vi "RealTimeSingle.vi"(0 "Digitizer Settings":T30={"Digitizer delay (us) "=0.0, "rf points per line"=2048, "lines per plane"=128, "Samp Rate (Hz)"=100000000.0, "Additional dig delay (us)"=0.0, "Voltage Scale"=0.4, "Pre-Looks"=0, "Offset delay (us)"=0.0, "bits A/D"=8, "Avg Num"=1, "DigTimeOut"=5.0, "Rel Dig Delay"=0.0, "Dig Ch"=0, "LeCroyCluster"={"LeCroy Channels"=[TRUE, FALSE, FALSE, FALSE], "LC read pt offset"=0.0, "Sweep Avg"=FALSE}, "Main Digitizer"=enum."NI Digitizer", "Dig Config"=enum."Single channel", "Digitizer ID Cluster"={"Acqiris/Alazar/SP ID"=[], "NI Instr Handles"=[], "LeCroy VISA"="", "GaGe Handle"={"Handle"=0, "Sample size"=0, "Resolution"=0, "Offset"=0, "Channels"=0, "Boards"=0}, "ATS Ref"="ATS9350", "Acqiris Address"=["PCI::INSTR0"], "ADQRef"=refnum, "adq_cu_ptr"=refnum}, "Trigger Settings"={"Trig Source"=1, "Trig Coupling"=0, "Trig Slope"=0, "Level (mV)"=1500.0}, "Bulk Acq"=FALSE, "Bulk Start Indexes"=[], "Data Ref RF"=refnum, "NI ID/Channel"=[], "Total Dig CH"=1, "Xtra Ann Trig delay (us)"=10.0, "Fix Z Delay?"=FALSE, "One Way Transmission?"=FALSE, "Data Ref Log"=refnum} {"Trigger Settings"."Trig Slope" items=["Positive", "Negative"]; "Trigger Settings"."Level (mV)" format="%.2f"; "Trigger Settings"."Trig Coupling" items=["DC 1 MOhm", "AC 1 MOhm", "DC 50 Ohm", "AC 50 Ohm"]; "Trigger Settings"."Trig Source" items=["Chan 1", "External"]; "Rel Dig Delay" format="%.2f"; "DigTimeOut" format="%.2f"; "Avg Num" min=1; "Offset delay (us)" format="%.2f"; "Additional dig delay (us)" format="%.2f"; "Digitizer delay (us)" format="%.2f"}, 1 "File Name":string="Case", 4 "Motion Settings":T26={"No Motion?"=FALSE, "Motion System"=enum."NI 735x", "Motion Bd ID"=1, "Motion Profile"="SMAC1", "# Axis"=1, "Reverse Z axis?"=TRUE, "SMAC Axis"=0, "scan pair"=enum."y-(x) scan", "RT fps"=6.0, "Steps per mm"=[1000, 1000, 1000, 1000], "Motor Parameters"={"velocity ct/s"=[10000.0, 10000.0, 10000.0, 50000.0], "accel ct/s^2"=[50000.0, 50000.0, 50000.0, 200000.0]}, "One Way Scan"=FALSE, "Reverse One Way Scan"=FALSE, "Global Position (mm)"=[], "Plane"=0, "Distance between\nscan lines (um)"=0.0, "Distance between\nscan planes (um)"=0.0, "number of scan planes"=1, "Total steps in line"=0, "Xtra plane\ndistance  (um)"=100, "Xtra planes "=1, "Add Axis"=FALSE, "overshoot cts"=200, "BKPT Shift"=0, "Scan Start Time (ms)"=0, "ESP VISA"="GPIB::1::INSTR", "3rd Axis"=1, "GL Ref Out"=refnum, "Galil Address"=""} {"3rd Axis" items=["x", "y", "z", "w"]; "Xtra planes" min=1; "Xtra plane\ndistance  (um)" min=0; "Distance between\nscan planes (um)" format="%.2f"; "Distance between\nscan lines (um)" format="%.2f"; "SMAC Axis" items=["None"=0, "Axis 1"=1, "Axis 2"=2, "Axis 3"=3, "Axis 4"=4, "Axis 5"=5, "Axis 6"=6, "Axis 7"=7, "Axis 8"=8, "Vector Space 1"=17, "Vector Space 2"=18, "Vector Space 3"=19, "Vector Space 4"=20]; "Motion Bd ID" min=1 max=32 step=1}, 5 "Type of scan":T21=enum."1-D B Scan", 6 "Ann Array Params":T22={"Synth Foc?"=FALSE, "Focal Zones"=41, "Switch T/R"=0, "Trans Geometry (mm)"={"Transducer"=0, "Geo Focus"=12.0, "a (radius)"=3.0, "# of rings"=5, "kerf space "=0.1, "Center Freq"=12.0}, "Sub Ap Excite?"=FALSE, "Full Array Scan?"=FALSE, "Xmt/Rcv"={"XMIT"=[TRUE, TRUE, TRUE, TRUE, TRUE], "RCV"=[TRUE, TRUE, TRUE, TRUE, TRUE]}, "PulseSpacing (us)"=0.0, "Xmit Ring"=0, "XMIT CHS"=0, "RCV CHS"=0, "GPU?"=FALSE, "Save TIFF?"=FALSE, "downfactor"=1, "RCV 1CH"=0} {"RCV 1CH" items=["All", "1", "2", "3", "4", "5"]; "Trans Geometry (mm)"."Transducer" items=["6D 12R 40 MHz"=0, "10D 31R 20 MHz"=1, "10D 23R 20 MHz"=2, "6D 23R 40 MHz"=3, "4.5D 10.7R 40 MHz"=4, "9D 23.5R 20 MHz"=5, "9D 25.8R 20MHz"=6, "Enter"=99]; "Switch T/R" min=1 max=5 step=1}, 7 "return to start":bool, 9 "Dual XDCR Settings":T1 {"XDCR Settings"."UT340 Controls"."Low Pass Filter (MHz)" min=-6 max=60 step=1; "XDCR Settings"."UT340 Controls"."High Pass Filter (MHz)" min=1 max=20 step=1; "XDCR Settings"."UT340 Controls"."Rep Rate (Hz)" min=20 step=1; "XDCR Settings"."UT340 Controls"."Pulse Width (ns)" min=100.0 max=250.0 step=2.0; "XDCR Settings"."UT340 Controls"."Voltage" min=100 max=250 step=2; "XDCR Settings"."UT340 Controls"."PC Gain (dB)" min=2 max=72; "XDCR Settings"."UT340 Controls"."PE Gain (dB)" min=-6 max=60 step=1; "XDCR Settings"."JSR Complete"."JSR Trigger Settings"."PRF (Hz)" items=["100 Hz"=0.1, "200 Hz"=0.2, "400 Hz"=0.4, "600 Hz"=0.6, "800 Hz"=0.8, "1000 Hz"=1.0, "1250 Hz"=1.25, "1500 Hz"=1.5, "1750 Hz"=1.75, "2000 Hz"=2.0, "2500 Hz"=2.5, "3000 Hz"=3.0, "3500 Hz"=3.5, "4000 Hz"=4.0, "4500 Hz"=4.5, "5000 Hz"=5.0]; "XDCR Settings"."JSR Complete"."JSR Trigger Settings"."Trigger Source" items=["Internal", "External"]; "XDCR Settings"."JSR Complete"."JSR Trigger Settings"."External Trigger Limit" items=["No Limit", "5 kHz"]; "XDCR Settings"."JSR Complete"."JSR Receive Settings"."Gain (dB)" min=-13 max=66 step=1; "XDCR Settings"."JSR Complete"."JSR Receive Settings"."Low Pass Filter" items=["5 MHz"=5, "10 MHz"=10, "15 MHz"=15, "22.5 MHz"=22, "35 MHz"=35, "50 MHz"=50]; "XDCR Settings"."JSR Complete"."JSR Receive Settings"."High Pass Filter" items=["DC"=0, "1 MHz"=1000, "2.5 MHz"=2500, "5 MHz"=5000, "7.5 MHz"=7500, "12.5 MHz"=12500]; "XDCR Settings"."JSR Complete"."JSR Receive Settings"."Receiver Mode" items=["Echo", "Through"]; "XDCR Settings"."JSR Complete"."JSR Pulse Settings"."Pulser Voltage (V)" items=["100"=100, "125"=125, "150"=150, "175"=175, "200"=200, "225"=225, "250"=250, "275"=275, "300"=300, "325"=325, "350"=350, "375"=375, "400"=400, "425"=425, "450"=450, "475"=475]; "XDCR Settings"."JSR Complete"."JSR Pulse Settings"."Pulser Impedance" items=["High z", "Low z"]; "XDCR Settings"."JSR Complete"."JSR Pulse Settings"."Pulse Energy Level" items=["0 (Minimum)", "1", "2", "3 (Maximum)"]; "XDCR Settings"."JSR Complete"."JSR Pulse Settings"."Damping" items=["331 Ohms"=331, "198 Ohms"=198, "142 Ohms"=142, "110 Ohms"=110, "92 Ohms"=92, "77 Ohms"=77, "67 Ohms"=67, "59 Ohms"=59, "52 Ohms"=52, "47 Ohms"=47, "43 Ohms"=43, "39 Ohms"=39, "37 Ohms"=37, "34 Ohms"=34, "32 Ohms"=32, "30 Ohms"=30]; "XDCR Settings"."Panametrics Settings"."FINE ATTENUATION" items=["00.0", "00.5", "01.0", "01.5", "02.0", "02.5", "03.0", "03.5", "04.0", "04.5", "05.0", "05.5", "06.0", "06.5", "07.0", "07.5", "08.0", "08.5", "09.0", "09.5", "10.0", "10.5", "11.0", "11.5", "12.0", "12.5", "13.0", "13.5", "14.0", "14.5", "15.0", "15.5"]; "XDCR Settings"."Panametrics Settings"."COARSE ATTENUATION" items=["00.0", "10.0", "20.0", "30.0", "40.0", "50.0"]; "XDCR Settings"."Panametrics Settings"."GAIN (db)" items=["26.0", "40.0", "54.0"]; "XDCR Settings"."Panametrics Settings"."PRF (KHz)" items=["XREMT", "EXBNC", "0.200", "0.500", "1.000", "2.000", "5.000", "10.00", "20.00"]; "XDCR Settings"."Panametrics Settings"."MODE" items=["P/ E", "THRU", "RPP", "EXT_PLSR"]; "XDCR Settings"."Panametrics Settings"."LP FILT (MHz)" items=["20", "50", "100", "200"]; "XDCR Settings"."Panametrics Settings"."HP FILT (KHz)" items=["1", "1000", "3000", "10000"]; "XDCR Settings"."Panametrics Settings"."DAMPING (Ohm)" items=["7", "10", "16", "20", "26", "30", "40", "50"]; "XDCR Settings"."Panametrics Settings"."ENERGY (uJ)" items=["1", "2", "4", "8", "16", "32"]; "XDCR Settings"."Daxsonics Settings"."Freq (MHz)" items=["4"=4, "5"=5, "6"=6, "8"=8, "10"=10, "12"=12, "14"=14, "15"=15, "16"=16, "17"=17, "18"=18, "20"=20, "25"=25, "30"=30, "35"=35, "40"=40, "45"=45, "50"=50]; "XDCR Settings"."Daxsonics Settings"."Voltage (V)" items=["0"=0, "5"=5, "10"=10, "15"=15, "20"=20, "25"=25, "30"=30, "35"=35, "40"=40, "45"=45, "50"=50, "55"=55, "60"=60, "65"=65, "70"=70, "75"=75, "80"=80, "85"=85, "90"=90, "95"=95, "100"=100, "110"=110, "120"=120, "130"=130, "140"=140, "150"=150, "160"=160, "170"=170, "180"=180, "190"=190]; "XDCR Settings"."Daxsonics Settings"."Gain (dB)" items=["22"=22, "25"=25, "28"=28, "31"=31, "34"=34, "37"=37, "40"=40, "43"=43, "46"=46, "49"=49, "52"=52, "55"=55, "58"=58, "61"=61, "64"=64, "67"=67]; "XDCR Settings"."Digitizer Settings"."Additional dig delay (ms)" format="%.2f"; "XDCR Settings"."Digitizer Settings"."Time scale per Div" items=["100 ns"=0.1, "200 ns"=0.2, "500 ns"=0.5, "1 micros"=1.0, "2 micros"=2.0, "5 micros"=5.0, "10 micros"=10.0, "20 micros"=20.0, "50 micros"=50.0, "100 micros"=100.0, "200 micros"=200.0, "500 micros"=500.0, "1 ms"=1000.0, "2 ms"=2000.0, "5 ms"=5000.0, "10 ms"=10000.0, "20 ms"=20000.0, "50 ms"=50000.0, "100 ms"=100000.0, "200 ms"=200000.0]; "XDCR Settings"."Digitizer Settings"."RF data Sampling"."rf points per line" min=1; "XDCR Settings"."Digitizer Settings"."RF data Sampling"."Ref Delay (ms)" format="%.2f"}) -> (11 "Dual XDCR Settings Out":T1 {"XDCR Settings"."UT340 Controls"."Low Pass Filter (MHz)" min=-6 max=60 step=1; "XDCR Settings"."UT340 Controls"."High Pass Filter (MHz)" min=1 max=20 step=1; "XDCR Settings"."UT340 Controls"."Rep Rate (Hz)" min=20 step=1; "XDCR Settings"."UT340 Controls"."Pulse Width (ns)" min=100.0 max=250.0 step=2.0; "XDCR Settings"."UT340 Controls"."Voltage" min=100 max=250 step=2; "XDCR Settings"."UT340 Controls"."PC Gain (dB)" min=2 max=72; "XDCR Settings"."UT340 Controls"."PE Gain (dB)" min=-6 max=60 step=1; "XDCR Settings"."JSR Complete"."JSR Trigger Settings"."PRF (Hz)" items=["100 Hz"=0.1, "200 Hz"=0.2, "400 Hz"=0.4, "600 Hz"=0.6, "800 Hz"=0.8, "1000 Hz"=1.0, "1250 Hz"=1.25, "1500 Hz"=1.5, "1750 Hz"=1.75, "2000 Hz"=2.0, "2500 Hz"=2.5, "3000 Hz"=3.0, "3500 Hz"=3.5, "4000 Hz"=4.0, "4500 Hz"=4.5, "5000 Hz"=5.0]; "XDCR Settings"."JSR Complete"."JSR Trigger Settings"."Trigger Source" items=["Internal", "External"]; "XDCR Settings"."JSR Complete"."JSR Trigger Settings"."External Trigger Limit" items=["No Limit", "5 kHz"]; "XDCR Settings"."JSR Complete"."JSR Receive Settings"."Gain (dB)" min=-13 max=66 step=1; "XDCR Settings"."JSR Complete"."JSR Receive Settings"."Low Pass Filter" items=["5 MHz"=5, "10 MHz"=10, "15 MHz"=15, "22.5 MHz"=22, "35 MHz"=35, "50 MHz"=50]; "XDCR Settings"."JSR Complete"."JSR Receive Settings"."High Pass Filter" items=["DC"=0, "1 MHz"=1000, "2.5 MHz"=2500, "5 MHz"=5000, "7.5 MHz"=7500, "12.5 MHz"=12500]; "XDCR Settings"."JSR Complete"."JSR Receive Settings"."Receiver Mode" items=["Echo", "Through"]; "XDCR Settings"."JSR Complete"."JSR Pulse Settings"."Pulser Voltage (V)" items=["100"=100, "125"=125, "150"=150, "175"=175, "200"=200, "225"=225, "250"=250, "275"=275, "300"=300, "325"=325, "350"=350, "375"=375, "400"=400, "425"=425, "450"=450, "475"=475]; "XDCR Settings"."JSR Complete"."JSR Pulse Settings"."Pulser Impedance" items=["High z", "Low z"]; "XDCR Settings"."JSR Complete"."JSR Pulse Settings"."Pulse Energy Level" items=["0 (Minimum)", "1", "2", "3 (Maximum)"]; "XDCR Settings"."JSR Complete"."JSR Pulse Settings"."Damping" items=["331 Ohms"=331, "198 Ohms"=198, "142 Ohms"=142, "110 Ohms"=110, "92 Ohms"=92, "77 Ohms"=77, "67 Ohms"=67, "59 Ohms"=59, "52 Ohms"=52, "47 Ohms"=47, "43 Ohms"=43, "39 Ohms"=39, "37 Ohms"=37, "34 Ohms"=34, "32 Ohms"=32, "30 Ohms"=30]; "XDCR Settings"."Panametrics Settings"."FINE ATTENUATION" items=["00.0", "00.5", "01.0", "01.5", "02.0", "02.5", "03.0", "03.5", "04.0", "04.5", "05.0", "05.5", "06.0", "06.5", "07.0", "07.5", "08.0", "08.5", "09.0", "09.5", "10.0", "10.5", "11.0", "11.5", "12.0", "12.5", "13.0", "13.5", "14.0", "14.5", "15.0", "15.5"]; "XDCR Settings"."Panametrics Settings"."COARSE ATTENUATION" items=["00.0", "10.0", "20.0", "30.0", "40.0", "50.0"]; "XDCR Settings"."Panametrics Settings"."GAIN (db)" items=["26.0", "40.0", "54.0"]; "XDCR Settings"."Panametrics Settings"."PRF (KHz)" items=["XREMT", "EXBNC", "0.200", "0.500", "1.000", "2.000", "5.000", "10.00", "20.00"]; "XDCR Settings"."Panametrics Settings"."MODE" items=["P/ E", "THRU", "RPP", "EXT_PLSR"]; "XDCR Settings"."Panametrics Settings"."LP FILT (MHz)" items=["20", "50", "100", "200"]; "XDCR Settings"."Panametrics Settings"."HP FILT (KHz)" items=["1", "1000", "3000", "10000"]; "XDCR Settings"."Panametrics Settings"."DAMPING (Ohm)" items=["7", "10", "16", "20", "26", "30", "40", "50"]; "XDCR Settings"."Panametrics Settings"."ENERGY (uJ)" items=["1", "2", "4", "8", "16", "32"]; "XDCR Settings"."Daxsonics Settings"."Freq (MHz)" items=["4"=4, "5"=5, "6"=6, "8"=8, "10"=10, "12"=12, "14"=14, "15"=15, "16"=16, "17"=17, "18"=18, "20"=20, "25"=25, "30"=30, "35"=35, "40"=40, "45"=45, "50"=50]; "XDCR Settings"."Daxsonics Settings"."Voltage (V)" items=["0"=0, "5"=5, "10"=10, "15"=15, "20"=20, "25"=25, "30"=30, "35"=35, "40"=40, "45"=45, "50"=50, "55"=55, "60"=60, "65"=65, "70"=70, "75"=75, "80"=80, "85"=85, "90"=90, "95"=95, "100"=100, "110"=110, "120"=120, "130"=130, "140"=140, "150"=150, "160"=160, "170"=170, "180"=180, "190"=190]; "XDCR Settings"."Daxsonics Settings"."Gain (dB)" items=["22"=22, "25"=25, "28"=28, "31"=31, "34"=34, "37"=37, "40"=40, "43"=43, "46"=46, "49"=49, "52"=52, "55"=55, "58"=58, "61"=61, "64"=64, "67"=67]; "XDCR Settings"."Digitizer Settings"."Additional dig delay (ms)" format="%.2f"; "XDCR Settings"."Digitizer Settings"."Time scale per Div" items=["100 ns"=0.1, "200 ns"=0.2, "500 ns"=0.5, "1 micros"=1.0, "2 micros"=2.0, "5 micros"=5.0, "10 micros"=10.0, "20 micros"=20.0, "50 micros"=50.0, "100 micros"=100.0, "200 micros"=200.0, "500 micros"=500.0, "1 ms"=1000.0, "2 ms"=2000.0, "5 ms"=5000.0, "10 ms"=10000.0, "20 ms"=20000.0, "50 ms"=50000.0, "100 ms"=100000.0, "200 ms"=200000.0]; "XDCR Settings"."Digitizer Settings"."RF data Sampling"."rf points per line" min=1; "XDCR Settings"."Digitizer Settings"."RF data Sampling"."Ref Delay (ms)" format="%.2f"}, 12 "Ann Array Params Out":T22={"Synth Foc?"=FALSE, "Focal Zones"=41, "Switch T/R"=0, "Trans Geometry (mm)"={"Transducer"=0, "Geo Focus"=12.0, "a (radius)"=3.0, "# of rings"=5, "kerf space "=0.1, "Center Freq"=12.0}, "Sub Ap Excite?"=FALSE, "Full Array Scan?"=FALSE, "Xmt/Rcv"={"XMIT"=[TRUE, TRUE, TRUE, TRUE, TRUE], "RCV"=[TRUE, TRUE, TRUE, TRUE, TRUE]}, "PulseSpacing (us)"=0.0, "Xmit Ring"=0, "XMIT CHS"=0, "RCV CHS"=0, "GPU?"=FALSE, "Save TIFF?"=FALSE, "downfactor"=1, "RCV 1CH"=0} {"RCV 1CH" items=["All", "1", "2", "3", "4", "5"]; "Trans Geometry (mm)"."Transducer" items=["6D 12R 40 MHz"=0, "10D 31R 20 MHz"=1, "10D 23R 20 MHz"=2, "6D 23R 40 MHz"=3, "4.5D 10.7R 40 MHz"=4, "9D 23.5R 20 MHz"=5, "9D 25.8R 20MHz"=6, "Enter"=99]; "Switch T/R" min=1 max=5 step=1}, 13 "Dual XDCR Mode":T25(ring), 14 "Digitizer Settings Out":T30={"Digitizer delay (us) "=0.0, "rf points per line"=2048, "lines per plane"=128, "Samp Rate (Hz)"=100000000.0, "Additional dig delay (us)"=0.0, "Voltage Scale"=0.4, "Pre-Looks"=0, "Offset delay (us)"=0.0, "bits A/D"=8, "Avg Num"=1, "DigTimeOut"=5.0, "Rel Dig Delay"=0.0, "Dig Ch"=0, "LeCroyCluster"={"LeCroy Channels"=[TRUE, FALSE, FALSE, FALSE], "LC read pt offset"=0.0, "Sweep Avg"=FALSE}, "Main Digitizer"=enum."NI Digitizer", "Dig Config"=enum."Single channel", "Digitizer ID Cluster"={"Acqiris/Alazar/SP ID"=[], "NI Instr Handles"=[], "LeCroy VISA"="", "GaGe Handle"={"Handle"=0, "Sample size"=0, "Resolution"=0, "Offset"=0, "Channels"=0, "Boards"=0}, "ATS Ref"="ATS9350", "Acqiris Address"=["PCI::INSTR0"], "ADQRef"=refnum, "adq_cu_ptr"=refnum}, "Trigger Settings"={"Trig Source"=1, "Trig Coupling"=0, "Trig Slope"=0, "Level (mV)"=1500.0}, "Bulk Acq"=FALSE, "Bulk Start Indexes"=[], "Data Ref RF"=refnum, "NI ID/Channel"=[], "Total Dig CH"=1, "Xtra Ann Trig delay (us)"=10.0, "Fix Z Delay?"=FALSE, "One Way Transmission?"=FALSE, "Data Ref Log"=refnum} {"Trigger Settings"."Trig Slope" items=["Positive", "Negative"]; "Trigger Settings"."Level (mV)" format="%.2f"; "Trigger Settings"."Trig Coupling" items=["DC 1 MOhm", "AC 1 MOhm", "DC 50 Ohm", "AC 50 Ohm"]; "Trigger Settings"."Trig Source" items=["Chan 1", "External"]; "Rel Dig Delay" format="%.2f"; "DigTimeOut" format="%.2f"; "Avg Num" min=1; "Offset delay (us)" format="%.2f"; "Additional dig delay (us)" format="%.2f"; "Digitizer delay (us)" format="%.2f"}, 15 "File Name Out":string="Case", 18 "Motion Settings Out":T26={"No Motion?"=FALSE, "Motion System"=enum."NI 735x", "Motion Bd ID"=1, "Motion Profile"="SMAC1", "# Axis"=1, "Reverse Z axis?"=TRUE, "SMAC Axis"=0, "scan pair"=enum."y-(x) scan", "RT fps"=6.0, "Steps per mm"=[1000, 1000, 1000, 1000], "Motor Parameters"={"velocity ct/s"=[10000.0, 10000.0, 10000.0, 50000.0], "accel ct/s^2"=[50000.0, 50000.0, 50000.0, 200000.0]}, "One Way Scan"=FALSE, "Reverse One Way Scan"=FALSE, "Global Position (mm)"=[], "Plane"=0, "Distance between\nscan lines (um)"=0.0, "Distance between\nscan planes (um)"=0.0, "number of scan planes"=1, "Total steps in line"=0, "Xtra plane\ndistance  (um)"=100, "Xtra planes "=1, "Add Axis"=FALSE, "overshoot cts"=200, "BKPT Shift"=0, "Scan Start Time (ms)"=0, "ESP VISA"="GPIB::1::INSTR", "3rd Axis"=1, "GL Ref Out"=refnum, "Galil Address"=""} {"3rd Axis" items=["x", "y", "z", "w"]; "Xtra planes" min=1; "Xtra plane\ndistance  (um)" min=0; "Distance between\nscan planes (um)" format="%.2f"; "Distance between\nscan lines (um)" format="%.2f"; "SMAC Axis" items=["None"=0, "Axis 1"=1, "Axis 2"=2, "Axis 3"=3, "Axis 4"=4, "Axis 5"=5, "Axis 6"=6, "Axis 7"=7, "Axis 8"=8, "Vector Space 1"=17, "Vector Space 2"=18, "Vector Space 3"=19, "Vector Space 4"=20]; "Motion Bd ID" min=1 max=32 step=1}, 19 "error out":errorcluster)   [LabVIEW 2022 SP3]
uses:
  ScanningControl/Digitizers/-DigitizerRoutines/DigitizerSettings.ctl
  ScanningControl/Digitizers/-DigitizerRoutines/Digitizer.ctl
  ScanningControl/Digitizers/-DigitizerRoutines/DigConfig.ctl
  ScanningControl/Digitizers/-DigitizerRoutines/DigitizerID.ctl
  C:/Windows/System32/ADQAPI_dotNet_helper.dll
  Windows/System32/ADQAPI_dotNet_helper.dll
  ScanningControl/Motion Controllers/NI_controller/-NI_MotionRoutines/MotionParameters.ctl
  ScanningControl/Motion Controllers/NI_controller/-NI_MotionRoutines/MotionSys.ctl
  ScanningControl/Motion Controllers/-MotionRoutines/ScanAxis.ctl
  ScanningControl/Motion Controllers/-MotionRoutines/3rdAxis.ctl
  ScanningControl/Pulsers/Daxsonics/-DaxSubroutines/Dax_Control_Cluster.ctl
  Annular Array/-AnnularRoutines/AnnularArray.ctl
  Annular Array/-AnnularRoutines/TransGeometry.ctl
  Annular Array/-AnnularRoutines/ArrayGeometry.ctl
  ScanningControl/-ScanSystem/Controls/ScanType2.ctl
  ScanningControl/DualXDCR/Dual XDCR Complete Settings.ctl
  ScanningControl/DualXDCR/XDCRSettings.ctl
  ScanningControl/Pulsers/Panametrics/Pana5900.ctl
  ScanningControl/Pulsers/JSR/Controls/JSR Complete.ctl
  ScanningControl/Pulsers/JSR/Controls/JSR Pulse.ctl
  ScanningControl/Pulsers/JSR/Controls/Damping.ctl
  ScanningControl/Pulsers/JSR/Controls/Energy.ctl
  ScanningControl/Pulsers/JSR/Controls/Z.ctl
  ScanningControl/Pulsers/JSR/Controls/Volt.ctl
  ScanningControl/Pulsers/JSR/Controls/JSR Recieve.ctl
  ScanningControl/Pulsers/JSR/Controls/Mode.ctl
  ScanningControl/Pulsers/JSR/Controls/HPF.ctl
  ScanningControl/Pulsers/JSR/Controls/LPF.ctl
  ScanningControl/Pulsers/JSR/Controls/Gain.ctl
  ScanningControl/Pulsers/JSR/Controls/JSR Trigger.ctl
  ScanningControl/Pulsers/JSR/Controls/Trig Limit.ctl
  ScanningControl/Pulsers/JSR/Controls/Trig Source.ctl
  ScanningControl/Pulsers/JSR/Controls/PRF.ctl
  ScanningControl/Pulsers/UTEX/Controls/UTEX Controls.ctl
  ScanningControl/Pulsers/JSR/Controls/JSR Simple.ctl
  ScanningControl/Pulsers/UTEX/Controls/UTEX Controls Simple.ctl
  <vilib>/Utility/miscctls.llb/LVRectTypeDef.ctl
  ScanningControl/-ScanSystem/Controls/location.ctl
  ScanningControl/Motion Controllers/Galil/Command Menu.ctl
  <vilib>/Analysis/baseanly.llb/Mean (DBL).vi
  ScanningControl/Motion Controllers/-MotionRoutines/MotionGlobals.vi
  ScanningControl/Pulsers/PulserGlobals.vi
  ScanningControl/Switch Modules/SwitchGlobals.vi
  Misc Programs/MathOperations/ModuloFractionArray.vi
  Misc Programs/MathOperations/ModuloFraction.vi
  <vilib>/Motion/FlexMotion/CustomControls/CustomControls.llb/Program.flx
  <vilib>/Motion/FlexMotion/FunctionsVIs/OnboardProgramming.llb/Pause/Resume Program.flx
  <vilib>/Motion/FlexMotion/FunctionsVIs/Trajectory.llb/Load Acceleration/Deceleration.flx
  <vilib>/ptbypt/NI_PtbyPt.lvlib
  <vilib>/Analysis/NI_AALBase.lvlib
  <vilib>/Motion/FlexMotion/FunctionsVIs/StartStopMotion.llb/Start Motion (8 axes).flx
  <vilib>/Motion/FlexMotion/FunctionsVIs/StartStopMotion.llb/Stop Motion (8 axes).flx
  <instrlib>/LeCroy Wave Series/LeCroy Wave Series.lvlib
panel:
  in  "Reset Scan":bool
  in  "Initilize":bool
  out "Total Pts":bool=TRUE
  in  "Force Symmetric?":bool
  out "Z Change":bool=TRUE
  out "FixedLinesPerPlane":i32
  out "Scan Start Pos (mm)":dbl[](array[numeric])
  in  "Transducer":u16(ring)
  in  "Delay Corr?":bool=TRUE
  out "Last End Point":dbl format="%.2f"
  out "End Point Counter":u32
  in  "Dual XDCR\nDigi Time Settings":cluster{"RF PPL":i32, "Ref Delay (us)":dbl}[](array[cluster])
  in  "FileName Gen":bool
  in  "Acquisition Volume (mm)":dbl[](array[numeric])
  in  "dB Range":cluster{dbl, dbl}(slide)={-1.5, -60.0} scale=-42.1..0.11000000000000001
  out "Found Center":bool
  in  "Fill":bool
  in  "1-to-1":bool
  in  "Scan":bool
  in  "Exit":bool
  in  "Tab Control":T34(tab)
  in  "Inc Step Size\n(mm)":dbl=1.0
  in  "Axis Tune":enum32{"Axis 1", "Axis 2", "Axis 3", "Axis 4"}(radio)=enum."Axis 2"
  in  "Position (mm)":dbl format="%.2f"
  in  "Stop Motor":bool
  in  "Pause Motion":bool caption="Pause Scanning"
  out "Frame #":i32
  out "No data":bool
  out "FPS":dbl format="%#.2g"
  in  "Position (mm) (Pt1)":dbl format="%.3f"
  in  "Position (mm) (Pt2)":dbl format="%.3f"
  in  "End Point\nMarker":bool
  in  "Center":bool
  in  "JSR Simple":T35={"Pulse Energy Level"=2, "Gain (dB)"=50, "Pulser Voltage (V)"=0} {"Pulser Voltage (V)" items=["100"=100, "125"=125, "150"=150, "175"=175, "200"=200, "225"=225, "250"=250, "275"=275, "300"=300, "325"=325, "350"=350, "375"=375, "400"=400, "425"=425, "450"=450, "475"=475]; "Gain (dB)" min=-13 max=66 step=1; "Pulse Energy Level" items=["0 (Minimum)", "1", "2", "3 (Maximum)"]}
  in  "Distance Between Planes (um)":sgl[](array[numeric])
  in  "Acquistion Parameters":T36={"Sampling Rate"=250.0, "Ref Delay (ms)"=0.0, "rf points per line"=2048, "Dig Scale"=4.0} {"Dig Scale" items=["10 V"=10.0, "4 V"=4.0, "2 V"=2.0, "1 V"=1.0, "400 mV"=0.4, "200 mV"=0.2, "100 mV"=0.1]; "rf points per line" min=1; "Ref Delay (ms)" format="%.2f"}
  in  "Motion Parameters":T37={"lines per plane"=128, "Distance between\nscan lines (um)"=100.0, "Frames/s"=2.0, "BKPT Shift"=75, "Overshoot"=200} {"Overshoot" min=0 max=10000; "Distance between\nscan lines (um)" min=0.1 step=0.1; "lines per plane" min=1}
  in  "Display mode":u16(ring)=1 items=["Linear Abs Grey", "Log Grey Scale", "Linear Color Scale", "Sector"]
  in  "SetDig":bool
  in  "UT340 Controls":T38={"PE Gain (dB)"=1, "Voltage"=100} {"Voltage" min=1 max=20 step=1; "PE Gain (dB)" min=-6 max=60 step=1}
  in  "Set Pulser":bool
  in  "Daxsonics Settings":T3={"Freq (MHz) "=20, "Voltage (V)"=0, "Gain (dB)"=22} {"Freq (MHz)" items=["3"=3, "2"=2, "1"=1, "0"=0]; "Voltage (V)" items=["66"=66, "65"=65, "64"=64, "63"=63, "62"=62, "61"=61, "60"=60, "59"=59, "58"=58, "57"=57, "56"=56, "55"=55, "54"=54, "53"=53, "52"=52, "51"=51, "50"=50, "49"=49, "48"=48, "47"=47, "46"=46, "45"=45, "44"=44, "43"=43, "42"=42, "41"=41, "40"=40, "39"=39, "38"=38, "37"=37, "36"=36, "35"=35, "34"=34, "33"=33, "32"=32, "31"=31, "30"=30, "29"=29, "28"=28, "27"=27, "26"=26, "25"=25, "24"=24, "23"=23, "22"=22, "21"=21, "20"=20, "19"=19, "18"=18, "17"=17, "16"=16, "15"=15, "14"=14, "13"=13, "12"=12, "11"=11, "10"=10, "9"=9, "8"=8, "7"=7, "6"=6, "5"=5, "4"=4, "3"=3, "2"=2, "1"=1, "0"=0, "-1"=65535, "-2"=65534, "-3"=65533, "-4"=65532, "-5"=65531, "-6"=65530, "-7"=65529, "-8"=65528, "-9"=65527, "-10"=65526, "-11"=65525, "-12"=65524, "-13"=65523]; "Gain (dB)" items=["475"=475, "450"=450, "425"=425, "400"=400, "375"=375, "350"=350, "325"=325, "300"=300, "275"=275, "250"=250, "225"=225, "200"=200, "175"=175, "150"=150, "125"=125, "100"=100]}
  in  "Panametrics Settings":T39 {"FINE ATTENUATION" items=["00.0", "00.5", "01.0", "01.5", "02.0", "02.5", "03.0", "03.5", "04.0", "04.5", "05.0", "05.5", "06.0", "06.5", "07.0", "07.5", "08.0", "08.5", "09.0", "09.5", "10.0", "10.5", "11.0", "11.5", "12.0", "12.5", "13.0", "13.5", "14.0", "14.5", "15.0", "15.5"]; "COARSE ATTENUATION" items=["00.0", "10.0", "20.0", "30.0", "40.0", "50.0"]; "ENERGY (uJ)" items=["1", "2", "4", "8", "16", "32"]}
  in  "scan pair":T28=enum."x-(y) scan"
  in  "Full Scan Size (mm)":dbl[](array[numeric])
  in  "Re-Load\nDual Transducer\nSettings":bool
  in  "Save\nDual Transducer\nSettings":bool
  in  "distance?":bool=TRUE
  in  "Type of Mean":u16(ring)=3 items=["Mean from lines", "Mean just lines", "Poly Mean", "No mean", "Filter"]
  in  "*.eye":bool
  in  "BMP?":bool
  in  "Movie Name":string="none"
  in  "Filter Prams":T40={"low cutoff"=20, "order"=81, "high cutoff"=60}
  in  "view":bool=TRUE
  in  "Pause Mode?":bool
  out "Real Time Image":dbl[][](graph)
  # "Width \n(White Lines)"
  # "Cross-Axis\nWidth"
  # "Depth\n(Blue Lines)"
  # "1-D and 2-D B scan settings"
  # "1-D and 2-D B scan settings"
  # "Manual Axis Motion"
  # "XDCR 1"
  # "XDCR 2"
  # "Click Value\nto Change"
  # "Cross-Axis\nWidth"
  # "Depth"
  # "Width"
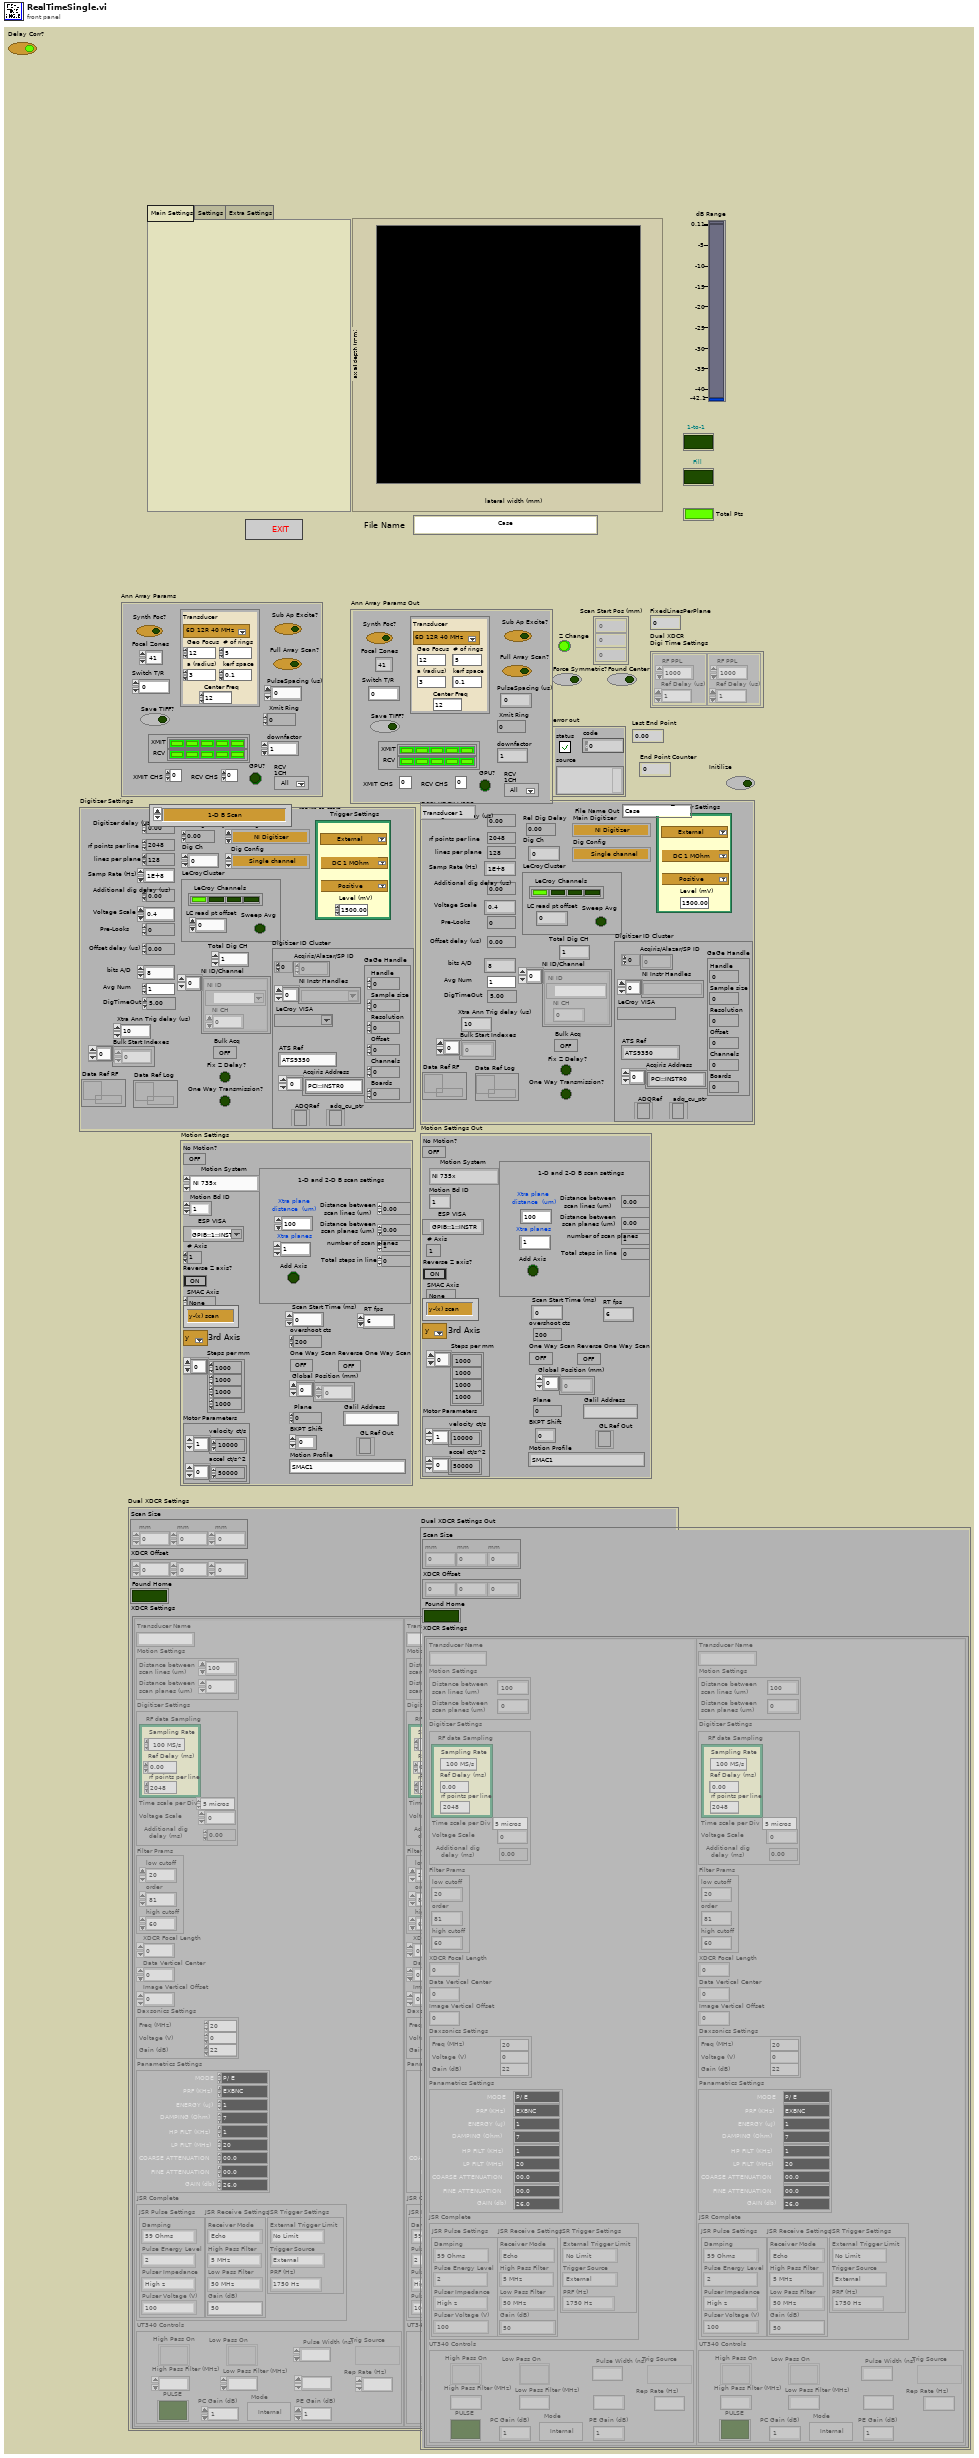
[diagram p1: front panel]
types:
  T1 = typedef "Dual XDCR Complete Settings.ctl" = cluster{"Scan Size":dbl[], "XDCR Offset":dbl[], "Found Home":bool, "XDCR Settings":T2[]}
  T2 = typedef "XDCRSettings.ctl" = cluster{"Transducer Name":string, "Motion Settings":cluster{"Distance between\nscan lines (um)":sgl, "Distance between\nscan planes (um)":sgl}, "Digitizer Settings":cluster{"RF data Sampling":cluster{"Sampling Rate":dbl, "Ref Delay (ms)":dbl, "rf points per line":i32}, "Time scale per Div":dbl, "Voltage Scale":dbl, "Additional dig delay (ms)":dbl}, "Filter Prams":cluster{"low cutoff":i32, "order":i32, "high cutoff":i32}, "XDCR Focal Length":dbl, "Data Vertical Center":dbl, "Image Vertical Offset":dbl, "Daxsonics Settings":T3, "Panametrics Settings":T4, "JSR Complete":T5, "UT340 Controls":T20}
  T3 = typedef "Dax_Control_Cluster.ctl" = cluster{"Freq (MHz) ":u16, "Voltage (V)":u16, "Gain (dB)":u16}
  T4 = typedef "Pana5900.ctl" = cluster{"ENERGY (uJ)":u16, "DAMPING (Ohm)":u16, "HP FILT (KHz) ":u16, "LP FILT (MHz)":u16, "MODE":u16, "PRF (KHz)":u16, "GAIN (db)":u16, "COARSE ATTENUATION":u16, "FINE ATTENUATION":u16}
  T5 = typedef "JSR Complete.ctl" = cluster{"JSR Pulse Settings":T6, "JSR Receive Settings":T11, "JSR Trigger Settings":T16}
  T6 = typedef "JSR Pulse.ctl" = cluster{"Damping":T7, "Pulse Energy Level":T8, "Pulser Impedance":T9, "Pulser Voltage (V)":T10}
  T7 = typedef "Damping.ctl" = i16
  T8 = typedef "Energy.ctl" = u16
  T9 = typedef "Z.ctl" = u16
  T10 = typedef "Volt.ctl" = i16
  T11 = typedef "JSR Recieve.ctl" = cluster{"Receiver Mode":T12, "High Pass Filter":T13, "Low Pass Filter":T14, "Gain (dB)":T15}
  T12 = typedef "Mode.ctl" = i8
  T13 = typedef "HPF.ctl" = u16
  T14 = typedef "LPF.ctl" = u16
  T15 = typedef "Gain.ctl" = i8
  T16 = typedef "JSR Trigger.ctl" = cluster{"External Trigger Limit":T17, "Trigger Source":T18, "PRF (Hz)":T19}
  T17 = typedef "Trig Limit.ctl" = i8
  T18 = typedef "Trig Source.ctl" = i8
  T19 = typedef "PRF.ctl" = dbl
  T20 = typedef "UTEX Controls.ctl" = cluster{"High Pass On":bool, "High Pass Filter (MHz)":i16, "Low Pass On":bool, "Low Pass Filter (MHz)":i16, "PE Gain (dB)":i16, "Voltage":i16, "Pulse Width (ns)":dbl, "Mode":bool, "PC Gain (dB)":i16, "Trig Source":bool, "Rep Rate (Hz)":i16, "PULSE":bool}
  T21 = typedef "ScanType2.ctl" = enum16{"Therapy With Scan", "M scan", "M Scan With Therapy Burst", "1-D B Scan", "1-D B Scan With Therapy Burst", "2-D B Scan", "2-D B Scan With Therapy Burst", "Rotational Scan", "1-D B-Scan PRF", "2-D B-Scan PRF", "Real-Time Scan", "Contrast Agents", "1-D w/ Real-Time Set Up", "Dual Transducer", "Acoustic Microscopy", "Hydrophone Scanning"}
  T22 = typedef "AnnularArray.ctl" = cluster{"Synth Foc?":bool, "Focal Zones":i16, "Switch T/R":i16, "Trans Geometry (mm)":T23, "Sub Ap Excite?":bool, "Full Array Scan?":bool, "Xmt/Rcv":cluster{"XMIT":bool[], "RCV":bool[]}, "PulseSpacing (us)":sgl, "Xmit Ring":i32, "XMIT CHS":u8, "RCV CHS":u8, "GPU?":bool, "Save TIFF?":bool, "downfactor":i32, "RCV 1CH":u16}
  T23 = typedef "TransGeometry.ctl" = cluster{"Transducer":T24, "Geo Focus":dbl, "a (radius)":dbl, "# of rings":i32, "kerf space ":dbl, "Center Freq":dbl}
  T24 = typedef "ArrayGeometry.ctl" = u16
  T25 = enum16{"Transducer 1", "Transducer 2", "Dual XDCR", "Exit"}
  T26 = typedef "MotionParameters.ctl" = cluster{"No Motion?":bool, "Motion System":T27, "Motion Bd ID":u8, "Motion Profile":string, "# Axis":i8, "Reverse Z axis?":bool, "SMAC Axis":u16, "scan pair":T28, "RT fps":sgl, "Steps per mm":i32[], "Motor Parameters":cluster{"velocity ct/s":dbl[], "accel ct/s^2":dbl[]}, "One Way Scan":bool, "Reverse One Way Scan":bool, "Global Position (mm)":dbl[], "Plane":i32, "Distance between\nscan lines (um)":sgl, "Distance between\nscan planes (um)":sgl, "number of scan planes":i32, "Total steps in line":i32, "Xtra plane\ndistance  (um)":i32, "Xtra planes ":i32, "Add Axis":bool, "overshoot cts":i32, "BKPT Shift":i32, "Scan Start Time (ms)":u32, "ESP VISA":refnum<visa-resource-name>, "3rd Axis":T29, "GL Ref Out":refnum<k7>, "Galil Address":string}
  T27 = typedef "MotionSys.ctl" = enum16{"MM3000", "NI 735x", "Newport ESP", "No Motion Card", "Galil"}
  T28 = typedef "ScanAxis.ctl" = enum16{"y-(x) scan", "x-(y) scan", "z-(x) scan", "z-(y) scan", "y-(z) scan", "x-(z) scan", "w-(x) scan", "w-(y) scan", "w-(z) scan", "x-(w) scan", "y-(w) scan", "z-(w) scan"}
  T29 = typedef "3rdAxis.ctl" = u16
  T30 = typedef "DigitizerSettings.ctl" = cluster{"Digitizer delay (us) ":dbl, "rf points per line":i32, "lines per plane":i32, "Samp Rate (Hz)":dbl, "Additional dig delay (us)":dbl, "Voltage Scale":dbl, "Pre-Looks":i32, "Offset delay (us)":dbl, "bits A/D":i8, "Avg Num":i32, "DigTimeOut":sgl, "Rel Dig Delay":sgl, "Dig Ch":i32, "LeCroyCluster":cluster{"LeCroy Channels":bool[], "LC read pt offset":dbl, "Sweep Avg":bool}, "Main Digitizer":T31, "Dig Config":T32, "Digitizer ID Cluster":T33, "Trigger Settings":cluster{"Trig Source":u16, "Trig Coupling":u16, "Trig Slope":u16, "Level (mV)":dbl}, "Bulk Acq":bool, "Bulk Start Indexes":i32[], "Data Ref RF":refnum<data-value>, "NI ID/Channel":cluster{"NI ID":refnum<k15>, "NI CH":i32}[], "Total Dig CH":i32, "Xtra Ann Trig delay (us)":dbl, "Fix Z Delay?":bool, "One Way Transmission?":bool, "Data Ref Log":refnum<data-value>}
  T31 = typedef "Digitizer.ctl" = enum16{"Acqiris Digitizer", "NI Digitizer", "LeCroy", "GaGe", "AlazarTech", "No Digitizer", "Teledyne"}
  T32 = typedef "DigConfig.ctl" = enum16{"Single channel", "2 Chans w/ 2 Acqiris", "2 Chans w/ 1 Acqiris", "5-CH Pulser New", "5-CH pulser w/ ann array", "5-pass style ann array", "Empty"}
  T33 = typedef "DigitizerID.ctl" = cluster{"Acqiris/Alazar/SP ID":u32[], "NI Instr Handles":refnum<k15>[], "LeCroy VISA":refnum<visa-resource-name>, "GaGe Handle":cluster{"Handle":u32, "Sample size":u32, "Resolution":i32, "Offset":i32, "Channels":u32, "Boards":u32}, "ATS Ref":string, "Acqiris Address":string[], "ADQRef":refnum<k24>, "adq_cu_ptr":refnum<k24>}
  T34 = enum32{"Main Settings", "Settings", "Extra Settings"}
  T35 = typedef "JSR Simple.ctl" = cluster{"Pulse Energy Level":T8, "Gain (dB)":T15, "Pulser Voltage (V)":T10}
  T36 = cluster{"Sampling Rate":dbl, "Ref Delay (ms)":dbl, "rf points per line":i32, "Dig Scale":dbl}
  T37 = cluster{"lines per plane":u16, "Distance between\nscan lines (um)":sgl, "Frames/s":sgl, "BKPT Shift":i32, "Overshoot":i32}
  T38 = typedef "UTEX Controls Simple.ctl" = cluster{"PE Gain (dB)":i16, "Voltage":i16}
  T39 = cluster{"ENERGY (uJ)":u16, "COARSE ATTENUATION":u16, "FINE ATTENUATION":u16}
  T40 = cluster{"low cutoff":i32, "order":i32, "high cutoff":i32}
  T41 = typedef "LVRectTypeDef.ctl" = cluster{"Left":i16, "Top":i16, "Right":i16, "Bottom":i16}
  T42 = cluster{"gain":dbl, bool, "Array":i16[][], "gain 2":dbl, bool}
  T43 = typedef "location.ctl" = enum16{"Automatic", "WCM Main", "Hawaii", "Columbia MM3000", "Columbia  NI System", "NYU", "RRI 2", "UHI Allen", "CUMC RT", "Chiba", "Stony Brook", "WCM Microscopy", "WCM Aeoretch", "WCM Optics Lab", "WCM Main 2Axis", "WCM Rotation", "WCM SAM SMAC", "SERI GP"}
  T44 = typedef "SwitchOption.ctl" = enum16{"Cytex", "Pickering", "NI Switch", "No Switch", "Riverside USB"}
  T45 = typedef "pulser.ctl" = enum16{"Pan 5900", "Daxsonics", "Agilent 33xxx", "UTEX", "JSR", "WMC Mono-Cycle", "No Pulser", "NYU AVTECH", "Tabor W1281A", "Pan 5800", "Unlisted", "Tabor WX2182B"}
  T46 = enum8{"Enabled", "Disabled", "Disabled and Grayed Out"}
  T47 = enum16{"Round to +INF", "Round Nearest", "Round to -INF"}
  T48 = enum16{"Absolute Position", "Relative Position", "Velocity", "Relative to Cap Pos", "Modulus Position", "Absolute Contouring", "Relative Contouring"}
  T49 = enum16{"Home", "Index", "Center", "Forward Limit", "Reverse Limit", "Run Sequence"}
  T50 = typedef "Command Menu.ctl" = enum16{"CommandPassThrough", "Abort Motion", "Define Pos", "Velocity", "Acceleration", "Deceleration", "Position Rel", "Postion Abs", "Begin Move", "After Move", "Home", "KI", "KD", "KP", "IL", "Config I/O", "Set Bit", "Clear Bit", "Motor Off", "Moto On", "Status", "Execute", "Halt Execute", "HX Status", "Tell Velocity", "Check Motion", "BreakPoint", "Tell Position", "Current Code Line", "Tell Switches", "OC Force On", "OC Off", "Pos Soft Limit", "Rev Soft Limit"}
  T51 = cluster{"Voltage Scale":dbl, "Offset":dbl, "Coupling":u16}
  T52 = typedef "Program.flx" = u8
  T53 = enum16{"Left Button", "Center Button", "Right Button", "Window Close"}
  T54 = typedef "Bd Id Out" = u8
  T55 = cluster{"velocity ct/s":dbl[], "accel ct/s^2":dbl[]}
  T56 = typedef "Resource Out (Enum).flx" = u16
  T57 = typedef "AxisOrVectorSpaceControl To Control.flx" = u16
  T58 = typedef "GL Axis Control.ctl" = u16
  T59 = typedef "LVStringsAndValuesArrayTypeDef_DBL.ctl" = cluster{"String":string, "Value":dbl}[]
  T60 = cluster{"Samp Rate (Hz)":dbl, "Digitizer delay (us) ":dbl, "rf points per line":i32, "Voltage Scale":dbl}
  T61 = cluster{"lines per plane":i32, "Distance between\nscan lines (um)":sgl, "RT fps":sgl, "BKPT Shift":i32, "overshoot cts":i32}
  T62 = cluster{"FIR Windowed Coefficients":dbl[], "Filter Prams":cluster{"low cutoff":i32, "order":i32, "high cutoff":i32}}
  T63 = cluster{"Trig Source":u16, "Trig Coupling":u16, "Trig Slope":u16, "Level (mV)":dbl}
  T64 = cluster{"data value reference":refnum<data-value>, "bytes to transfer":u32, "rf pts actual":u32}
  T65 = typedef "imagedata.ctl" = cluster{"image type":i32, "image depth":i32, "image":u8[], "mask":u8[], "colors":u32[], "Rectangle":cluster{"left":i16, "top":i16, "right":i16, "bottom":i16}}
  T66 = cluster{"Y Scale Offset":dbl, "Y Scale Multi":dbl, "X Scale Offset":dbl, "X Scale Multi":dbl, "Gate Distance":dbl}
  T67 = typedef "LVBoundsTypeDef.ctl" = cluster{"Width":u32, "Height":u32}
  T68 = typedef "eventvkey.ctl" = enum16{"ASCII", "Enter", "Return", "Shift", "Ctrl", "Alt", "Cmd", "Opt", "Caps", "NumLock", "Clear", "Break", "Up", "Down", "Left", "Right", "Insert", "Delete", "Home", "End", "PageUp", "PageDown", "Escape", "Help", "Pause", "ScrollLock", "F1", "F2", "F3", "F4", "F5", "F6", "F7", "F8", "F9", "F10", "F11", "F12", "F13", "F14", "F15", "F16", "F17", "F18", "F19", "F20", "F21", "F22", "F23", "F24", "Play", "VolumeUp", "VolumeDown", "Mute", "Two Byte Char"}
  T69 = cluster{"Shift":bool, "Ctrl":bool, "Alt":bool, "Cmd":bool, "Opt":bool}
  T70 = typedef "LVRangeTypeDef.ctl" = cluster{"Minimum":dbl, "Maximum":dbl, "Increment":dbl, "Minor Increment":dbl, "Start":dbl}
  T71 = cluster{"gain":dbl, bool, "Array out":i16[][], "gain 2 Ch":dbl, "dig error":bool}
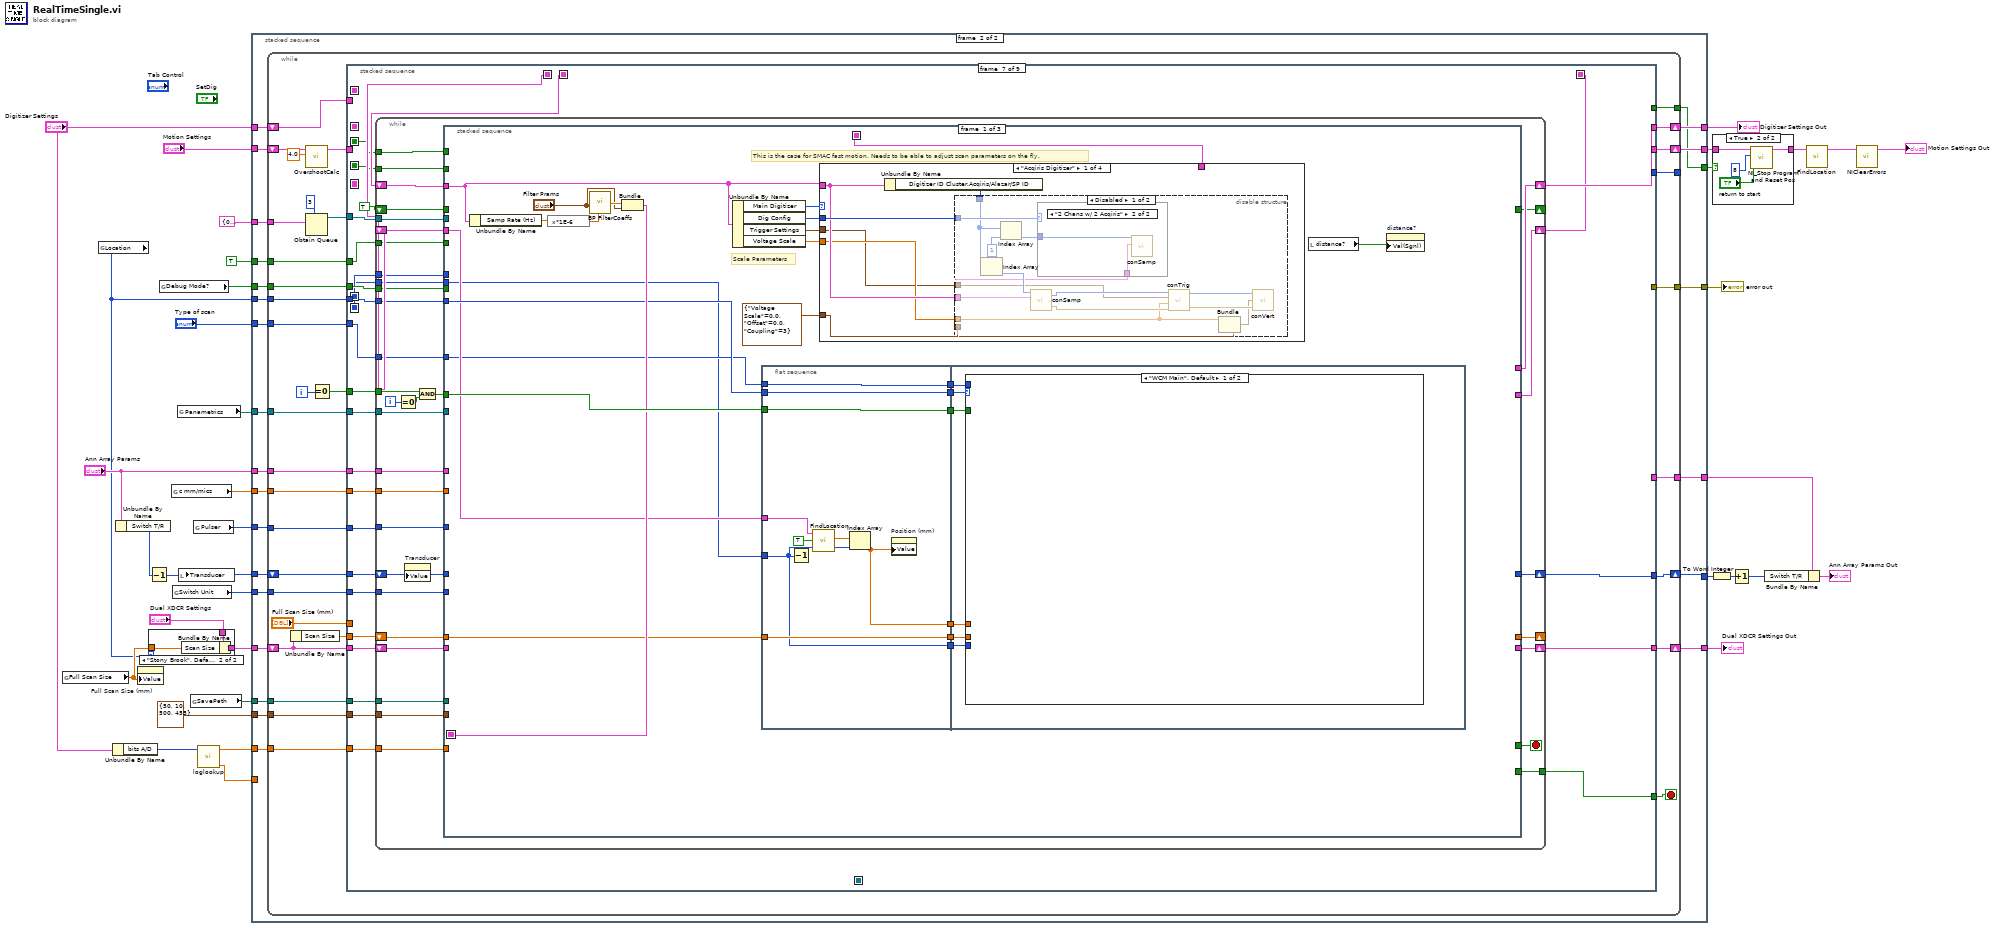
[diagram p0: block diagram]
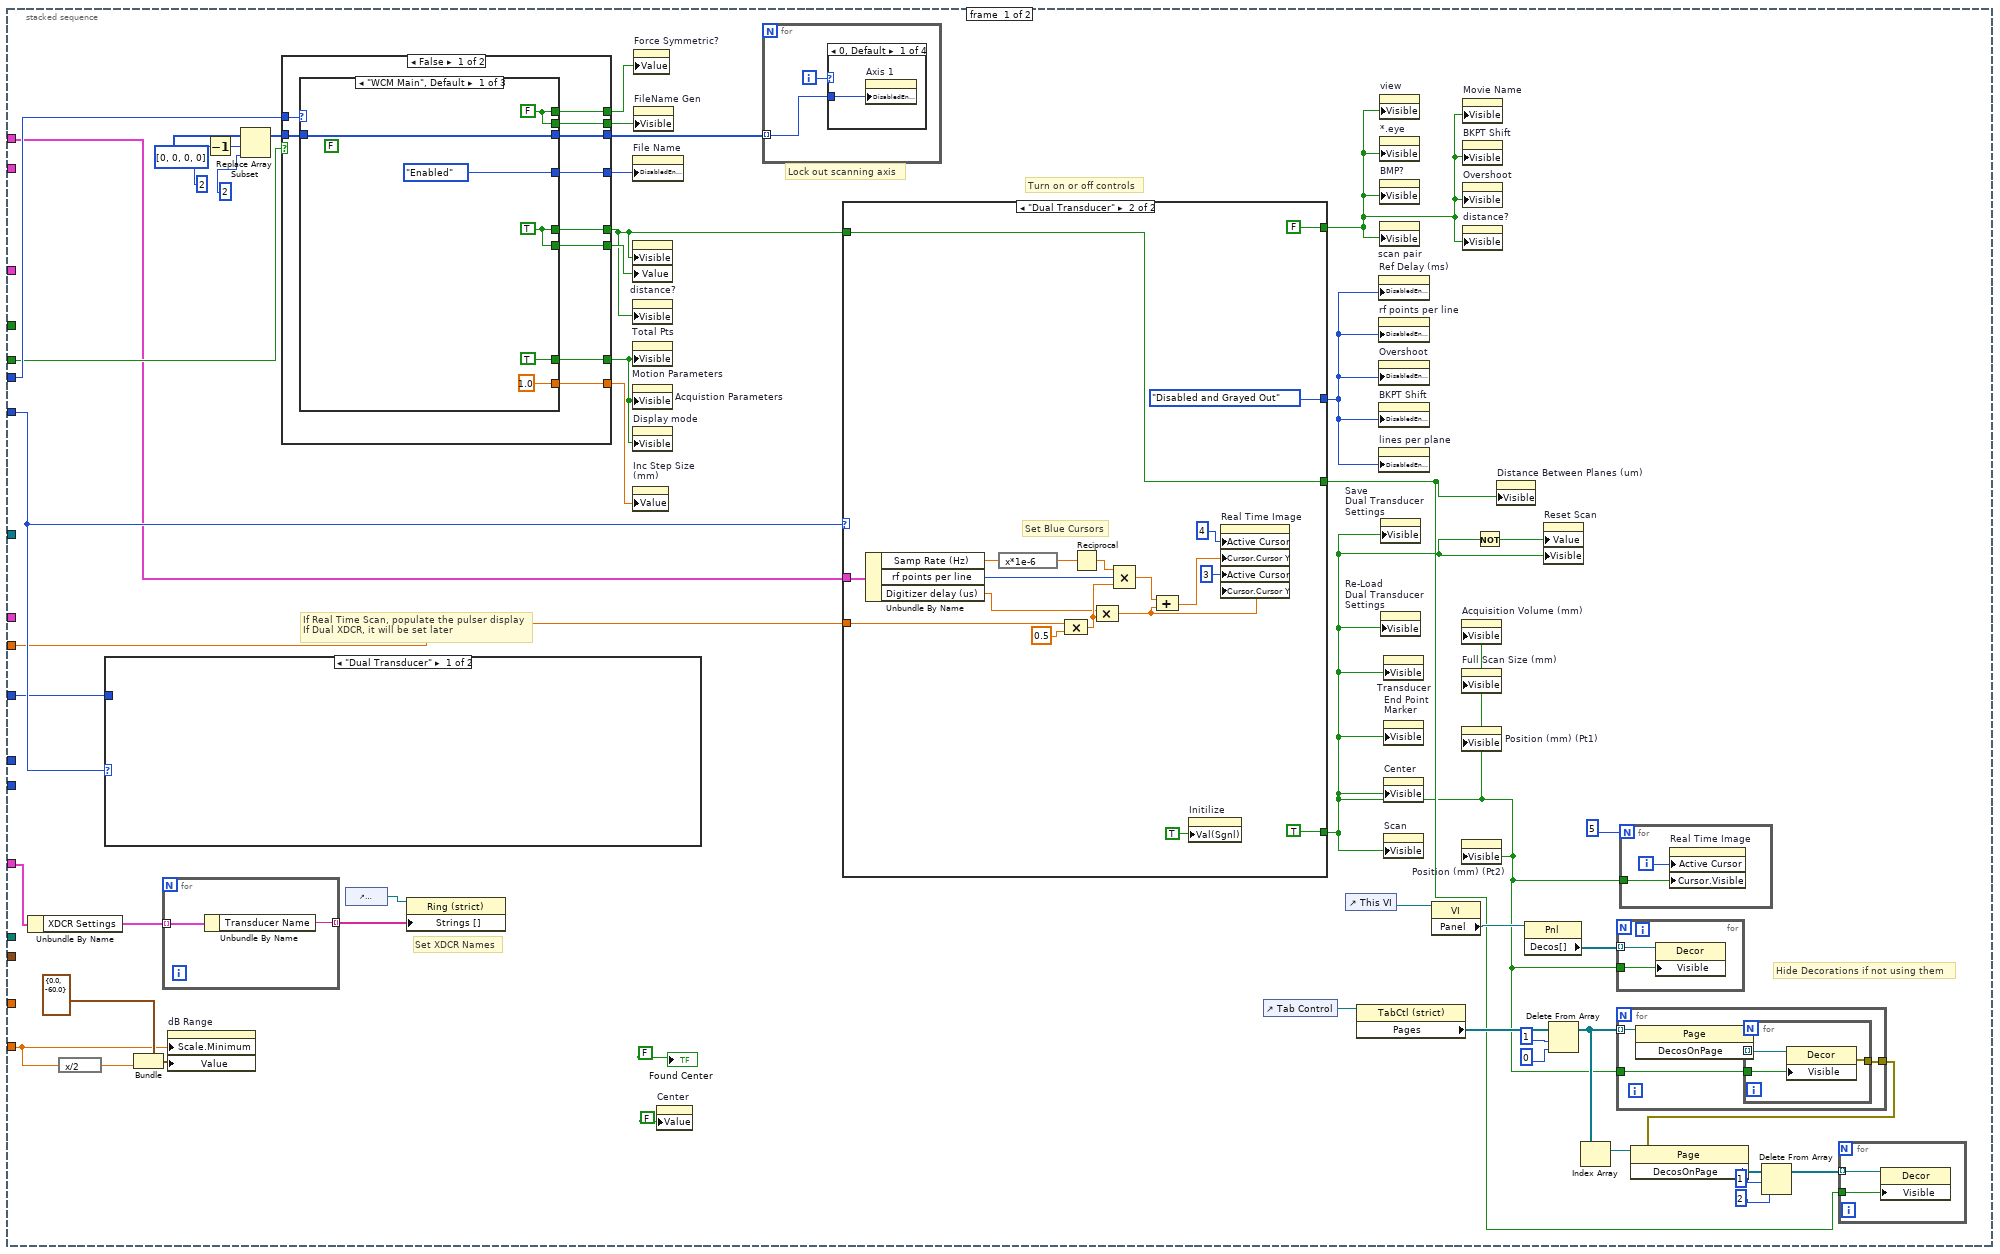
[diagram p2: hidden frame]
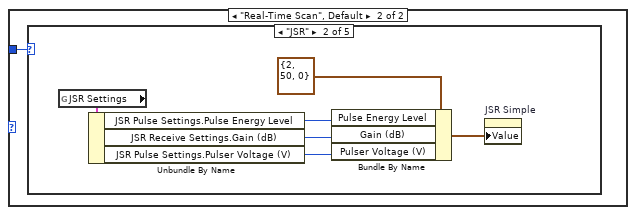
[diagram p3: hidden frame]
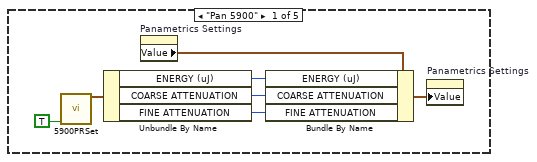
[diagram p4: hidden frame]
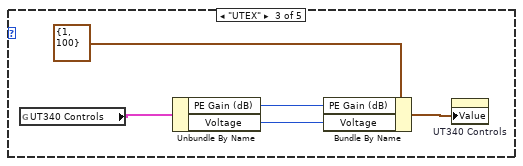
[diagram p5: hidden frame]
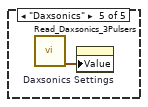
[diagram p7: hidden frame]
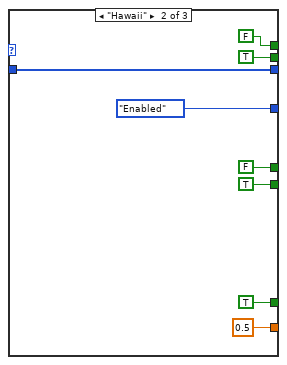
[diagram p8: hidden frame]
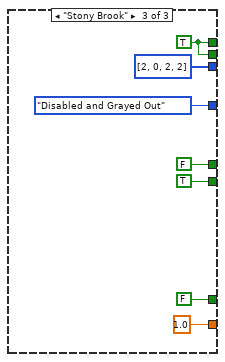
[diagram p9: hidden frame]
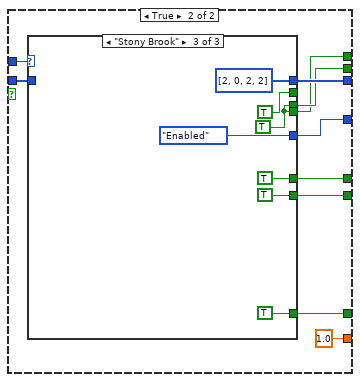
[diagram p10: hidden frame]
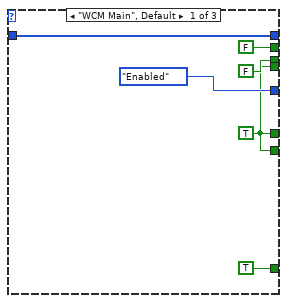
[diagram p11: hidden frame]
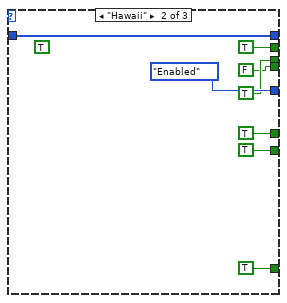
[diagram p12: hidden frame]
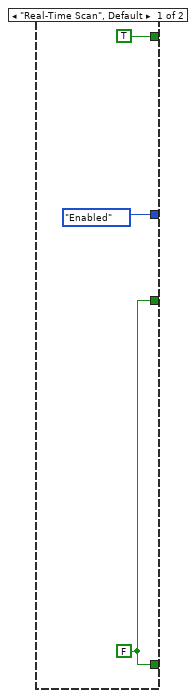
[diagram p13: hidden frame]
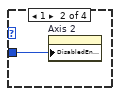
[diagram p14: hidden frame]
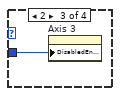
[diagram p15: hidden frame]
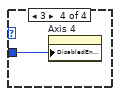
[diagram p16: hidden frame]
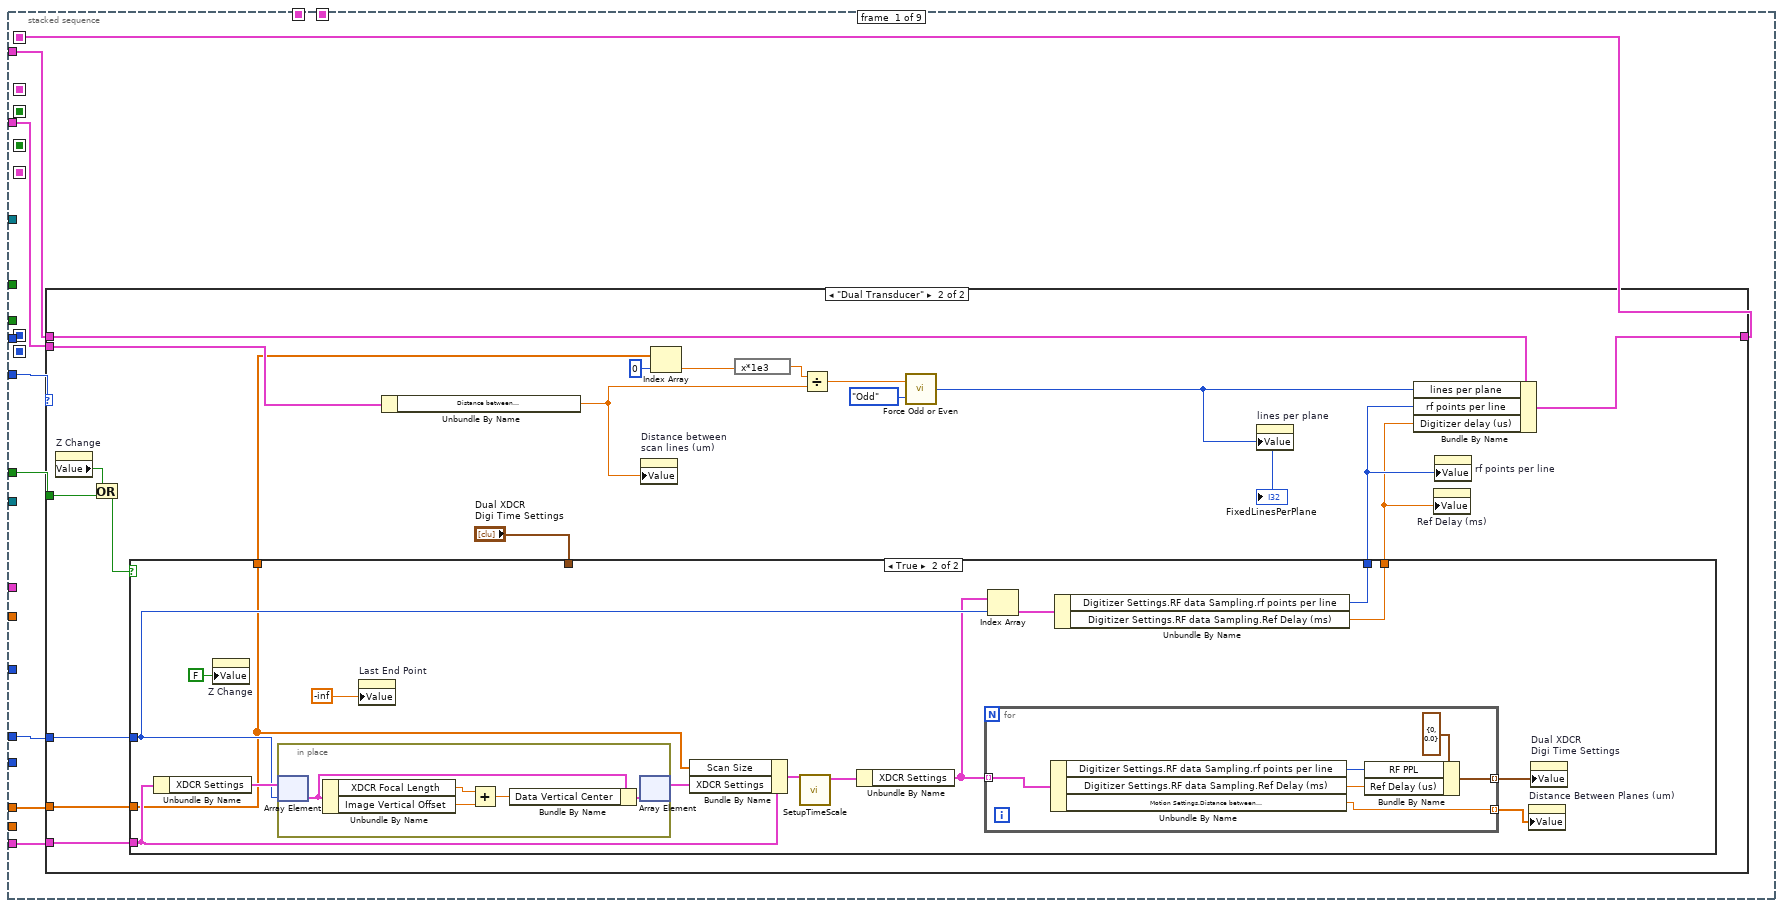
[diagram p17: hidden frame]
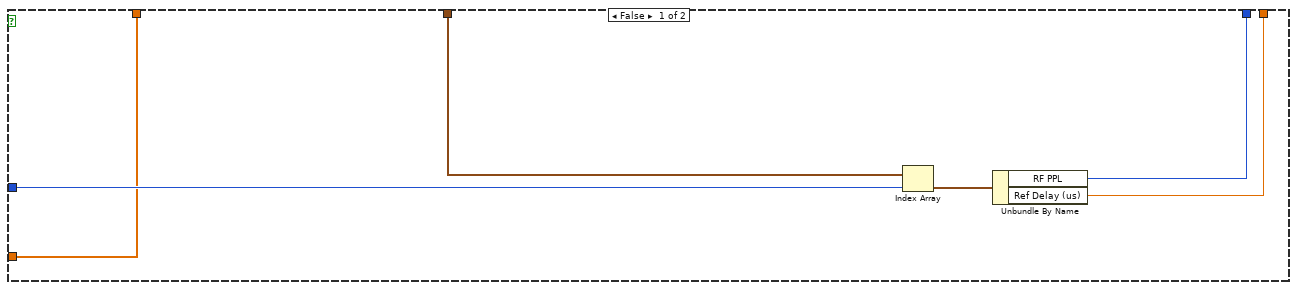
[diagram p19: hidden frame]
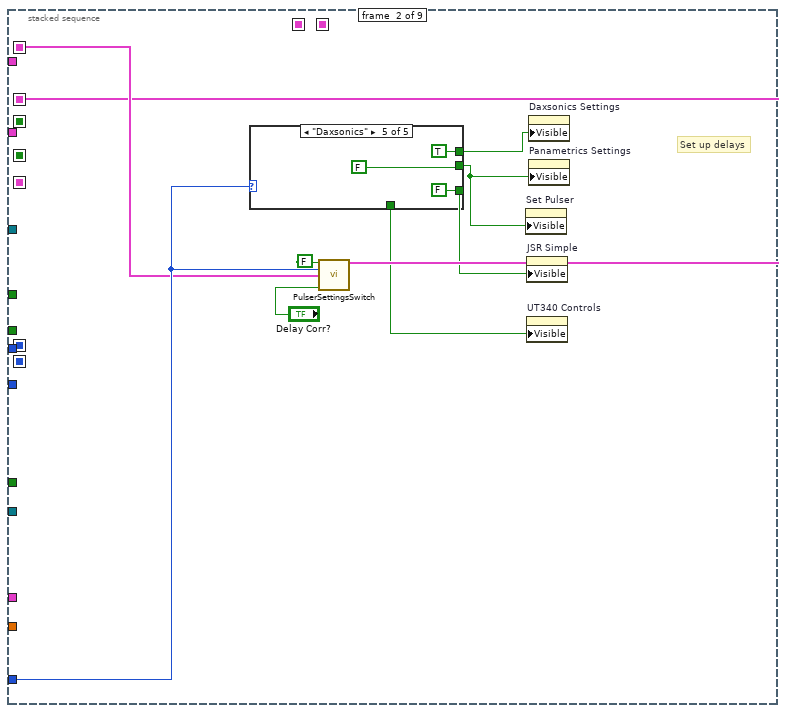
[diagram p20: hidden frame]
diagram:
  n1 = global read "SwitchGlobals.vi" "Full Scan Size"() -> (w10:dbl[])
  n2 = global read "MotionGlobals.vi" "Location"() -> (w9:T43)
  n3 = Unbundle By Name("Digitizer Settings") -> ("bits A/D"=w26:i8)
  n4 = Unbundle By Name("Ann Array Params") -> ("Switch T/R"=w21:i16)
  n5 = property on="Full Scan Size (mm)" class="Arr (strict)"("Value"=w10) -> ()  [unwired: 2 in, 2 out]
  n6 = Decrement(x=w21) -> (x-1=w30:i16)
  n7 = case shown="\"Stony Brook\", Default" w9 {
    tunnel: [w36 w39] -> w23
    tunnel: "Dual XDCR Settings" -> [w36 w38]
    tunnel: w10 -> [_ w37]
    frame "Hawaii" {
    }
    frame "Stony Brook", Default {
      n8 = Bundle By Name(cluster=w38, "Scan Size"=w37) -> (w39:T1)
    }
  }
  n9 = global read "MotionGlobals.vi" "Debug Mode?"() -> (w14:bool)
  n10 = global read "MotionGlobals.vi" "c mm/mics"() -> (w5:sgl)
  n11 = global read "SwitchGlobals.vi" "Switch Unit"() -> (w24:T44)
  n12 = global read "PulserGlobals.vi" "Panametrics"() -> (w6:refnum<visa-resource-name>)
  n13 = local write "Transducer"(w30) -> ()
  n14 = global read "MotionGlobals.vi" "SavePath"() -> (w35:path)
  n15 = global read "PulserGlobals.vi" "Pulser"() -> (w25:T45)
  n16 = call "loglookup.vi"("A/D bits"=w26) -> ("Log Lookup"=w27:sgl[], "Minimum dB"=w1:dbl)  [unwired: 2 in, 2 out]
  n17 = stacked-sequence {
    tunnel: w35 -> [_ w237]
    tunnel: [_ w236] -> w34
    tunnel: [_ w235] -> w33
    tunnel: T42 {"gain"=0.0, TRUE, "Array"=[], "gain 2"=0.0, TRUE} -> [_ w234]
    tunnel: T41 {"Left"=50, "Top"=10, "Right"=500, "Bottom"=455} ("Plot Area Bounds") -> [_ w233]
    tunnel: w30 -> [_ w232]
    tunnel: w5 -> [w55 w231]
    tunnel: [_ w215] -> w8
    tunnel: [_ w230] -> w29
    tunnel: w27 -> [_ w229]
    tunnel: "Digitizer Settings" -> [w56 w228]
    tunnel: w25 -> [w85 w227]
    tunnel: w24 -> [_ w226]
    tunnel: w23 -> [w83 w225]
    tunnel: "Ann Array Params" -> [_ w224]
    tunnel: [_ w223] -> w20
    tunnel: [_ w222] -> w17
    tunnel: TRUE -> [_ w221]
    tunnel: "Type of scan" -> [w88 w220]
    tunnel: w14 -> [w86 w219]
    tunnel: "Motion Settings" -> [_ w218]
    tunnel: [_ w217] -> w11
    tunnel: w9 -> [w87 w216]
    tunnel: w6 -> [_ w214]
    tunnel: w1 -> [w44 _]
    frame #0 {
      # "Hide Decorations if not using them"
      # "Turn on or off controls"
      # "Set XDCR Names"
      # "If Real Time Scan, populate the pulser display\nIf Dual XDCR, it will be set later"
      # "Lock out scanning axis"
      n18 = Unbundle By Name(w83) -> ("XDCR Settings"=w82:T2[])
      n19 = expression code="x/2"(w44) -> (w43:dbl)
      n20 = case shown="\"Dual Transducer\"" w88 {
        tunnel: w85 -> [_ w100]
        frame "Dual Transducer" {
        }
        frame "Real-Time Scan", Default {
          n21 = case shown="\"JSR\"" w100 {
            frame "Pan 5900" {
              n22 = call "5900PRSet.vi"("ExitSendCmd"=TRUE) -> ("Panametrics Settings Out"=w104:T4)  [unwired: 12 in, 2 out]
              n23 = Unbundle By Name(w104) -> ("ENERGY (uJ)"=w105:u16, "COARSE ATTENUATION"=w106:u16, "FINE ATTENUATION"=w107:u16)
              n24 = property on="Panametrics Settings" class="Clust (strict)"() -> ("Value"=w102:T39)  [unwired: 2 in, 2 out]
              n25 = Bundle By Name(cluster=w102, "ENERGY (uJ)"=w105, "COARSE ATTENUATION"=w106, "FINE ATTENUATION"=w107) -> (w103:T39)
              n26 = property on="Panametrics Settings" class="Clust (strict)"("Value"=w103) -> ()  [unwired: 2 in, 2 out]
            }
            frame "JSR" {
              n27 = global read "PulserGlobals.vi" "JSR Settings"() -> (w111:T5)
              n28 = Unbundle By Name(w111) -> ("JSR Pulse Settings.Pulse Energy Level"=w110:T8, "JSR Receive Settings.Gain (dB)"=w108:T15, "JSR Pulse Settings.Pulser Voltage (V)"=w109:T10)
              n29 = Bundle By Name(cluster=T35 {"Pulse Energy Level"=2, "Gain (dB)"=50, "Pulser Voltage (V)"=0} ("JSR Simple"), "Pulse Energy Level"=w110, "Gain (dB)"=w108, "Pulser Voltage (V)"=w109) -> (w112:T35)
              n30 = property on="JSR Simple" class="Clust (strict)"("Value"=w112) -> ()  [unwired: 2 in, 2 out]
            }
            frame "UTEX" {
              n31 = global read "PulserGlobals.vi" "UT340 Controls"() -> (w116:T20)
              n32 = Unbundle By Name(w116) -> ("PE Gain (dB)"=w115:i16, "Voltage"=w114:i16)
              n33 = Bundle By Name(cluster=T38 {"PE Gain (dB)"=1, "Voltage"=100} ("UT340 Controls"), "PE Gain (dB)"=w115, "Voltage"=w114) -> (w117:T38)
              n34 = property on="UT340 Controls" class="Clust (strict)"("Value"=w117) -> ()  [unwired: 2 in, 2 out]
            }
            frame "Agilent 33xxx", Default {
            }
            frame "Daxsonics" {
              n35 = call "Read_Daxsonics_3Pulsers.vi"() -> ("Dax Values"=w119:T3)  [unwired: 5 in, 6 out]
              n36 = property on="Daxsonics Settings" class="Clust (strict)"("Value"=w119) -> ()  [unwired: 2 in, 2 out]
            }
          }
        }
      }
      n37 = Bundle(cluster=cluster{dbl, dbl} {0.0, -60.0} ("dB Range"), w43) -> (w45:cluster{dbl, dbl})  [unwired: 1 in]
      n38 = for {
        tunnel: w82 -> [w213] mode=indexing
        tunnel: [w212] -> w81 mode=indexing
        n39 = Unbundle By Name(w213) -> ("Transducer Name"=w212:string)
      }
      n40 = property on="dB Range" class="Slide (strict)"("Scale.Minimum"=w44, "Value"=w45) -> ()  [unwired: 2 in, 2 out]
      n41 = Decrement(x=2 ("Axis 1")) -> (x-1=w71:i32)
      n42 = Replace Array Subset(array=i32[] [0, 0, 0, 0], new element=2 ("new element/subarray"), index=w71) -> (w70:i32[])
      n43 = case shown="False" w86 {
        tunnel: [w129 w160] -> w79
        tunnel: [w128 w159] -> w78
        tunnel: w87 -> [w127 w158]
        tunnel: [w126 w157] -> w75
        tunnel: [w125 w156] -> w47
        tunnel: [w124 w155] -> w74
        tunnel: [w123 w154] -> w73
        tunnel: w70 -> [w122 w153]
        tunnel: [w121 w152] -> w67
        tunnel: [w120 1.0 ("Cursor.Cursor Position:Cursor Y")] -> w58
        frame False {
          n44 = case shown="\"WCM Main\", Default" w127 {
            tunnel: [w135 FALSE FALSE] -> w125
            tunnel: [w135 TRUE TRUE] -> w129
            tunnel: [w132 w138 i32[] [2, 0, 2, 2]] -> w128
            tunnel: [T46."Enabled" ("Disabled") T46."Enabled" ("Disabled") T46."Disabled and Grayed Out" ("Disabled")] -> w126
            tunnel: [w131 TRUE w145] -> w124
            tunnel: [TRUE TRUE FALSE] -> w123
            tunnel: w122 -> [w132 w138 _]
            tunnel: [w131 FALSE w145] -> w121
            tunnel: [1.0 ("Inc Step Size\n(mm)") 0.5 ("Inc Step Size\n(mm)") 1.0 ("Inc Step Size\n(mm)")] -> w120
            frame "WCM Main", Default {
              (unwired) FALSE
              w131 = FALSE
              w135 = TRUE
            }
            frame "Hawaii" {
            }
            frame "Stony Brook" {
              w145 = TRUE
            }
          }
        }
        frame True {
          n45 = case shown="\"Stony Brook\"" w158 {
            tunnel: [w161 TRUE TRUE] -> w156
            tunnel: [w161 TRUE TRUE] -> w160
            tunnel: [w162 w168 i32[] [2, 0, 2, 2]] -> w159
            tunnel: [FALSE TRUE TRUE] -> _
            tunnel: [T46."Enabled" ("Disabled") T46."Enabled" ("Disabled") T46."Enabled" ("Disabled")] -> w157
            tunnel: [FALSE TRUE w175] -> w155
            tunnel: [TRUE TRUE TRUE] -> w154
            tunnel: w153 -> [w162 w168 _]
            tunnel: [w161 FALSE w175] -> w152
            frame "WCM Main", Default {
              w161 = TRUE
            }
            frame "Hawaii" {
              (unwired) TRUE
            }
            frame "Stony Brook" {
              w175 = TRUE
            }
          }
        }
      }
      n46 = control-ref of="Transducer"() -> (w80:refnum<vi>)
      n47 = property on="Property Node" class="Ring (strict)"(reference=w80, "Strings []"=w81) -> ()  [unwired: 1 in, 2 out]
      n48 = property on="File Name" class="Str"("DisabledEnum"=w75) -> ()  [unwired: 2 in, 2 out]
      n49 = property on="distance?" class="Bool (strict)"("Visible"=w47, "Value"=w79) -> ()  [unwired: 2 in, 2 out]
      n50 = property on="Total Pts" class="Bool (strict)"("Visible"=w47) -> ()  [unwired: 2 in, 2 out]
      n51 = property on="Motion Parameters" class="Clust (strict)"("Visible"=w73) -> ()  [unwired: 2 in, 2 out]
      n52 = property on="Acquistion Parameters" class="Clust (strict)"("Visible"=w73) -> ()  [unwired: 2 in, 2 out]
      n53 = property on="Display mode" class="Ring (strict)"("Visible"=w73) -> ()  [unwired: 2 in, 2 out]
      n54 = property on="Inc Step Size\n(mm)" class="DigNum (strict)"("Value"=w58) -> ()  [unwired: 2 in, 2 out]
      n55 = property on="Force Symmetric?" class="Bool (strict)"("Value"=w67) -> ()  [unwired: 2 in, 2 out]
      n56 = property on="FileName Gen" class="Bool (strict)"("Visible"=w74) -> ()  [unwired: 2 in, 2 out]
      n57 = property on="Center" class="Bool (strict)"("Value"=FALSE ("Center")) -> ()  [unwired: 2 in, 2 out]
      n58 = for {
        tunnel: w78 -> [w206] mode=indexing
        i -> [w207]
        n59 = case shown="0, Default" w207 {
          tunnel: w206 -> [w208 w209 w210 w211]
          frame 0, Default {
            n60 = property on="Axis 1" class="Bool (strict)"("DisabledEnum"=w208) -> ()  [unwired: 2 in, 2 out]
          }
          frame 1 {
            n61 = property on="Axis 2" class="Bool (strict)"("DisabledEnum"=w209) -> ()  [unwired: 2 in, 2 out]
          }
          frame 2 {
            n62 = property on="Axis 3" class="Bool (strict)"("DisabledEnum"=w210) -> ()  [unwired: 2 in, 2 out]
          }
          frame 3 {
            n63 = property on="Axis 4" class="Bool (strict)"("DisabledEnum"=w211) -> ()  [unwired: 2 in, 2 out]
          }
        }
      }
      n64 = case shown="\"Dual Transducer\"" w88 {
        tunnel: [w182 TRUE] -> w40
        tunnel: [TRUE FALSE] -> w59
        tunnel: [T46."Enabled" ("Disabled") T46."Disabled and Grayed Out" ("Disabled")] -> w68
        tunnel: w55 -> [_ w190]
        tunnel: w56 -> [_ w188]
        tunnel: [w182 w185] -> w42
        tunnel: w47 -> [_ w185]
        frame "Real-Time Scan", Default {
          w182 = FALSE
        }
        frame "Dual Transducer" {
          # "Set Blue Cursors"
          n65 = Unbundle By Name(w188) -> ("Samp Rate (Hz)"=w192:dbl, "rf points per line"=w191:i32, "Digitizer delay (us)"=w194:dbl)
          n66 = expression code="x*1e-6"(w192) -> (w195:dbl)
          n67 = Compound Arithmetic op=MULTIPLY(w190, sgl 0.5 ("value")) -> (w196:sgl)
          n68 = Reciprocal(x=w195) -> (1/x=w193:dbl)
          n69 = Compound Arithmetic op=MULTIPLY(w194, w196) -> (w186:dbl)
          n70 = Compound Arithmetic op=MULTIPLY(w193, w191, w196) -> (w197:dbl)
          n71 = Compound Arithmetic op=ADD(w197, w186) -> (w187:dbl)
          n72 = property on="Initilize" class="Bool (strict)"("Val(Sgnl)"=TRUE ("Value (Signaling)")) -> ()  [unwired: 2 in, 2 out]
          n73 = property on="Real Time Image" class="IntGraph (strict)"("Active Cursor"=u32 4, "Cursor.Cursor Y"=w187, "Active Cursor"=u32 3, "Cursor.Cursor Y"=w186) -> ()  [unwired: 2 in, 2 out]
        }
      }
      n74 = control-ref of="Tab Control"() -> (w63:refnum<vi>)
      n75 = control-ref of="This VI"() -> (w65:refnum<vi>)
      n76 = property class="TabCtl (strict)"(reference=w63) -> ("Pages"=w62:refnum<vi>[])  [unwired: 1 in, 2 out]
      n77 = property on="Ref Delay (ms)" class="DigNum (strict)"("DisabledEnum"=w68) -> ()  [unwired: 2 in, 2 out]
      n78 = property on="rf points per line" class="DigNum (strict)"("DisabledEnum"=w68) -> ()  [unwired: 2 in, 2 out]
      n79 = property on="Overshoot" class="DigNum (strict)"("DisabledEnum"=w68) -> ()  [unwired: 2 in, 2 out]
      n80 = property on="BKPT Shift" class="DigNum (strict)"("DisabledEnum"=w68) -> ()  [unwired: 2 in, 2 out]
      n81 = property on="lines per plane" class="DigNum (strict)"("DisabledEnum"=w68) -> ()  [unwired: 2 in, 2 out]
      n82 = property on="view" class="Bool (strict)"("Visible"=w59) -> ()  [unwired: 2 in, 2 out]
      n83 = property on="*.eye" class="Bool (strict)"("Visible"=w59) -> ()  [unwired: 2 in, 2 out]
      n84 = property on="BMP?" class="Bool (strict)"("Visible"=w59) -> ()  [unwired: 2 in, 2 out]
      n85 = property on="scan pair" class="Enum (strict)"("Visible"=w59) -> ()  [unwired: 2 in, 2 out]
      n86 = property on="Save\nDual Transducer\nSettings" class="Bool"("Visible"=w40) -> ()  [unwired: 2 in, 2 out]
      n87 = property on="Re-Load\nDual Transducer\nSettings" class="Bool"("Visible"=w40) -> ()  [unwired: 2 in, 2 out]
      n88 = property on="Transducer" class="Ring (strict)"("Visible"=w40) -> ()  [unwired: 2 in, 2 out]
      n89 = property on="End Point\nMarker" class="Bool (strict)"("Visible"=w40) -> ()  [unwired: 2 in, 2 out]
      n90 = property on="Center" class="Bool (strict)"("Visible"=w40) -> ()  [unwired: 2 in, 2 out]
      n91 = property on="Scan" class="Bool (strict)"("Visible"=w40) -> ()  [unwired: 2 in, 2 out]
      n92 = property class="VI"(reference=w65) -> ("Panel"=w64:refnum<vi>)  [unwired: 1 in, 2 out]
      n93 = property on="Acquisition Volume (mm)" class="Arr (strict)"("Visible"=w40) -> ()  [unwired: 2 in, 2 out]
      n94 = property on="Full Scan Size (mm)" class="Arr (strict)"("Visible"=w40) -> ()  [unwired: 2 in, 2 out]
      n95 = property on="Position (mm) (Pt1)" class="DigNum (strict)"("Visible"=w40) -> ()  [unwired: 2 in, 2 out]
      n96 = property on="Position (mm) (Pt2)" class="DigNum (strict)"("Visible"=w40) -> ()  [unwired: 2 in, 2 out]
      n97 = property on="Movie Name" class="Str"("Visible"=w59) -> ()  [unwired: 2 in, 2 out]
      n98 = property on="BKPT Shift" class="DigNum (strict)"("Visible"=w59) -> ()  [unwired: 2 in, 2 out]
      n99 = property on="Overshoot" class="DigNum (strict)"("Visible"=w59) -> ()  [unwired: 2 in, 2 out]
      n100 = property on="distance?" class="Bool (strict)"("Visible"=w59) -> ()  [unwired: 2 in, 2 out]
      n101 = Not(x=w40) -> (.not. x?=w41:bool)
      n102 = property on="Distance Between Planes (um)" class="Arr (strict)"("Visible"=w42) -> ()  [unwired: 2 in, 2 out]
      n103 = property class="Pnl"(reference=w64) -> ("Decos[]"=w66:refnum<vi>[])  [unwired: 1 in, 2 out]
      n104 = property on="Reset Scan" class="Bool (strict)"("Value"=w41, "Visible"=w40) -> ()  [unwired: 2 in, 2 out]
      n105 = Delete From Array(array=w62, length=1, index=0) -> (array with subset deleted=w54:refnum<vi>[])  [unwired: 1 out]
      n106 = Index Array(array=w54) -> (element=w53:refnum<vi>)  [unwired: 1 in]
      n107 = for {
        tunnel: w66 -> [w99] mode=indexing
        tunnel: w40 -> [w98]
        n108 = property class="Decor"(reference=w99, "Visible"=w98) -> ()  [unwired: 1 in, 2 out]
      }
      n109 = for {
        tunnel: w54 -> [w93] mode=indexing
        tunnel: w40 -> [w92]
        tunnel: [w91] -> w52
        n110 = property class="Page"(reference=w93) -> ("DecosOnPage"=w94:refnum<vi>[])  [unwired: 1 in, 2 out]
        n111 = for {
          tunnel: w94 -> [w97] mode=indexing
          tunnel: w92 -> [w96]
          tunnel: [w95] -> w91
          n112 = property class="Decor"(reference=w97, "Visible"=w96) -> (error out=w95:errorcluster)  [unwired: 1 in, 1 out]
        }
      }
      n113 = for {
        N: 5 -> [_]
        tunnel: w40 -> [w204]
        i -> [w205]
        n114 = property on="Real Time Image" class="IntGraph (strict)"("Active Cursor"=w205, "Cursor.Visible"=w204) -> ()  [unwired: 2 in, 2 out]
      }
      n115 = property class="Page"(reference=w53, error in=w52) -> ("DecosOnPage"=w51:refnum<vi>[])  [unwired: 2 out]
      n116 = Delete From Array(array=w51, length=1, index=2) -> (array with subset deleted=w50:refnum<vi>[])  [unwired: 1 out]
      n117 = for {
        tunnel: w50 -> [w90] mode=indexing
        tunnel: w42 -> [w89]
        n118 = property class="Decor"(reference=w90, "Visible"=w89) -> ()  [unwired: 1 in, 2 out]
      }
      "Found Center" <- FALSE
    }
    frame #1 {
      n119 = while {
        tunnel: w221 -> [w247]
        tunnel: w216 -> [w271]
        tunnel: w237 -> [w270]
        tunnel: [w267] -> w235
        shift-right: [w240] -> w230
        shift-left: w218 -> [w243]
        shift-right: [w269] -> w236
        shift-left: w228 -> [w268]
        tunnel: w234 -> [w263]
        tunnel: w233 -> [w262]
        tunnel: w231 -> [w260]
        shift-right: [w259] -> w215
        shift-left: w232 -> [w261]
        shift-right: [w258] -> w217
        shift-left: w225 -> [w252]
        tunnel: w226 -> [w257]
        tunnel: w227 -> [w256]
        tunnel: [w255] -> _
        tunnel: w229 -> [w250]
        tunnel: w224 -> [w249]
        tunnel: [w248] -> w223
        tunnel: [w246] -> w222
        tunnel: w220 -> [w245]
        tunnel: w219 -> [w244]
        tunnel: w214 -> [w239]
        i -> [w254]
        stop <- w266 stop-if-true
        n120 = Unbundle By Name(w252) -> ("Scan Size"=w251:dbl[])
        n121 = call "OvershootCalc.vi"("Motion Settings In in"=w243, "Num of trigs to overshoot (2.5)"=sgl 4.0) -> ("Motion Settings out"=w242:T26)  [unwired: 3 in, 3 out]
        n122 = Obtain Queue(max queue size (-1, unlimited)=3, element data type=w263) -> (queue out=w264:refnum<queue>)  [unwired: 3 in, 2 out]
        n123 = Equal To 0?(x=w254) -> (x = 0?=w253:bool)
        n124 = stacked-sequence {
          seq-local: [_ _ _ _ _ w681 _ _ _] -> [_ _ _ _ _ _ _ _ w2580]
          seq-local: [w275 _ _ _ _ _ _ _ _] -> [_ w339 _ _ _ _ _ _ _]
          seq-local: [_ w336 _ _ _ _ _ _ _] -> [_ _ w362 w393 w433 _ _ w2551 w2577]
          seq-local: [_ _ w363 _ _ _ _ _ _] -> [_ _ _ w386 w431 _ _ _ _]
          seq-local: [_ _ _ _ w430 _ _ _ _] -> [_ _ _ _ _ w678 w733 _ _]
          seq-local: [_ _ _ _ w429 _ _ _ _] -> [_ _ _ _ _ w679 w732 _ _]
          seq-local: [_ _ w358 _ _ _ _ _ _] -> [_ _ _ _ w426 w677 w730 _ w2573]
          seq-local: [_ _ w357 _ _ _ _ _ _] -> [_ _ _ _ _ _ w729 _ _]
          seq-local: [_ _ w356 _ _ _ _ _ _] -> [_ _ _ w390 w423 _ w728 _ w2574]
          seq-local: [_ _ _ "Pause Mode?" _ _ _ _ _] -> [_ _ _ _ w424 _ w727 _ w2575]
          seq-local: [_ _ _ _ _ _ w726 _ _] -> [_ _ _ _ _ _ _ _ w2571]
          tunnel: [_ _ _ _ w447 _ _ _ _] -> w267
          tunnel: w247 -> [_ _ _ w387 _ _ w736 _ _]
          tunnel: w271 -> [_ _ _ _ w435 _ w749 w2556 _]
          tunnel: w270 -> [_ _ _ _ _ _ w753 _ _]
          tunnel: w268 -> [w279 _ _ _ _ _ _ _ _]
          tunnel: [_ _ _ _ _ _ w752 _ _] -> w269
          tunnel: w242 -> [w276 _ w359 _ _ _ _ w2550 _]
          tunnel: [_ _ _ _ _ _ w751 _ _] -> w266
          tunnel: w264 -> [_ _ _ _ _ _ w750 w2552 _]
          tunnel: w262 -> [_ _ _ _ _ _ w748 _ _]
          tunnel: w261 -> [w277 _ _ _ w438 w680 w745 _ _]
          tunnel: w260 -> [_ _ _ _ _ _ w747 _ _]
          tunnel: [_ _ _ _ _ _ w746 _ _] -> w259
          tunnel: w252 -> [w278 _ _ _ w439 _ w743 _ _]
          tunnel: [_ _ _ _ _ _ w744 _ _] -> w258
          tunnel: w257 -> [_ _ _ _ _ _ w742 _ _]
          tunnel: w256 -> [_ w341 _ _ w434 _ w741 _ _]
          tunnel: [_ _ _ _ w436 _ _ _ _] -> w255
          tunnel: w253 -> [w274 _ _ w391 w428 _ w738 _ _]
          tunnel: w251 -> [_ _ _ _ _ _ w740 _ _]
          tunnel: w250 -> [_ _ _ _ _ _ w739 _ _]
          tunnel: w249 -> [_ _ _ _ _ _ w737 _ w2576]
          tunnel: [_ _ _ _ _ _ _ _ w2576] -> w248
          tunnel: [_ _ _ w390 _ _ _ _ _] -> w246
          tunnel: w245 -> [w273 _ _ _ w427 _ w735 _ w2572]
          tunnel: w244 -> [_ _ _ _ _ _ w734 _ _]
          tunnel: "Full Scan Size (mm)" -> [w272 _ _ _ _ _ _ _ _]
          tunnel: [_ _ _ _ _ _ _ _ w2569] -> w240
          tunnel: w239 -> [_ _ _ _ _ _ w725 _ _]
          frame #0 {
            n125 = case shown="\"Dual Transducer\"" w273 {
              tunnel: w279 -> [w280 w296]
              tunnel: w276 -> [_ w295]
              tunnel: [w280 w299] -> w275
              tunnel: w278 -> [_ w294]
              tunnel: w277 -> [_ w293]
              tunnel: w274 -> [_ w282]
              tunnel: w272 -> [_ w286]
              frame "Therapy With Scan", Default {
              }
              frame "Dual Transducer" {
                n126 = property on="Z Change" class="Bool (strict)"() -> ("Value"=w281:bool)  [unwired: 2 in, 2 out]
                n127 = Or(x=w281, y=w282) -> (x .or. y?=w283:bool)
                n128 = case shown="True" w283 {
                  tunnel: [w303 w321] -> w291
                  tunnel: [w302 w320] -> w290
                  tunnel: w294 -> [_ w318]
                  tunnel: w293 -> [w305 w314]
                  tunnel: "Dual XDCR\nDigi Time Settings" -> [w306 _]
                  tunnel: [w301 w309] -> w289
                  tunnel: w286 -> [w301 w309]
                  frame False {
                    n129 = Index Array(array=w306, index=w305) -> (element=w304:cluster{"RF PPL":i32, "Ref Delay (us)":dbl})
                    n130 = Unbundle By Name(w304) -> ("RF PPL"=w303:i32, "Ref Delay (us)"=w302:dbl)
                  }
                  frame True {
                    n131 = Unbundle By Name(w318) -> ("XDCR Settings"=w317:T2[])
                    n132 = property on="Z Change" class="Bool (strict)"("Value"=FALSE ("Z Change")) -> ()  [unwired: 2 in, 2 out]
                    n133 = in-place {
                      n134 = in-place-array #1(w317, w314) -> (w330:T2)
                      n135 = Unbundle By Name(w330) -> ("XDCR Focal Length"=w332:dbl, "Image Vertical Offset"=w331:dbl)
                      n136 = Add(x=w332, y=w331) -> (x+y=w329:dbl)
                      n137 = Bundle By Name(cluster=w330, "Data Vertical Center"=w329) -> (w328:T2)
                      n138 = in-place-array #1(w328) -> (w316:T2[])  [unwired: 1 out]
                    }
                    n139 = property on="Last End Point" class="DigNum (strict)"("Value"=-inf) -> ()  [unwired: 2 in, 2 out]
                    n140 = Bundle By Name(cluster=w318, "Scan Size"=w309, "XDCR Settings"=w316) -> (w312:T1)
                    n141 = call "SetupTimeScale.vi"("Dual XDCR Settings in"=w312) -> ("Dual XDCR Settings out"=w319:T1)  [unwired: 10 in]
                    n142 = Unbundle By Name(w319) -> ("XDCR Settings"=w311:T2[])
                    n143 = for {
                      tunnel: w311 -> [w327] mode=indexing
                      tunnel: [w324] -> w313 mode=indexing
                      tunnel: [w322] -> w308 mode=indexing
                      n144 = Unbundle By Name(w327) -> ("Digitizer Settings.RF data Sampling.rf points per line"=w326:i32, "Digitizer Settings.RF data Sampling.Ref Delay (ms)"=w325:dbl, "Motion Settings.Distance between\nscan planes (um)"=w322:sgl)
                      n145 = Bundle By Name(cluster=cluster{"RF PPL":i32, "Ref Delay (us)":dbl} {"RF PPL"=0, "Ref Delay (us)"=0.0} ("Cluster"), "RF PPL"=w326, "Ref Delay (us)"=w325) -> (w324:cluster{"RF PPL":i32, "Ref Delay (us)":dbl})
                    }
                    n146 = Index Array(array=w311, index=w314) -> (element=w315:T2)
                    n147 = Unbundle By Name(w315) -> ("Digitizer Settings.RF data Sampling.rf points per line"=w321:i32, "Digitizer Settings.RF data Sampling.Ref Delay (ms)"=w320:dbl)
                    n148 = property on="Distance Between Planes (um)" class="Arr (strict)"("Value"=w308) -> ()  [unwired: 2 in, 2 out]
                    n149 = property on="Dual XDCR\nDigi Time Settings" class="Arr (strict)"("Value"=w313) -> ()  [unwired: 2 in, 2 out]
                  }
                }
                n150 = Unbundle By Name(w295) -> ("Distance between\nscan lines (um)"=w284:sgl)
                n151 = property on="Distance between\nscan lines (um)" class="DigNum (strict)"("Value"=w284) -> ()  [unwired: 2 in, 2 out]
                n152 = Index Array(array=w289, index=0) -> (element=w287:dbl)
                n153 = expression code="x*1e3"(w287) -> (w297:dbl)
                n154 = Divide(x=w297, y=w284) -> (x/y=w298:dbl)
                n155 = call "Force Odd or Even.vi"("Parity (odd)"=enum16{"Odd", "Even"}."Odd" ("Parity"), "input"=w298) -> ("output"=w285:i32)
                "FixedLinesPerPlane" <- w285
                n156 = property on="lines per plane" class="DigNum (strict)"("Value"=w285) -> ()  [unwired: 2 in, 2 out]
                n157 = Bundle By Name(cluster=w296, "lines per plane"=w285, "rf points per line"=w291, "Digitizer delay (us)"=w290) -> (w299:T30)
                n158 = property on="Ref Delay (ms)" class="DigNum (strict)"("Value"=w290) -> ()  [unwired: 2 in, 2 out]
                n159 = property on="rf points per line" class="DigNum (strict)"("Value"=w291) -> ()  [unwired: 2 in, 2 out]
              }
            }
          }
          frame #1 {
            # "Set up delays"
            n160 = case shown="\"Daxsonics\"" w341 {
              tunnel: [TRUE ("Visible") TRUE ("Visible") w348 FALSE ("Visible") FALSE ("Visible")] -> w338
              tunnel: [FALSE ("Visible") FALSE ("Visible") w348 TRUE ("Visible") FALSE ("Visible")] -> w335
              tunnel: [FALSE ("Visible") FALSE ("Visible") w348 FALSE ("Visible") TRUE ("Visible")] -> w334
              tunnel: [_ _ TRUE _ _] -> w333
              frame "Pan 5900" {
              }
              frame "No Pulser", Default {
              }
              frame "UTEX" {
                w348 = FALSE
              }
              frame "JSR" {
              }
              frame "Daxsonics" {
              }
            }
            n161 = call "PulserSettingsSwitch.vi"("Initilize?"=FALSE, "Pulser"=w341, "Digitizer Settings in"=w339, "Delay Corr?"="Delay Corr?") -> ("Digitizer Settings out"=w336:T30)  [unwired: 9 in, 2 out]
            n162 = property on="Set Pulser" class="Bool"("Visible"=w338) -> ()  [unwired: 2 in, 2 out]
            n163 = property on="JSR Simple" class="Clust (strict)"("Visible"=w335) -> ()  [unwired: 2 in, 2 out]
            n164 = property on="UT340 Controls" class="Clust (strict)"("Visible"=w333) -> ()  [unwired: 2 in, 2 out]
            n165 = property on="Daxsonics Settings" class="Clust (strict)"("Visible"=w334) -> ()  [unwired: 2 in, 2 out]
            n166 = property on="Panametrics Settings" class="Clust (strict)"("Visible"=w338) -> ()  [unwired: 2 in, 2 out]
          }
          frame #2 {
            w356 = FALSE
            n167 = Unbundle By Name(w359) -> ("SMAC Axis"=w360:u16, "scan pair"=w361:T28)
            n168 = property on="scan pair" class="Enum (strict)"("Value"=w361) -> ()  [unwired: 2 in, 2 out]
            n169 = call "GetScanAxis.vi"("scan pair"=w361) -> ("Axis 1"=w358:i32, "Axis 2"=w357:i32)  [unwired: 1 in, 1 out]
            n170 = Equal?(x=w360, y=w358) -> ()  [unwired: 1 out]
            n171 = property on="Pause Motion" class="Bool (strict)"("Visible"=w356) -> ()  [unwired: 2 in, 2 out]
            n172 = case shown="False" w356 {
              tunnel: w359 -> [w370 w385]
              tunnel: [w373 w385] -> w363
              tunnel: w362 -> [w384 _]
              tunnel: w358 -> [w379 _]
              frame False {
                n173 = Unbundle By Name(w384) -> ("lines per plane"=w381:i32)
                n174 = Unbundle By Name(w370) -> ("Distance between\nscan lines (um)"=w383:sgl, "Motor Parameters.velocity ct/s"=w380:dbl[], "Steps per mm"=w378:i32[])
                n175 = expression code="x*1e-3"(w383) -> (w382:sgl)
                n176 = Index Array(array=w380, index=w379) -> (element=w377:dbl)
                n177 = Index Array(array=w378, index=w379) -> (element=w376:i32)
                n178 = Multiply(x=w381, y=w382) -> (x*y=w375:sgl)
                n179 = Divide(x=w377, y=w376) -> (x/y=w374:dbl)
                n180 = To Single Precision Float(number=w374) -> (single precision float=w368:sgl)
                n181 = Divide(x=w375, y=w368) -> (x/y=w372:sgl)
                n182 = Reciprocal(x=w372) -> (1/x=w367:sgl)
                n183 = Unbundle By Name(w370) -> ("RT fps"=w369:sgl)
                n184 = call-poly "Decimal Rounding Poly.vi"("Round Method (Nearest)"=T47."Round to -INF", "Input"=w367) -> ("Output"=w366:dbl)  [unwired: 9 in]
                n185 = Max & Min(x=w369, y=w366) -> (min(x,y)=w371:dbl)  [unwired: 1 out]
                n186 = Bundle By Name(cluster=w370, "RT fps"=w371) -> (w373:T26)
              }
              frame True {
              }
            }
            n187 = case shown="False" w356 {
              frame False {
                n188 = property on="Pause Mode?" class="Bool (strict)"("Value"=TRUE ("Pause Mode?")) -> ()  [unwired: 2 in, 2 out]
              }
              frame True {
              }
            }
          }
          frame #3 {
            n189 = Unbundle By Name(w386) -> ("Motion System"=w392:T27)
            n190 = Unbundle By Name(w393) -> ("Dig Config"=w388:T32)
            n191 = case shown="\"NI 735x\"" w392 {
              tunnel: w391 -> [_ w405]
              tunnel: w386 -> [_ w404]
              frame "MM3000", Default {
              }
              frame "NI 735x" {
                n192 = disable-structure shown="Disabled" {
                  disable-tunnel: w405 -> [w407 _]
                  disable-tunnel: w404 -> [w406 _]
                  frame Disabled {
                    n193 = case shown="True" w407 {
                      tunnel: w406 -> [_ w409]
                      frame False {
                      }
                      frame True {
                        n194 = Unbundle By Name(w409) -> ("Motion Bd ID"=w408:u8)
                        n195 = while {
                          tunnel: w408 -> [w410]
                          i -> [w412]
                          stop <- w415 stop-if-true
                          n196 = call <vilib>:"Flush Return Data Buffer.flx"("Board ID"=w410) -> ("error out"=w418:errorcluster, "Bd ID Out"=w419:T54)  [unwired: 6 in]
                          n197 = call <vilib>:"Clear Faults.vi"("error in (no error)"=w418, "board in"=w419) -> ("error out"=w417:errorcluster)  [unwired: 8 in, 1 out]
                          n198 = Unbundle(w417) -> ("status"=w416:bool)  [unwired: 2 out]
                          n199 = Not(x=w416) -> (.not. x?=w413:bool)
                          n200 = Greater?(x=w412, y=5 ("x")) -> (0:w414:bool)
                          n201 = Or(x=w413, y=w414) -> (x .or. y?=w415:bool)
                        }
                      }
                    }
                  }
                  frame Enabled {
                  }
                }
              }
            }
            n202 = case shown="\"Single channel\", Default" w388 {
              tunnel: "Pause Mode?" -> [w397 _]
              tunnel: w387 -> [w396 _]
              tunnel: w386 -> [w395 _]
              frame "Single channel", Default {
                # "turn on RT trig"
                n203 = case shown="False" w397 {
                  tunnel: [w400 w403] -> w398
                  tunnel: w396 -> [w402 _]
                  frame False {
                    w399 = u16 1 items=["Function Gen Input", "Motion Trig", "Internal RT Motion Trig", "Internal CTR 1 Output"] ("Trig Source")
                    w401 = u16 2 items=["Function Gen Input", "Motion Trig", "Internal RT Motion Trig", "Internal CTR 1 Output"] ("Trig Source")
                    # "turn on gated RT trig"
                    n204 = Select(t=w399, s=w402, f=w401) -> (s? t:f=w400:u16)
                  }
                  frame True {
                    w403 = u16 1 items=["Function Gen Input", "Motion Trig", "Internal RT Motion Trig", "Internal CTR 1 Output"] ("Trig Source")
                    # "turn on motion trig"
                  }
                }
                n205 = Unbundle By Name(w395) -> ("GL Ref Out"=w394:refnum<k7>)
                n206 = call "RouteTrigSource.vi"("Galil.IGalil"=w394, "Trig Source"=w398) -> ()  [unwired: 9 in, 1 out]
              }
              frame "Empty" {
              }
            }
          }
          frame #4 {
            n207 = case shown="\"Dual Transducer\"" w427 {
              tunnel: w433 -> [w638 w653]
              tunnel: [w638 w647] -> w425
              tunnel: w439 -> [_ w663]
              tunnel: w431 -> [w639 w662]
              tunnel: w438 -> [_ w661]
              tunnel: w434 -> [_ w654]
              tunnel: [w639 w644] -> w421
              tunnel: [w638 w646] -> w422
              frame "M scan", Default {
              }
              frame "Dual Transducer" {
                n208 = To Unsigned Long Integer(number=w661) -> (unsigned 32bit integer=w648:u32)
                n209 = control-ref of="Daxsonics Settings"() -> (w657:refnum<vi>)
                n210 = Increment(x=w648) -> (x+1=w660:u32)
                n211 = control-ref of="Filter Prams"() -> (w658:refnum<vi>)
                n212 = control-ref of="JSR Simple"() -> (w641:refnum<vi>)
                n213 = property on="Dual XDCR\nDigi Time Settings" class="Arr (strict)"() -> ("Value"=w649:cluster{"RF PPL":i32, "Ref Delay (us)":dbl}[])  [unwired: 2 in, 2 out]
                n214 = control-ref of="Panametrics Settings"() -> (w655:refnum<vi>)
                n215 = control-ref of="UT340 Controls"() -> (w640:refnum<vi>)
                n216 = Index Array(array=w649, index=w648) -> (element=w650:cluster{"RF PPL":i32, "Ref Delay (us)":dbl})
                n217 = call "ChooseDualXDCRSettings.vi"("Digitizer Settings in"=w653, "Switch T/R"=w660, "Pulser"=w654, "Motion Settings in"=w662, "Dual XDCR Settings"=w663, "Setup Time\nParameters (F)"=TRUE ("Setup Time\nParameters (F)"), "Allow USB R/Ws?"=FALSE, "JSR Simple"=w641, "Filter Parameters Ref"=w658, "Daxsonics Settings Ref"=w657, "Panametrics Simple Ref"=w655, "UT340 Simple Ref"=w640) -> ("Digitizer Settings"=w647:T30, "Motion Settings"=w642:T26)  [unwired: 13 in, 1 out]
                n218 = Unbundle By Name(w650) -> ("Ref Delay (us)"=w651:dbl, "RF PPL"=w652:i32)
                n219 = property on="FixedLinesPerPlane" class="DigNum (strict)"() -> ("Value"=w643:i32)  [unwired: 2 in, 2 out]
                n220 = call "CalcTotalScanCts.vi"("Number of scan lines"=w643, "Motion Settings In"=w642) -> ("Total Steps"=w645:dbl)  [unwired: 9 in]
                n221 = Bundle By Name(cluster=w642, "Total steps in line"=w645) -> (w644:T26)
                n222 = Bundle By Name(cluster=w647, "lines per plane"=w643, "Digitizer delay (us)"=w651, "rf points per line"=w652) -> (w646:T30)
              }
            }
            n223 = Unbundle By Name(w421) -> ("Motion System"=w420:T27)
            n224 = case shown="\"NI 735x\", \"Galil\"" w420 {
              selector: w420 -> [w456 _]
              tunnel: [w478 _] -> w447
              tunnel: [w477 _] -> w436
              tunnel: w423 -> [w468 _]
              tunnel: w422 -> [w462 w636]
              tunnel: w424 -> [w464 _]
              tunnel: w421 -> [w476 w637]
              tunnel: w426 -> [w458 _]
              tunnel: w435 -> [w474 _]
              tunnel: [w463 w637] -> w430
              tunnel: [w462 w636] -> w429
              tunnel: w428 -> [w461 _]
              tunnel: w427 -> [w459 _]
              frame "NI 735x", "Galil" {
                w455 = FALSE ("t")
                n225 = property on="Found Center" class="Bool (strict)"() -> ("Value"=w472:bool)  [unwired: 2 in, 2 out]
                n226 = Not(x=w472) -> (.not. x?=w471:bool)
                n227 = Unbundle By Name(w476) -> ("SMAC Axis"=w470:u16, "Motor Parameters"=w460:T55)
                n228 = Equal?(x=w474, y=location."Stony Brook") -> (x = y?=w475:bool)
                n229 = Compound Arithmetic op=OR(w471, w475) -> (w467:bool)
                n230 = Select(t=w467, s=w468, f=w455) -> (s? t:f=w469:bool)
                n231 = case shown="False" w464 {
                  tunnel: w476 -> [w490 w608]
                  tunnel: [w483 w602] -> w463
                  tunnel: w470 -> [w489 _]
                  tunnel: w469 -> [w488 _]
                  tunnel: [FALSE ("Pause SMAC") w601] -> w465
                  tunnel: w461 -> [_ w607]
                  tunnel: w460 -> [w486 _]
                  tunnel: w459 -> [_ w606]
                  tunnel: w458 -> [_ w605]
                  tunnel: [w485 w604] -> w457
                  tunnel: w456 -> [w480 _]
                  tunnel: w455 -> [w479 _]
                  frame False {
                    n232 = case shown="\"NI 735x\"" w480 {
                      tunnel: w490 -> [w491 w498 w545]
                      tunnel: w489 -> [_ w497 w544]
                      tunnel: w488 -> [_ w496 w539]
                      tunnel: w486 -> [_ w495 w543]
                      tunnel: [_ w494 w540] -> w485
                      tunnel: [w491 w493 w542] -> w484
                      tunnel: [_ w492 w541] -> w481
                      tunnel: w479 -> [_ _ _]
                      frame "MM3000", Default {
                      }
                      frame "NI 735x" {
                        n233 = case shown="True" w496 {
                          selector: w496 -> [_ w511]
                          tunnel: w497 -> [w505 w509]
                          tunnel: w498 -> [w500 w506]
                          tunnel: w495 -> [_ w510]
                          tunnel: [w504 w508] -> w494
                          tunnel: [w500 w506] -> w493
                          tunnel: [w503 w507] -> w492
                          frame False {
                            n234 = Unbundle By Name(w500) -> ("Motion Bd ID"=w499:u8)
                            n235 = call "MoveMotor.vi"("Position Mode (Absolute)"=T48."Absolute Position", "Target Position (0)"=0, "Axis or Vector Space"=w505, "Motion Bd ID"=w499) -> ("error out"=w503:errorcluster, "Resource Output"=w504:u16)  [unwired: 5 in, 1 out]
                          }
                          frame True {
                            n236 = disable-structure shown="Disabled" {
                              disable-tunnel: w511 -> [w531 _]
                              disable-tunnel: w510 -> [w524 _]
                              disable-tunnel: w509 -> [w519 _]
                              disable-tunnel: [w515 _] -> w508
                              disable-tunnel: [w514 _] -> w507
                              disable-tunnel: w506 -> [w513 _]
                              frame Disabled {
                                n237 = Not(x=w531) -> (.not. x?=w529:bool)
                                n238 = Unbundle By Name(w524) -> ("velocity ct/s"=w523:dbl[], "accel ct/s^2"=w522:dbl[])
                                n239 = Unbundle By Name(w513) -> ("Motion Bd ID"=w512:u8)
                                n240 = property on="Found Center" class="Bool (strict)"("Value"=w529) -> ()  [unwired: 2 in, 2 out]
                                n241 = Decrement(x=w519) -> (x-1=w518:u16)
                                n242 = Index Array(array=w523, index=w518) -> (element=w521:dbl)
                                n243 = Index Array(array=w522, index=w518) -> (element=w520:dbl)
                                n244 = call <vilib>:"Load Velocity.flx"("Velocity (10000)"=w521, "Axis or Vector Space"=w519, "Board ID"=w512) -> ("error out"=w528:errorcluster, "Resource Output"=w517:T56, "Bd ID Out"=w527:T54)  [unwired: 4 in]
                                n245 = call "Load Acceleration/Deceleration.flx"("Acceleration (100000)"=w520, "error in (no error)"=w528, "Axis or Vector Space"=w517, "Board ID"=w527) -> ("error out"=w516:errorcluster, "Resource Output"=w525:T56, "Bd ID Out"=w526:T54)  [unwired: 3 in]
                                n246 = call <vilib>:"Find Reference.flx"("Search Type"=T49."Center", "error in (no error)"=w516, "Axis or Vector Space"=w525, "Board ID"=w526) -> ("error out"=w530:errorcluster, "Axis or Vector Space Output"=w536:T57, "Bd ID Out"=w537:T54)  [unwired: 5 in]
                                n247 = call <vilib>:"Wait Reference.flx"("error in (no error)"=w530, "Axis or Vector Space"=w536, "Board ID"=w537) -> ("error out"=w532:errorcluster, "Axis or Vector Space Output"=w534:T57, "Bd ID Out"=w535:T54)  [unwired: 5 in, 1 out]
                                n248 = call <vilib>:"Reset Position.flx"("Primary Reset Position (0)"=0, "error in (no error)"=w532, "Axis"=w534, "Board ID"=w535) -> ("error out"=w514:errorcluster, "Resource Output"=w515:T56)  [unwired: 3 in, 1 out]
                              }
                              frame Enabled {
                              }
                            }
                          }
                        }
                      }
                      frame "Galil" {
                        n249 = case shown="True" w539 {
                          tunnel: w544 -> [w556 w577]
                          tunnel: w545 -> [w559 w596]
                          tunnel: w543 -> [_ w599]
                          tunnel: [w556 w577] -> w540
                          tunnel: [w559 w596] -> w542
                          tunnel: [w558 w589] -> w541
                          frame False {
                            n250 = Unbundle By Name(w559) -> ("GL Ref Out"=w557:refnum<k7>)
                            n251 = Decrement(x=w556) -> (x-1=w555:u16)
                            n252 = call "GL Command Set.vi"("Command"=Command_Menu."Halt Execute", "Value"=-1, "Axis"=w555, "Galil.IGalil"=w557) -> ("error out"=w551:errorcluster, "Axis Out"=w546:T58, "ref out"=w550:refnum<k7>)  [unwired: 3 in, 2 out]
                            n253 = call "GL CheckForMotion.vi"("error in"=w551, "Axis"=w546, "Refnum in"=w550) -> ("error out"=w548:errorcluster, "Axis out"=w547:T58, "Refnum out"=w549:refnum<k7>)  [unwired: 6 in]
                            n254 = call "GL Set Operation Mode.vi"("position cts (abs/rel)"=0, "Position Mode (Absolute)"=T48."Absolute Position", "error in (no error)"=w548, "Start Now?"=TRUE, "Axis"=w547, "Galil.IGalil"=w549) -> ("error out"=w558:errorcluster)  [unwired: 3 in, 2 out]
                          }
                          frame True {
                            n255 = Unbundle By Name(w599) -> ("velocity ct/s"=w598:dbl[], "accel ct/s^2"=w597:dbl[])
                            n256 = Unbundle By Name(w596) -> ("GL Ref Out"=w570:refnum<k7>)
                            n257 = Decrement(x=w577) -> (x-1=w571:u16)
                            n258 = property on="Found Center" class="Bool (strict)"("Value"=TRUE ("Found Center")) -> ()  [unwired: 2 in, 2 out]
                            n259 = call "GL Command Set.vi"("Command"=Command_Menu."Halt Execute", "Value"=-1, "Axis"=w571, "Galil.IGalil"=w570) -> ("error out"=w567:errorcluster, "Axis Out"=w563:T58, "ref out"=w562:refnum<k7>)  [unwired: 3 in, 2 out]
                            n260 = call "GL CheckForMotion.vi"("error in"=w567, "Axis"=w563, "Refnum in"=w562) -> ("error out"=w566:errorcluster, "Axis out"=w564:T58, "Refnum out"=w565:refnum<k7>)  [unwired: 6 in]
                            n261 = Index Array(array=w598, index=w571) -> (element=w580:dbl)
                            n262 = Index Array(array=w597, index=w571) -> (element=w579:dbl)
                            n263 = call "GL Command Set.vi"("Command"=Command_Menu."Velocity", "error in (no error)"=w566, "Value"=w580, "Axis"=w564, "Galil.IGalil"=w565) -> ("error out"=w583:errorcluster, "Axis Out"=w578:T58, "ref out"=w574:refnum<k7>)  [unwired: 2 in, 2 out]
                            n264 = call "GL Command Set.vi"("Command"=Command_Menu."Acceleration", "error in (no error)"=w583, "Value"=w579, "Axis"=w578, "Galil.IGalil"=w574) -> ("error out"=w573:errorcluster, "Axis Out"=w584:T58, "ref out"=w575:refnum<k7>)  [unwired: 2 in, 2 out]
                            n265 = call "GL Command Set.vi"("Command"=Command_Menu."Deceleration", "error in (no error)"=w573, "Value"=w579, "Axis"=w584, "Galil.IGalil"=w575) -> ("error out"=w586:errorcluster, "Axis Out"=w585:T58, "ref out"=w587:refnum<k7>)  [unwired: 2 in, 2 out]
                            n266 = call "GL Center.vi"("error in"=w586, "Axis"=w585, "Galil.IGalil"=w587) -> ("error out"=w594:errorcluster, "Axis Out"=w593:T58, "Galil Out"=w595:refnum<k7>)  [unwired: 4 in]
                            n267 = call "GL CheckForMotion.vi"("error in"=w594, "Axis"=w593, "Refnum in"=w595) -> ("error out"=w588:errorcluster, "Axis out"=w591:T58, "Refnum out"=w590:refnum<k7>)  [unwired: 6 in]
                            n268 = call "GL Command Set.vi"("Command"=Command_Menu."Define Pos", "error in (no error)"=w588, "Axis"=w591, "Galil.IGalil"=w590) -> ("error out"=w589:errorcluster)  [unwired: 3 in, 4 out]
                          }
                        }
                      }
                    }
                    n269 = call "FindLocation.vi"("Motion Settings"=w484, "error in (no error)"=w481) -> ("Motion Settings Out"=w483:T26, "location (mm)"=→"Scan Start Pos (mm)":dbl[])  [unwired: 1 in, 2 out]
                  }
                  frame True {
                    n270 = case shown="False" w607 {
                      tunnel: w608 -> [w616 w635]
                      tunnel: [w613 w634] -> w603
                      tunnel: w606 -> [w618 _]
                      tunnel: w605 -> [w614 w633]
                      tunnel: [w614 w633] -> w604
                      tunnel: [w612 w632] -> w600
                      frame False {
                        n271 = property on="Dual XDCR \nHome (mm)" class="Arr (strict)"() -> ("Value"=w617:dbl[])  [unwired: 2 in, 2 out]
                        n272 = case shown="\"Real-Time Scan\", Default" w618 {
                          tunnel: [w626 w631] -> w612
                          tunnel: w617 -> [w627 w631]
                          tunnel: w614 -> [w629 _]
                          tunnel: w616 -> [w625 w630]
                          tunnel: [w628 w630] -> w615
                          frame "Real-Time Scan", Default {
                            n273 = call "FindLocation.vi"("Motion Settings"=w625, "Wait for Motion Complete"=TRUE) -> ("Motion Settings Out"=w628:T26, "location (mm)"=w624:dbl[])  [unwired: 1 in, 2 out]
                            n274 = Decrement(x=w629) -> (x-1=w622:i32)
                            n275 = Index Array(array=w627, index=w622) -> (element=w623:dbl)
                            n276 = Replace Array Subset(array=w624, new element=w623, index=w622) -> (w626:dbl[])
                          }
                          frame "Dual Transducer" {
                          }
                        }
                        n277 = call "MultiAxisMove.vi"("Find Location"=TRUE, "Wait For Move Complete"=TRUE, "Position Mode (Rel)"=T48."Absolute Position" ("Position Mode (Absolute)"), "Distance to move (mm)"=w612, "Motion Settings"=w615) -> ("Motion Settings Out"=w613:T26)  [unwired: 4 in, 2 out]
                      }
                      frame True {
                        n278 = call "FindLocation.vi"("Motion Settings"=w635) -> ("Motion Settings Out"=w634:T26, "location (mm)"=w632:dbl[])  [unwired: 2 in, 2 out]
                      }
                    }
                    n279 = while {
                      tunnel: [w610] -> w602
                      tunnel: w603 -> [w610]
                      tunnel: [w609] -> w601
                      stop <- w609 continue-if-true
                      n280 = property on="Pause Motion" class="Bool (strict)"() -> ("Value"=w609:bool)  [unwired: 2 in, 2 out]
                    }
                    n281 = property on="Scan Start Pos (mm)" class="Arr (strict)"("Value"=w600) -> ()  [unwired: 2 in, 2 out]
                  }
                }
                n282 = property on="Pause Motion" class="Bool (strict)"("Value"=w465) -> ()  [unwired: 2 in, 2 out]
                n283 = call "PrepForScan.vi"("Motion Settings In"=w463, "Pause?"=w464, "SMAC?"=w468, "Scan Axis"=w457, "MoveBack?"=TRUE, "Digitizer Settings"=w462) -> ("Program ID"=w477:u8, "error out"=w478:errorcluster)  [unwired: 4 in, 4 out]
              }
              frame "No Motion Card", Default {
              }
            }
            n284 = Unbundle By Name(w421) -> ("Distance between\nscan lines (um)"=w444:sgl, "RT fps"=w443:sgl, "BKPT Shift"=w442:i32, "overshoot cts"=w440:i32, "Motion System"=w437:T27)
            n285 = flat-sequence {
              tunnel: w425 -> [w664]
              tunnel: [w664] -> w446
              tunnel: w446 -> [w676]
              frame #0 {
                n286 = control-ref of="Freq (MHz)"() -> (w667:refnum<vi>)
                n287 = control-ref of="Voltage (V)"() -> (w666:refnum<vi>)
                n288 = control-ref of="Gain (dB)"() -> (w665:refnum<vi>)
                n289 = call "JSR_Control_Enumerator.vi"("Voltage (V) Ref"=w665, "Gain (db) Ref"=w666, "Pulse Energy Level Ref"=w667) -> ()  [unwired: 6 in, 3 out]
                n290 = call "DigControlSettings.vi"("Digitizer Settings"=w664) -> ("Sampling Rates"=w668:T59, "Voltage Scale"=w669:T59)  [unwired: 6 in, 3 out]
                n291 = property on="Dig Scale" class="Ring (strict)"("StringsAndValues[]"=w669) -> ()  [unwired: 2 in, 2 out]
                n292 = property on="Sampling Rate" class="Ring (strict)"("StringsAndValues[]"=w668) -> ()  [unwired: 2 in, 2 out]
              }
              frame #1 {
                n293 = Unbundle By Name(w676) -> ("Samp Rate (Hz)"=w673:dbl, "Digitizer delay (us)"=w671:dbl, "rf points per line"=w672:i32, "Voltage Scale"=w675:dbl)
                n294 = expression code="x*1E-6"(w673) -> (w674:dbl)
                n295 = Bundle("Samp Rate (Hz)"=w674, "Digitizer delay (us)"=w671, "rf points per line"=w672, "Voltage Scale"=w675) -> (w670:T60)  [unwired: 1 in]
                n296 = property on="Acquistion Parameters" class="Clust (strict)"("Value"=w670) -> ()  [unwired: 2 in, 2 out]
              }
            }
            n297 = Unbundle By Name(w422) -> ("lines per plane"=w445:i32)
            n298 = Unbundle By Name(w422) -> ("Main Digitizer"=w432:T31)
            n299 = case shown="\"AlazarTech\"" w432 {
              tunnel: w423 -> [_ w450]
              tunnel: w437 -> [_ w449]
              tunnel: w421 -> [_ w448]
              frame "Acqiris Digitizer", Default {
              }
              frame "AlazarTech" {
                n300 = case shown="True" w450 {
                  tunnel: w449 -> [_ w452]
                  tunnel: w448 -> [_ w451]
                  frame False {
                  }
                  frame True {
                    n301 = case shown="\"NI 735x\"" w452 {
                      tunnel: w451 -> [w453 _]
                      frame "NI 735x" {
                        n302 = call "LoadPauseProgram.vi"("Motion Settings"=w453) -> ("error out"=w454:errorcluster)  [unwired: 10 in]
                        n303 = local write "error out"(w454) -> ()
                      }
                      frame "No Motion Card", Default {
                      }
                    }
                  }
                }
              }
            }
            n304 = Bundle("lines per plane"=w445, "Distance between\nscan lines (um)"=w444, "RT fps"=w443, "BKPT Shift"=w442, "overshoot cts"=w440) -> (w441:T61)  [unwired: 1 in]
            n305 = local write "Motion Parameters"(w441) -> ()
          }
          frame #5 {
            n306 = Unbundle By Name(w679) -> ("Dig Config"=w682:T32)
            n307 = case shown="\"5-CH pulser w/ ann array\"" w682 {
              tunnel: [_ w693 _] -> w681
              tunnel: w679 -> [_ w687 w721]
              tunnel: w678 -> [_ w684 w720]
              tunnel: w680 -> [_ w686 w722]
              tunnel: w677 -> [_ w685 w718]
              frame "Single channel", Default {
              }
              frame "5-CH pulser w/ ann array" {
                n308 = Replace Array Subset(array=bool[] [FALSE, FALSE, FALSE, FALSE, FALSE] ("XMIT"), new element=TRUE ("new element/subarray"), index=w686) -> (w688:bool[])
                n309 = call "5ChPulserTrigsNew.vi"("Motion Settings"=w684, "Digitizer Settings"=w687, "XMIT"=w688, "Axis"=w685) -> ("5CH Pulser Tasks"=w695:refnum<k21>[])  [unwired: 5 in, 1 out]
                n310 = for {
                  tunnel: w695 -> [w717] mode=indexing
                  tunnel: [w716] -> w693 mode=indexing
                  tunnel: [w715] -> w692
                  n311 = call <vilib>:"DAQmx Start Task.vi"("task/channels in"=w717) -> ("task out"=w716:refnum<k21>, "error out"=w715:errorcluster)  [unwired: 1 in, 12 out]
                }
                n312 = for {
                  tunnel: bool[][] [[TRUE], [FALSE]] ("data") -> [w709] mode=indexing
                  tunnel: w692 -> [_]
                  tunnel: [w708] -> w691
                  n313 = flat-sequence {
                    tunnel: w709 -> [w712]
                    tunnel: [w712] -> w710
                    tunnel: w710 -> [w714]
                    tunnel: [w713] -> w708
                    frame #0 {
                      n314 = Wait (ms)(milliseconds to wait=u32 25) -> ()  [unwired: 1 out]
                    }
                    frame #1 {
                      n315 = call "DAQ Assistant"("data"=w714) -> ("error out"=w713:errorcluster)  [unwired: 17 in, 1 out]
                    }
                  }
                }
                n316 = Unbundle By Name(w684) -> ("Motion System"=w683:T27)
                n317 = case shown="\"NI 735x\"" w683 {
                  tunnel: w691 -> [_ w698 w704]
                  tunnel: w684 -> [_ w696 w702]
                  frame "MM3000", Default {
                  }
                  frame "NI 735x" {
                    n318 = Unbundle By Name(w696) -> ("Motion Bd ID"=w697:u8)
                    n319 = for {
                      N: 3 -> [_]
                      tunnel: w697 -> [w701]
                      tunnel: w698 -> [w700]
                      n320 = call "ForceBreakPt.vi"("error in"=w700, "Bd ID in"=w701) -> ()  [unwired: 2 out]
                    }
                  }
                  frame "Galil" {
                    n321 = Unbundle By Name(w702) -> ("GL Ref Out"=w703:refnum<k7>)
                    n322 = for {
                      N: 3 -> [_]
                      tunnel: w703 -> [w707]
                      tunnel: w704 -> [w706]
                      n323 = call "GL_ForceBreakPt.vi"("error in"=w706, "GL Ref Out"=w707) -> ()  [unwired: 2 out]
                    }
                  }
                }
              }
              frame "5-CH Pulser New" {
                n324 = Replace Array Subset(array=bool[] [FALSE, FALSE, FALSE, FALSE, FALSE] ("XMIT"), new element=TRUE ("new element/subarray"), index=w722) -> (w719:bool[])
                n325 = call "DaxInternaMultiTrig.vi"("Motion Settings"=w720, "Digitizer Settings"=w721, "XMIT"=w719, "Axis"=w718) -> ()  [unwired: 6 in, 1 out]
              }
            }
          }
          frame #6 {
            n326 = while {
              tunnel: w753 -> [w788]
              tunnel: w727 -> [w787]
              shift-right: [w785] -> w752
              shift-left: w732 -> [w768]
              shift-right: [w784] -> w726
              shift-left: w733 -> [w774]
              tunnel: [w783] -> w751
              tunnel: w750 -> [w782]
              tunnel: w749 -> [w772]
              tunnel: w748 -> [w781]
              tunnel: w747 -> [w780]
              shift-right: [w779] -> w746
              shift-left: w745 -> [w773]
              shift-right: [w778] -> w744
              shift-left: w743 -> [w763]
              tunnel: w742 -> [w777]
              tunnel: w741 -> [w776]
              tunnel: w730 -> [w775]
              shift-right: [w771] -> _
              shift-left: w740 -> [w770]
              tunnel: w739 -> [w769]
              tunnel: w738 -> [w766]
              tunnel: w737 -> [w762]
              tunnel: w736 -> [w761]
              tunnel: w728 -> [w760]
              tunnel: w735 -> [w759]
              tunnel: w734 -> [w758]
              shift-right: [w756] -> _
              shift-left: TRUE -> [w757]
              tunnel: w729 -> [w755]
              tunnel: w725 -> [w754]
              i -> [w767]
              stop <- w786 stop-if-true
              n327 = Equal To 0?(x=w767) -> (x = 0?=w764:bool)
              n328 = property on="Transducer" class="Ring (strict)"("Value"=w773) -> ()  [unwired: 2 in, 2 out]
              n329 = And(x=w766, y=w764) -> (x .and. y?=w765:bool)
              n330 = stacked-sequence {
                seq-local: [w813 _ _] -> [_ w961 w2547]
                seq-local: [w801 _ _] -> [_ w938 _]
                tunnel: w788 -> [_ w962 _]
                tunnel: w787 -> [_ w933 _]
                tunnel: [_ w960 _] -> w786
                tunnel: w768 -> [w800 w943 w2545]
                tunnel: [_ w959 _] -> w785
                tunnel: w782 -> [_ w954 _]
                tunnel: w774 -> [w794 w942 _]
                tunnel: [_ w953 _] -> w784
                tunnel: [_ w951 _] -> w783
                tunnel: w781 -> [_ w950 _]
                tunnel: w773 -> [_ w944 _]
                tunnel: w780 -> [_ w949 _]
                tunnel: [_ w948 _] -> w779
                tunnel: [_ w947 _] -> w778
                tunnel: w777 -> [_ w946 _]
                tunnel: w776 -> [_ w934 _]
                tunnel: w775 -> [_ w945 _]
                tunnel: w765 -> [w806 _ _]
                tunnel: w772 -> [w799 w937 _]
                tunnel: [_ w941 _] -> w771
                tunnel: w770 -> [w793 w940 _]
                tunnel: w769 -> [_ w939 _]
                tunnel: w763 -> [_ w936 _]
                tunnel: w762 -> [_ w935 _]
                tunnel: w761 -> [_ _ _]
                tunnel: w760 -> [_ w928 _]
                tunnel: w759 -> [w791 w932 _]
                tunnel: w758 -> [_ w931 _]
                tunnel: w757 -> [_ w930 _]
                tunnel: [_ w929 _] -> w756
                tunnel: w755 -> [w790 w927 _]
                tunnel: w754 -> [_ w925 _]
                frame #0 {
                  # "Scale Parameters"
                  # "This is the case for SMAC fast motion. Needs to be able to adjust scan parameters on the fly."
                  n331 = Unbundle By Name(w800) -> ("Samp Rate (Hz)"=w805:dbl)
                  n332 = expression code="x*1E-6"(w805) -> (w802:dbl)
                  n333 = call "BP FilterCoeffs.vi"("sample rate MHz"=w802, "Filter Prams"="Filter Prams") -> ("FIR Windowed Coefficients"=w804:dbl[])  [unwired: 4 in]
                  n334 = Bundle("FIR Windowed Coefficients"=w804, "Filter Prams"="Filter Prams") -> (w801:T62)  [unwired: 1 in]
                  n335 = Unbundle By Name(w800) -> ("Main Digitizer"=w811:T31, "Dig Config"=w810:T32, "Trigger Settings"=w808:T63, "Voltage Scale"=w807:dbl)
                  n336 = flat-sequence {
                    tunnel: w799 -> [w821]
                    tunnel: w806 -> [w822]
                    tunnel: w794 -> [w818]
                    tunnel: w793 -> [w823]
                    tunnel: [w823] -> w798
                    tunnel: [w816] -> w797
                    tunnel: [w822] -> w796
                    tunnel: [w821] -> w795
                    tunnel: [w817] -> w792
                    tunnel: w791 -> [w817]
                    tunnel: w790 -> [w815]
                    tunnel: [w814] -> w789
                    tunnel: w798 -> [w829]
                    tunnel: w797 -> [w828]
                    tunnel: w796 -> [w827]
                    tunnel: w795 -> [w826]
                    tunnel: w792 -> [w825]
                    tunnel: w789 -> [w824]
                    frame #0 {
                      n337 = Decrement(x=w815) -> (x-1=w814:i32)
                      n338 = call "FindLocation.vi"("Motion Settings"=w818, "Wait for Motion Complete"=TRUE) -> ("location (mm)"=w820:dbl[])  [unwired: 1 in, 3 out]
                      n339 = Index Array(array=w820, index=w814) -> (element=w816:dbl)
                      n340 = property on="Position (mm)" class="DigNum (strict)"("Value"=w816) -> ()  [unwired: 2 in, 2 out]
                    }
                    frame #1 {
                      n341 = case shown="\"WCM Main\", Default" w826 {
                        selector: w826 -> [_ w830]
                        tunnel: w829 -> [_ w834]
                        tunnel: w828 -> [_ w836]
                        tunnel: w827 -> [_ w833]
                        tunnel: w825 -> [_ w832]
                        tunnel: w824 -> [_ w831]
                        frame "WCM Main", Default {
                        }
                        frame "Hawaii", "Stony Brook" {
                          n342 = case shown="True" w833 {
                            tunnel: w830 -> [_ w846]
                            frame False {
                            }
                            frame True {
                              n343 = case shown="\"Stony Brook\"" w846 {
                                tunnel: [0.0 ("Z Scale.Range:Maximum") 0.0 ("Z Scale.Range:Maximum")] -> w849
                                frame "Stony Brook" {
                                }
                                frame "Hawaii", Default {
                                }
                              }
                              n344 = property on="dB Range" class="Slide (strict)"("Maximum"=w849) -> ("Value"=w848:cluster{dbl, dbl})  [unwired: 2 in, 2 out]
                              n345 = Unbundle(w848) -> (w847:dbl)  [unwired: 1 out]
                              n346 = property on="Real Time Image" class="IntGraph (strict)"("ZScale.Maximum"=w849, "ZScale.Minimum"=w847) -> ()  [unwired: 2 in, 2 out]
                              "End Point Counter" <- u32 0 ("End Point Counter")
                            }
                          }
                          n347 = property on="Acquisition Volume (mm)" class="Arr (strict)"("Value"=w834) -> ()  [unwired: 2 in, 2 out]
                          n348 = Index Array(array=w834, index=w831) -> (element=w835:dbl)
                          n349 = expression code="x/2"(w835) -> (w837:dbl)
                          n350 = Subtract(x=w836, y=w837) -> (x-y=w839:dbl)
                          n351 = Add(x=w836, y=w837) -> (x+y=w838:dbl)
                          n352 = property on="Position (mm) (Pt1)" class="DigNum (strict)"("Value"=w839) -> ()  [unwired: 2 in, 2 out]
                          n353 = property on="Position (mm) (Pt2)" class="DigNum (strict)"("Value"=w838) -> ()  [unwired: 2 in, 2 out]
                          n354 = case shown="\"Dual Transducer\"" w832 {
                            tunnel: w833 -> [_ w841]
                            tunnel: w830 -> [_ w840]
                            frame "Therapy With Scan", Default {
                            }
                            frame "Dual Transducer" {
                              n355 = case shown="True" w841 {
                                tunnel: w840 -> [_ w842]
                                frame False {
                                }
                                frame True {
                                # "Force File Name Generation"
                                n356 = call "PatientSpecificFileNameGen2.vi"("Location"=w842, "Add to Database"=FALSE, "Auto Increment"=TRUE) -> ("PatientFileName"=w843:string)  [unwired: 1 in, 1 out]
                                n357 = property on="File Name" class="Str"("Value"=w843) -> ()  [unwired: 2 in, 2 out]
                                }
                              }
                            }
                          }
                        }
                      }
                    }
                  }
                  n358 = case shown="\"Acqiris Digitizer\"" w811 {
                    tunnel: w810 -> [w858 _ _ _]
                    tunnel: [_ _ w907 _] -> w813
                    tunnel: w800 -> [w855 w879 w905 w912]
                    tunnel: w808 -> [w853 w882 w895 _]
                    tunnel: T51 {"Voltage Scale"=0.0, "Offset"=0.0, "Coupling"=3} ("V scale") -> [w856 w881 w910 _]
                    tunnel: w807 -> [w854 w876 w894 _]
                    frame "Acqiris Digitizer" {
                      n359 = Unbundle By Name(w855) -> ("Digitizer ID Cluster.Acqiris/Alazar/SP ID"=w857:u32[])
                      n360 = disable-structure shown="Disabled" {
                        disable-tunnel: w858 -> [w872 _]
                        disable-tunnel: w857 -> [w869 _]
                        disable-tunnel: w856 -> [w863 _]
                        disable-tunnel: w855 -> [w861 _]
                        disable-tunnel: w854 -> [w860 _]
                        disable-tunnel: w853 -> [w859 _]
                        frame Disabled {
                          n361 = Index Array(array=w869) -> (element=w868:u32)  [unwired: 1 in]
                          n362 = Index Array(array=w869, index=1) -> (element=w870:u32)
                          n363 = call "conSamp.vi"("Digitizer Settings"=w861, "InstrumentID"=w868) -> ("error out"=w865:errorcluster, "DUP ID"=w867:u32)  [unwired: 2 in]
                          n364 = case shown="\"2 Chans w/ 2 Acqiris\"" w872 {
                            tunnel: w870 -> [_ w874]
                            tunnel: w861 -> [_ w873]
                            frame "Single channel", Default {
                            }
                            frame "2 Chans w/ 2 Acqiris" {
                              n365 = call "conSamp.vi"("Digitizer Settings"=w873, "InstrumentID"=w874) -> ()  [unwired: 2 in, 2 out]
                            }
                          }
                          n366 = call "conTrig.vi"("error in"=w865, "Voltage Scale"=w860, "Trigger"=w859, "InstrumentID"=w867) -> ("error out"=w864:errorcluster, "dup id"=w866:u32)  [unwired: 1 in]
                          n367 = Bundle(cluster=w863, "Voltage Scale"=w860) -> (w862:T51)  [unwired: 2 in]
                          n368 = call "conVert.vi"("InstrumentID"=w866, "V scale"=w862, "error in"=w864) -> ()  [unwired: 3 in, 2 out]
                        }
                        frame Enabled {
                        }
                      }
                    }
                    frame "NI Digitizer", Default {
                      n369 = Unbundle By Name(w879) -> ("Digitizer ID Cluster.NI Instr Handles"=w888:refnum<k15>[])
                      n370 = Unbundle By Name(w879) -> ("rf points per line"=w877:i32, "lines per plane"=w878:i32)
                      n371 = Index Array(array=w888) -> (element=w887:refnum<k15>)  [unwired: 1 in]
                      n372 = property class="niScope"(reference=w887, "Min Number of Points"=w877, "Number of Records"=w878, "Enable Records > Memory"=TRUE) -> (reference out=w891:refnum<k15>, error out=w890:errorcluster)  [unwired: 1 in]
                      n373 = call "NI conSamp.vi"("error in"=w890, "Digitizer Settings"=w879, "InstrumentID"=w891) -> ("error out"=w884:errorcluster, "DUP ID"=w885:refnum<k15>)  [unwired: 1 in]
                      n374 = call "NIconTrig.vi"("error in"=w884, "Trigger"=w882, "InstrumentID"=w885) -> ("error out"=w883:errorcluster, "dup id"=w886:refnum<k15>)  [unwired: 1 out]
                      n375 = Bundle(cluster=w881, "Voltage Scale"=w876) -> (w880:T51)  [unwired: 2 in]
                      n376 = call "NIconVert.vi"("InstrumentID"=w886, "V scale"=w880, "error in"=w883) -> ("error out"=w875:errorcluster)  [unwired: 1 in, 3 out]
                      n377 = local write "error out"(w875) -> ()
                    }
                    frame "AlazarTech" {
                      w901 = u32 1 items=["A"=1, "B"=2, "A + B"=3, "C"=4, "A + C"=5, "A + B"=6, "D"=8, "A + D"=9, "B + D"=10, "C + D"=12, "A + B + C + D"=15] ("Channel")
                      n378 = Unbundle By Name(w905) -> ("rf points per line"=w903:i32, "lines per plane"=w902:i32, "Digitizer ID Cluster.Acqiris/Alazar/SP ID"=w900:u32[])
                      n379 = Index Array(array=w900) -> (element=w896:u32)  [unwired: 1 in]
                      n380 = call "Alazar_conTrig - ATS-SDK.vi"("Trigger"=w895, "Voltage Scale"=w894, "Handle in"=w896) -> ("error out"=w893:errorcluster, "Handle_Out"=w899:u32)  [unwired: 2 in]
                      n381 = Bundle(cluster=w910, "Voltage Scale"=w894) -> (w898:T51)  [unwired: 2 in]
                      n382 = call "Alazar_ChannelConfig - ATS-SDK.vi"("error in (no error)"=w893, "V scale"=w898, "Handle in"=w899) -> ("error out"=w892:errorcluster, "Handle_Out"=w897:u32)  [unwired: 2 in, 1 out]
                      n383 = call "AlazarAcqPrep - ATS-SDK.vi"("Handle"=w897, "Digitizer Settings"=w905, "Enable Trigger Enable"=TRUE, "Channel"=w901, "BuffCount"=4, "rf points per line"=w903, "error in (no error)"=w892, "rf lines per buffer"=w902) -> ("Handle Out"=w908:u32, "AlazarCluster"=w907:T64, "error out"=w909:errorcluster)  [unwired: 4 in, 1 out]
                      n384 = call "AlazarStartCapture.vi"("Handle"=w908, "error in (no error)"=w909) -> ()  [unwired: 3 out]
                    }
                    frame "LeCroy" {
                      w922 = FALSE ("Continuous Acquisition Mode (T: On)")
                      w913 = u16 2 items=["RealTime", "RIS", "Sequence", "Roll", "WaveStream"] ("Sample Mode (0: RealTime)")
                      n385 = Unbundle By Name(w912) -> ("Digitizer ID Cluster.LeCroy VISA"=w915:refnum<visa-resource-name>, "Digitizer delay (us)"=w914:dbl, "lines per plane"=w911:i32)
                      n386 = call <instrlib>:"Configure Continuous Acquisition.vi"("Auto Trigger Enabled (T: Normal)"=w922, "Continuous Acquisition Mode (T: On)"=w922, "VISA resource name"=w915) -> ("error out"=w923:errorcluster, "VISA resource name out"=w924:refnum<visa-resource-name>)  [unwired: 7 in]
                      n387 = expression code="-1E-6*x"(w914) -> (w920:dbl)
                      n388 = call <instrlib>:"Configure Sample Mode.vi"("error in (no error)"=w923, "Number of Segments (2)"=w911, "Sample Mode (0: RealTime)"=w913, "VISA resource name"=w924) -> ("error out"=w918:errorcluster, "VISA resource name out"=w919:refnum<visa-resource-name>)  [unwired: 6 in]
                      n389 = Number To Exponential String(number=w920) -> (E-format string=w921:string)  [unwired: 3 in]
                      n390 = Concatenate Strings("TRDL " ("Write Buffer"), w921) -> (w917:string)
                      n391 = call <instrlib>:"Write.vi"("error in (no error)"=w918, "Write Buffer"=w917, "VISA resource name"=w919) -> ()  [unwired: 6 in, 3 out]
                    }
                  }
                  n392 = local read "distance?"() -> (w809:bool)
                  n393 = property on="distance?" class="Bool (strict)"("Val(Sgnl)"=w809) -> ()  [unwired: 2 in, 2 out]
                }
                frame #1 {
                  w926 = 0.1  # Scan Size Inc
                  n394 = Obtain Notifier ("Stop Scan")(name (unnamed)="ResetScan", notification data type=TRUE) -> (notifier out=w956:refnum<notifier>)  [unwired: 2 in, 2 out]
                  n395 = while {
                    tunnel: w962 -> [w1000]
                    tunnel: w939 -> [w999]
                    tunnel: w954 -> [w997]
                    tunnel: [w995] -> w960
                    shift-right: [w964] -> w959
                    shift-left: w943 -> [w994]
                    tunnel: w956 -> [w993]
                    shift-right: [w991] -> w953
                    shift-left: w942 -> [w992]
                    shift-right: [w989] -> _
                    shift-left: _ -> [w990]
                    shift-right: [w987] -> _
                    shift-left: TRUE ("No data") -> [w988]
                    tunnel: [w985] -> w951
                    tunnel: w937 -> [w984]
                    tunnel: w950 -> [w983]
                    shift-right: [w981] -> w948
                    shift-left: w944 -> [w982]
                    tunnel: w949 -> [w980]
                    shift-right: [w978] -> w947
                    shift-left: w936 -> [w979]
                    shift-right: [w976] -> w941
                    shift-left: w940 -> [w977]
                    tunnel: w946 -> [w975]
                    tunnel: w934 -> [w974]
                    tunnel: w945 -> [w973]
                    tunnel: w935 -> [w972]
                    shift-right: [w971] -> _
                    shift-left: w938 -> [w986]
                    tunnel: w933 -> [w970]
                    tunnel: w932 -> [w969]
                    tunnel: w931 -> [w968]
                    tunnel: w928 -> [w967]
                    tunnel: w927 -> [w966]
                    tunnel: w926 -> [w965]
                    tunnel: w925 -> [w963]
                    i -> [w1001]
                    stop <- w996 stop-if-true
                    n396 = event shown="[9] \"Stop Motor\": Value Change" {
                      selector: _ -> [_ _ _ _ _ _ _ _ _ _ _ _ _ _ _ _ _ _ _ _ _ _ _ _ _ _ _ _ _ _ _ _ _ _ _ _ _]
                      dyn-events: _ -> [_ _ _ _ _ _ _ _ _ _ _ _ _ _ _ _ _ _ _ _ _ _ _ _ _ _ _ _ _ _ _ _ _ _ _ _ _]
                      timeout: 80 -> [_ _ _ _ _ _ _ _ _ _ _ _ _ _ _ _ _ _ _ _ _ _ _ _ _ _ _ _ _ _ _ _ _ _ _ _ _]
                      tunnel: w1001 -> [w1022 _ _ _ _ _ _ _ _ _ _ _ _ _ _ _ _ _ _ _ _ _ _ _ _ _ _ _ _ _ _ _ _ _ _ _ _]
                      tunnel: [_ _ _ _ _ _ _ _ _ _ w1568 w1655 w1670 _ w1699 _ _ _ _ _ _ w1909 _ _ _ _ w2032 w2088 w2127 w2155 _ _ _ _ w2362 w2391 w2508] -> w996
                      tunnel: w1000 -> [w1021 _ _ _ _ _ _ _ _ _ _ _ _ _ _ _ _ _ _ _ _ _ _ _ _ _ _ _ _ _ _ _ _ _ _ _ _]
                      tunnel: w999 -> [w1020 _ _ _ _ _ _ _ _ _ _ _ _ _ _ _ _ _ _ _ _ _ _ _ _ _ _ _ _ _ _ _ _ _ _ _ _]
                      tunnel: w997 -> [w1019 _ _ _ _ _ _ _ _ _ _ _ _ _ _ _ _ _ _ _ _ _ _ _ _ _ _ _ _ _ _ _ _ _ _ _ _]
                      tunnel: [_ _ _ _ _ _ _ _ _ _ w1568 w1655 w1670 _ w1699 _ _ _ _ _ _ w1909 _ _ _ _ w2032 w2088 w2127 w2155 _ _ _ _ w2362 w2391 w2508] -> w995
                      tunnel: w994 -> [w1003 w1128 w1210 w1338 w1376 w1383 w1467 w1512 w1533 w1551 w1589 w1654 w1677 w1689 w1714 w1777 w1786 w1804 w1842 w1871 w1883 w1912 w1934 w1957 w1978 w2022 w2064 w2097 w2137 w2157 w2289 w2301 w2316 w2334 w2367 w2394 w2511]
                      tunnel: [w1003 w1124 w1210 w1338 w1376 w1383 w1467 w1495 w1533 w1551 w1569 w1631 w1677 w1689 w1713 w1777 w1786 w1804 w1842 w1871 w1883 w1912 w1934 w1957 w1978 w2022 w2064 w2097 w2137 w2160 w2289 w2301 w2316 w2334 w2367 w2393 w2511] -> w964
                      tunnel: w993 -> [_ _ _ _ _ _ _ _ _ _ w1592 w1656 w1669 _ w1715 _ _ _ _ _ _ w1913 _ _ _ _ w2031 w2089 w2128 w2156 _ _ _ _ w2363 w2402 w2510]
                      tunnel: w992 -> [w1018 w1129 w1209 w1354 w1375 w1382 w1457 w1511 w1532 w1542 w1588 w1649 w1676 w1684 w1712 w1776 w1785 w1803 w1841 w1870 w1894 w1911 w1933 w1956 w1964 w2021 w2023 w2095 w2136 w2158 w2288 w2300 w2315 w2333 w2366 w2396 w2505]
                      tunnel: [w1018 w1123 w1209 w1354 w1375 w1385 w1457 w1511 w1530 w1549 w1571 w1640 w1676 w1687 w1711 w1776 w1785 w1803 w1841 w1870 w1894 w1911 w1933 w1956 w1964 w2021 w2056 w2095 w2130 w2159 w2288 w2300 w2315 w2333 w2366 w2392 w2505] -> w991
                      tunnel: w990 -> [w1017 w1130 w1216 w1353 w1374 w1384 w1466 w1513 w1529 w1548 w1591 w1657 w1675 w1695 w1716 w1775 w1788 w1802 w1840 w1869 w1896 w1915 w1932 w1955 w1977 w2020 w2063 w2096 w2135 w2162 w2287 w2299 w2314 w2332 w2365 w2403 w2509]
                      tunnel: [w1016 w1130 w1216 w1353 w1374 w1384 w1466 w1513 w1529 w1548 w1591 w1657 w1675 w1695 w1716 w1775 w1788 w1802 w1840 w1869 w1896 w1915 w1932 w1955 w1977 w2020 w2063 w2096 w2135 w2162 w2287 w2299 w2314 w2332 w2365 w2403 w2509] -> w989
                      tunnel: w988 -> [w1015 _ _ _ _ _ _ _ _ _ _ _ _ _ _ _ _ _ _ _ _ _ _ _ _ _ _ _ _ _ _ _ _ _ _ _ _]
                      tunnel: [w1014 _ _ _ _ _ _ _ _ _ _ _ _ _ _ _ _ _ _ _ _ _ _ _ _ _ _ _ _ _ _ _ _ _ _ _ _] -> w987
                      tunnel: w986 -> [w1013 w1120 w1211 w1332 w1369 w1377 w1462 w1507 w1525 w1544 w1574 w1633 w1671 w1693 w1704 w1769 w1778 w1797 w1833 w1866 w1885 w1907 w1919 w1942 w1971 w2010 w2040 w2091 w2131 w2144 w2281 w2294 w2306 w2321 w2353 w2387 w2499]
                      tunnel: [_ _ _ _ _ _ _ _ _ _ _ _ _ _ _ _ _ _ _ _ _ _ _ _ _ _ _ _ _ _ _ _ _ _ _ w2391 w2508] -> w985
                      tunnel: w984 -> [w1005 w1121 w1215 _ _ _ _ w1501 _ _ _ _ _ _ _ _ _ _ _ _ _ _ _ _ _ w2006 _ _ _ w2151 w2282 w2295 _ w2324 w2354 w2381 w2501]
                      tunnel: w983 -> [_ _ _ _ w1373 _ _ _ _ _ _ _ _ _ _ _ _ _ _ _ _ _ _ _ _ _ _ _ _ _ _ _ _ _ _ _ _]
                      tunnel: w982 -> [w1010 w1126 w1214 w1335 w1372 w1381 w1465 w1508 w1528 w1547 w1587 w1641 w1674 w1685 w1709 w1774 w1781 w1798 w1832 w1865 w1893 w1910 w1931 w1954 w1976 w2019 w2051 w2094 w2134 _ w2286 w2298 w2313 w2331 w2364 w2400 w2507]
                      tunnel: [w1010 w1126 w1214 w1335 w1372 w1381 w1465 w1508 w1528 w1547 w1587 w1641 w1674 w1685 w1708 w1774 w1781 w1798 w1832 w1865 w1893 w1910 w1931 w1954 w1976 w2019 w2051 w2094 w2134 w2150 w2286 w2298 w2313 w2331 w2364 w2400 w2507] -> w981
                      tunnel: w980 -> [_ _ w1218 _ _ _ _ _ _ _ w1570 _ _ _ _ _ _ _ _ _ _ _ _ _ _ _ _ _ _ _ _ _ _ _ _ _ _]
                      tunnel: w979 -> [w1004 w1127 w1217 w1334 w1371 w1380 w1464 w1509 w1527 w1546 w1575 w1639 w1673 w1692 w1702 w1773 w1783 w1800 w1831 w1864 w1891 w1908 w1930 w1953 w1975 w2018 w2046 w2093 w2133 w2149 w2285 w2297 w2312 w2320 w2348 w2397 w2500]
                      tunnel: [w1004 w1127 w1217 w1334 w1371 w1380 w1464 w1505 w1527 w1546 w1572 w1638 w1673 w1688 w1701 w1773 w1779 w1799 w1828 w1862 w1890 w1908 w1930 w1953 w1975 w2018 w2046 w2093 w2133 w2152 w2285 w2297 w2312 w2320 w2351 w2395 w2500] -> w978
                      tunnel: w977 -> [w1008 _ w1213 w1333 w1370 w1379 w1463 w1510 w1526 w1545 w1590 w1642 w1672 w1694 w1710 w1772 w1787 w1801 w1839 w1868 w1895 w1914 w1924 w1944 w1974 w2017 w2045 w2092 w2132 w2146 w2284 w2296 w2311 w2330 w2349 w2399 w2503]
                      tunnel: [w1009 w1117 w1213 w1333 w1370 w1379 w1463 w1496 w1526 w1545 w1590 w1642 w1672 w1694 w1710 w1772 w1787 w1801 w1839 w1868 w1895 w1914 w1921 w1943 w1974 w2017 w2041 w2092 w2132 w2146 w2284 w2296 w2311 w2330 w2352 w2398 w2502] -> w976
                      tunnel: w975 -> [_ _ _ _ _ _ _ _ _ _ w1586 w1637 _ _ _ _ _ _ _ _ w1892 _ _ _ _ _ _ _ _ w2153 _ _ _ _ _ _ _]
                      tunnel: w974 -> [_ _ _ _ _ _ w1430 _ _ _ _ _ _ _ w1705 w1770 _ _ _ _ _ _ _ _ _ _ _ _ _ w2145 _ _ _ _ _ w2388 _]
                      tunnel: w973 -> [_ _ w1212 _ _ w1378 w1439 w1497 _ _ _ w1636 _ _ _ _ _ _ _ _ _ _ _ _ _ _ w2025 _ _ w2140 _ _ _ _ _ w2384 _]
                      tunnel: w972 -> [_ _ _ _ _ _ _ _ _ _ _ _ _ _ w1706 _ _ _ _ _ _ _ _ _ _ _ _ _ _ _ _ _ _ _ _ _ _]
                      tunnel: [w1013 w1120 w1211 w1332 w1369 w1377 w1462 w1507 w1525 w1544 w1574 w1633 w1671 w1693 w1704 w1769 w1778 w1797 w1833 w1866 w1886 w1907 w1919 w1942 w1971 w2010 w2040 w2091 w2131 w2144 w2281 w2294 w2306 w2321 w2353 w2387 w2499] -> w971
                      tunnel: w970 -> [_ _ _ _ _ _ _ _ _ _ _ _ _ _ _ _ _ _ _ _ _ _ _ _ _ _ _ w2090 _ w2143 _ _ _ _ _ _ _]
                      tunnel: w969 -> [_ _ _ _ _ _ w1461 _ _ _ w1573 w1632 _ _ w1700 _ _ w1794 w1829 w1863 w1882 _ _ _ _ _ _ _ _ _ _ _ _ _ _ w2382 _]
                      tunnel: w968 -> [_ _ _ _ _ _ _ _ _ _ _ _ _ _ _ _ _ _ _ _ _ _ _ _ _ _ _ _ _ _ _ _ _ _ _ w2386 _]
                      tunnel: w967 -> [_ _ _ _ _ _ _ _ _ _ _ _ _ _ w1703 _ _ _ _ _ _ _ _ _ _ _ w2035 _ _ _ _ _ _ _ _ w2383 _]
                      tunnel: w966 -> [_ _ _ _ _ _ _ _ _ _ _ _ _ _ _ _ _ _ _ _ _ _ _ _ w1962 _ w2037 _ _ w2142 _ _ _ _ _ w2385 _]
                      tunnel: w965 -> [_ w1116 _ _ _ _ _ w1502 _ _ _ _ _ _ _ _ _ _ _ _ _ _ w1916 w1939 _ _ _ _ _ _ _ _ _ _ _ w2380 _]
                      tunnel: w963 -> [_ _ _ _ _ _ _ _ _ _ _ _ _ _ _ _ _ w1793 _ _ _ _ _ _ _ _ _ _ _ w2138 _ _ _ _ _ _ _]
                      event Timeout {
                        n397 = event-data() -> ()  [unwired: 1 in, 2 out]
                        n398 = Dequeue Element(queue=w1019) -> (element=w1012:T42, timed out?=w1006:bool)  [unwired: 2 in, 2 out]
                        n399 = Unbundle(w1012) -> (w1007:bool)  [unwired: 4 out]
                        n400 = Or(x=w1007, y=w1006) -> (x .or. y?=w1011:bool)
                        "No data" <- w1011
                        n401 = case shown="False" w1011 {
                          tunnel: w1022 -> [w1036 _]
                          tunnel: w1021 -> [w1035 _]
                          tunnel: w1020 -> [w1034 _]
                          tunnel: w1012 -> [w1033 _]
                          tunnel: w1003 -> [w1032 _]
                          tunnel: w1018 -> [w1031 _]
                          tunnel: w1017 -> [w1030 w1111]
                          tunnel: [w1029 w1111] -> w1016
                          tunnel: w1015 -> [w1028 _]
                          tunnel: [w1027 _] -> w1014
                          tunnel: w1013 -> [w1026 _]
                          tunnel: [w1024 w1110] -> w1009
                          tunnel: w1008 -> [w1025 w1110]
                          tunnel: w1005 -> [w1023 _]
                          frame False {
                            n402 = stacked-sequence {
                              tunnel: w1036 -> [w1048 w1082 _ _]
                              tunnel: w1035 -> [_ w1081 _ _]
                              tunnel: w1034 -> [w1047 _ _ _]
                              tunnel: w1033 -> [w1045 _ _ _]
                              tunnel: w1032 -> [w1044 _ _ _]
                              tunnel: w1031 -> [w1043 _ _ _]
                              tunnel: w1030 -> [_ _ _ w1109]
                              tunnel: [_ _ _ w1108] -> w1029
                              tunnel: w1028 -> [_ _ _ w1102]
                              tunnel: [_ _ _ FALSE ("No data")] -> w1027
                              tunnel: w1026 -> [w1038 _ _ _]
                              tunnel: w1025 -> [_ _ w1096 _]
                              tunnel: [_ _ w1096 _] -> w1024
                              tunnel: w1023 -> [_ _ _ _]
                              frame #0 {
                                # "Slightly faster version to read data"
                                # "Get and display data"
                                n403 = Unbundle(w1045) -> ("gain"=w1050:dbl, "Array"=w1041:i16[][], "gain 2"=w1049:dbl)  [unwired: 2 out]
                                n404 = case shown="0, Default" "Type of Mean" {
                                tunnel: w1041 -> [w1052 w1055]
                                tunnel: [w1052 w1054] -> w1040
                                tunnel: w1038 -> [_ w1053]
                                frame 0, Default {
                                }
                                frame 4 {
                                n405 = call "BP FilterI16_Fast.vi"("Filter"=w1053, "Array in"=w1055) -> ("Filtered X"=w1054:dbl[][])  [unwired: 4 in]
                                }
                                }
                                n406 = case shown="1" "Display mode" {
                                tunnel: [w1063 w1067 w1075 w1076 w1079] -> w1037
                                tunnel: w1040 -> [w1064 w1066 w1075 w1077 w1080]
                                tunnel: w1047 -> [_ w1065 _ w1078 _]
                                frame 0, Default {
                                n407 = Absolute Value(x=w1064) -> (abs(x)=w1063:dbl[][])
                                }
                                frame 1 {
                                n408 = for {
                                tunnel: [w1070] -> w1067 mode=indexing
                                tunnel: w1066 -> [w1069] mode=indexing
                                tunnel: w1065 -> [w1068]
                                workers-P: _ -> [_]
                                n409 = for {
                                tunnel: [w1074] -> w1070 mode=indexing
                                tunnel: w1069 -> [w1073] mode=indexing
                                tunnel: w1068 -> [w1071]
                                n410 = Absolute Value(x=w1073) -> (abs(x)=w1072:dbl)
                                n411 = Index Array(array=w1071, index=w1072) -> (element=w1074:sgl)
                                }
                                }
                                }
                                frame 2 {
                                }
                                frame 3 {
                                n412 = call "AvisoSectorConvert.vi"("Log Lookup"=w1078, "Raw In"=w1077) -> ("Sector out"=w1076:dbl[][])  [unwired: 9 in]
                                }
                                frame 10 {
                                n413 = expression code="log(abs(x))"(w1080) -> (w1079:dbl[][])
                                }
                                }
                                "Real Time Image" <- w1037
                                n414 = Increment(x=w1048) -> (x+1=w1051:i32)
                                "Frame #" <- w1051
                                n415 = case shown="True" "*.eye" {
                                selector: "*.eye" -> [_ w1056]
                                tunnel: w1051 -> [_ w1062]
                                tunnel: w1050 -> [_ w1061]
                                tunnel: w1049 -> [_ w1060]
                                tunnel: w1041 -> [_ w1059]
                                tunnel: w1044 -> [_ w1058]
                                tunnel: w1043 -> [_ w1057]
                                frame False {
                                }
                                frame True {
                                n416 = call "SaveEYE_RT_Single.vi"("Motion Settings"=w1057, "gain"=w1061, "*.eye"=w1056, "Digitizer Settings"=w1058, "gain 2 Ch"=w1060, "Frame"=w1062, "Data"=w1059) -> ()  [unwired: 5 in]
                                }
                                }
                              }
                              frame #1 {
                                n417 = case shown="True" "BMP?" {
                                tunnel: w1082 -> [_ w1086]
                                tunnel: w1081 -> [_ w1085]
                                frame False {
                                }
                                frame True {
                                n418 = invoke on="Real Time Image" class="IntGraph (strict)" method="Get Image"("image depth"=24) -> ("image data"=w1087:T65)  [unwired: 5 in, 5 out]
                                n419 = call <vilib>:"Unflatten Pixmap.vi"("image data"=w1087) -> ("24-bit pixmap"=w1088:u32[][])  [unwired: 10 out]
                                n420 = call "NumberFileName.vi"("String"=".bmp", "File number"=w1086, "file name"="Movie Name") -> ("Numbered File"=w1092:string)  [unwired: 1 in]
                                n421 = To Unsigned Byte Integer(number=w1088) -> (unsigned 8bit integer=w1089:u8[][])
                                n422 = call <vilib>:"Flatten Pixmap.vi"("colors"=u32[] [0, 0, 65793, 131586, 197379, 263172, 328965, 394758, 460551, 526344, 592137, 657930, 723723, 789516, 855309, 921102, 986895, 1052688, 1118481, 1184274, 1250067, 1315860, 1381653, 1447446, 1513239, 1579032, 1644825, 1710618, 1776411, 1842204, 1907997, 1973790, 2039583, 2105376, 2171169, 2236962, 2302755, 2368548, 2434341, 2500134, 2565927, 2631720, 2697513, 2763306, 2829099, 2894892, 2960685, 3026478, 3092271, 3158064, 3223857, 3289650, 3355443, 3421236, 3487029, 3552822, 3618615, 3684408, 3750201, 3815994, 3881787, 3947580, 4013373, 4079166, 4144959, 4210752, 4276545, 4342338, 4408131, 4473924, 4539717, 4605510, 4671303, 4737096, 4802889, 4868682, 4934475, 5000268, 5066061, 5131854, 5197647, 5263440, 5329233, 5395026, 5460819, 5526612, 5592405, 5658198, 5723991, 5789784, 5855577, 5921370, 5987163, 6052956, 6118749, 6184542, 6250335, 6316128, 6381921, 6447714, 6513507, 6579300, 6645093, 6710886, 6776679, 6842472, 6908265, 6974058, 7039851, 7105644, 7171437, 7237230, 7303023, 7368816, 7434609, 7500402, 7566195, 7631988, 7697781, 7763574, 7829367, 7895160, 7960953, 8026746, 8092539, 8158332, 8224125, 8289918, 8355711, 8421504, 8487297, 8553090, 8618883, 8684676, 8750469, 8816262, 8882055, 8947848, 9013641, 9079434, 9145227, 9211020, 9276813, 9342606, 9408399, 9474192, 9539985, 9605778, 9671571, 9737364, 9803157, 9868950, 9934743, 10000536, 10066329, 10132122, 10197915, 10263708, 10329501, 10395294, 10461087, 10526880, 10592673, 10658466, 10724259, 10790052, 10855845, 10921638, 10987431, 11053224, 11119017, 11184810, 11250603, 11316396, 11382189, 11447982, 11513775, 11579568, 11645361, 11711154, 11776947, 11842740, 11908533, 11974326, 12040119, 12105912, 12171705, 12237498, 12303291, 12369084, 12434877, 12500670, 12566463, 12632256, 12698049, 12763842, 12829635, 12895428, 12961221, 13027014, 13092807, 13158600, 13224393, 13290186, 13355979, 13421772, 13487565, 13553358, 13619151, 13684944, 13750737, 13816530, 13882323, 13948116, 14013909, 14079702, 14145495, 14211288, 14277081, 14342874, 14408667, 14474460, 14540253, 14606046, 14671839, 14737632, 14803425, 14869218, 14935011, 15000804, 15066597, 15132390, 15198183, 15263976, 15329769, 15395562, 15461355, 15527148, 15592941, 15658734, 15724527, 15790320, 15856113, 15921906, 15987699, 16053492, 16119285, 16185078, 16250871, 16316664, 16382457, 16448250, 16514043, 16579836, 16645629, 16448250] ("Array 2"), "8-bit pixmap"=w1089) -> ("image data"=w1090:T65)  [unwired: 4 in, 5 out]
                                n423 = Build Path(base path=w1085, name or relative path=w1092) -> (appended path=w1093:path)
                                n424 = call <vilib>:"Write BMP File.vi"("image data"=w1090, "path to BMP file"=w1093) -> ()  [unwired: 1 in, 9 out]
                                }
                                }
                              }
                              frame #2 {
                                n425 = property class="VI"() -> (reference out=w1098:refnum<vi>, "Front Panel.IsFrontmost"=w1097:bool)  [unwired: 2 in, 1 out]
                                n426 = case shown="False" w1097 {
                                tunnel: w1098 -> [w1099 _]
                                frame False {
                                n427 = property class="VI"(reference=w1099, "Front Panel.IsFrontmost"=TRUE) -> ()  [unwired: 1 in, 2 out]
                                }
                                frame True {
                                }
                                }
                              }
                              frame #3 {
                                n428 = Tick Count (ms)() -> (millisecond timer value=w1108:u32)
                                n429 = Subtract(x=w1108, y=w1109) -> (x-y=w1104:u32)
                                n430 = To Double Precision Float(number=w1104) -> (double precision float=w1103:dbl)
                                n431 = expression code="1000/x"(w1103) -> (w1106:dbl)
                                n432 = call <vilib>:"Mean PtByPt.vi"("x"=w1106, "sample length"=30, "initialize"=w1102) -> ("mean"=→"FPS":dbl)  [unwired: 1 in, 1 out]
                              }
                            }
                          }
                          frame True {
                          }
                        }
                        n433 = call "CheckTotalSamples.vi"("Digitizer Settings"=w1003) -> ("Total Pts"=→"Total Pts":bool)  [unwired: 14 in]
                      }
                      event "Acquisition Volume (mm)": Value Change {
                        n434 = event-data() -> ("OldVal"=w1115:dbl[], "NewVal"=w1119:dbl[])  [unwired: 1 in]
                        n435 = call-poly "ModFractionPoly.vi"("Modulo Fraction"=w1116, "Input"=w1119) -> ("Output"=w1118:dbl[])  [unwired: 1 in]
                        n436 = case shown="\"Hawaii\"" w1121 {
                          tunnel: w1118 -> [w1131 w1135 w1148]
                          tunnel: [w1131 w1133 w1146] -> w1117
                          frame "WCM Main", Default {
                          }
                          frame "Stony Brook" {
                            w1132 = dbl[] [20.1, 60.1, 15.1]  # Upper Limit
                            w1134 = 1.0  # Lower Limit
                            n437 = for {
                              tunnel: w1135 -> [w1136] mode=indexing
                              tunnel: [w1141] -> w1133 mode=indexing
                              tunnel: w1134 -> [w1139]
                              tunnel: w1132 -> [w1137] mode=indexing
                              n438 = In Range and Coerce(upper limit=w1137, x=w1136, lower limit=w1139) -> (coerced(x)=w1140:dbl, In Range?=w1138:bool)
                              n439 = case shown="False" w1138 {
                                tunnel: w1140 -> [w1143 w1144]
                                tunnel: [w1142 w1144] -> w1141
                                frame False {
                                n440 = Round To Nearest(number=w1143) -> (nearest integer value=w1142:dbl)
                                }
                                frame True {
                                }
                              }
                            }
                          }
                          frame "Hawaii" {
                            w1145 = dbl[] [60.1, 60.1, 15.1]  # Upper Limit
                            w1147 = 1.0  # Lower Limit
                            n441 = for {
                              tunnel: w1148 -> [w1150] mode=indexing
                              tunnel: [w1154] -> w1146 mode=indexing
                              tunnel: w1147 -> [w1152]
                              tunnel: w1145 -> [w1149] mode=indexing
                              n442 = In Range and Coerce(upper limit=w1149, x=w1150, lower limit=w1152) -> (coerced(x)=w1153:dbl, In Range?=w1151:bool)
                              n443 = case shown="False" w1151 {
                                tunnel: w1153 -> [w1156 w1157]
                                tunnel: [w1155 w1157] -> w1154
                                frame False {
                                n444 = Round To Nearest(number=w1156) -> (nearest integer value=w1155:dbl)
                                }
                                frame True {
                                }
                              }
                            }
                          }
                        }
                        n445 = Index Array(array=w1115) -> (element=w1113:dbl)  [unwired: 1 in]
                        n446 = Index Array(array=w1117) -> (element #1=w1114:dbl, element #2=w1125:dbl, element #3=w1122:dbl)  [unwired: 3 in]
                        n447 = Subtract(x=w1114, y=w1113) -> (x-y=w1112:dbl)
                        n448 = stacked-sequence {
                          tunnel: w1129 -> [w1168 w1191 _ _]
                          tunnel: w1128 -> [w1167 _ _ _]
                          tunnel: w1114 -> [w1161 _ _ _]
                          tunnel: w1125 -> [_ w1192 _ _]
                          tunnel: [w1160 _ _ _] -> w1124
                          tunnel: [_ w1190 _ _] -> w1123
                          tunnel: w1122 -> [_ _ w1203 _]
                          tunnel: w1116 -> [_ w1185 _ _]
                          tunnel: w1112 -> [w1158 _ _ _]
                          frame #0 {
                            n449 = Unbundle By Name(w1168) -> ("Distance between\nscan lines (um)"=w1162:sgl)
                            n450 = case shown="False" "Force Symmetric?" {
                              tunnel: w1161 -> [w1169 _]
                              tunnel: w1158 -> [_ w1176]
                              frame True {
                                n451 = expression code="x/2"(w1169) -> (w1170:dbl)
                                n452 = Negate(x=w1170) -> (-x=w1173:dbl)
                                n453 = property on="Real Time Image" class="IntGraph (strict)"("Active Cursor"=u32 0, "Cursor.Cursor X"=w1173, "Active Cursor"=u32 1, "Cursor.Cursor X"=w1170) -> ()  [unwired: 2 in, 2 out]
                              }
                              frame False {
                                n454 = property on="Real Time Image" class="IntGraph (strict)"("Active Cursor"=u32 0, "Active Cursor"=u32 1) -> ("Cursor.Cursor X"=w1175:dbl, "Cursor.Cursor X"=w1174:dbl)  [unwired: 2 in, 2 out]
                                n455 = expression code="x/2"(w1176) -> (w1181:dbl)
                                n456 = Negate(x=w1181) -> (-x=w1184:dbl)
                                n457 = Add(x=w1175, y=w1184) -> (x+y=w1178:dbl)
                                n458 = Add(x=w1181, y=w1174) -> (x+y=w1177:dbl)
                                n459 = property on="Real Time Image" class="IntGraph (strict)"("Active Cursor"=u32 0, "Cursor.Cursor X"=w1178, "Active Cursor"=u32 1, "Cursor.Cursor X"=w1177) -> ()  [unwired: 2 in, 2 out]
                              }
                            }
                            n460 = expression code="x*1e3"(w1161) -> (w1166:dbl)
                            n461 = Divide(x=w1166, y=w1162) -> (x/y=w1165:dbl)
                            n462 = call "Force Odd or Even.vi"("Parity (odd)"=enum16{"Odd", "Even"}."Odd" ("Parity"), "input"=w1165) -> ("output"=w1163:i32)
                            n463 = Bundle By Name(cluster=w1167, "lines per plane"=w1163) -> (w1160:T30)
                            n464 = property on="lines per plane" class="DigNum (strict)"("Value"=w1163) -> ()  [unwired: 2 in, 2 out]
                          }
                          frame #1 {
                            n465 = Unbundle By Name(w1191) -> ("Distance between\nscan planes (um)"=w1195:sgl)
                            n466 = expression code="x/2"(w1192) -> (w1202:dbl)
                            n467 = property on="Position (mm) (Pt1)" class="DigNum (strict)"() -> ("Value"=w1198:dbl)  [unwired: 2 in, 2 out]
                            n468 = property on="Position (mm) (Pt2)" class="DigNum (strict)"() -> ("Value"=w1199:dbl)  [unwired: 2 in, 2 out]
                            n469 = expression code="x*1e3"(w1192) -> (w1194:dbl)
                            n470 = Build Array(w1198, w1199) -> (w1200:dbl[])
                            n471 = Divide(x=w1194, y=w1195) -> (x/y=w1197:dbl)
                            n472 = call-poly <vilib>:"Mean.vi"("X"=w1200) -> ("mean"=w1201:dbl)  [unwired: 1 out]
                            n473 = Subtract(x=w1201, y=w1202) -> (x-y=w1186:dbl)
                            n474 = Add(x=w1201, y=w1202) -> (x+y=w1187:dbl)
                            n475 = call "Force Odd or Even.vi"("Parity (odd)"=enum16{"Odd", "Even"}."Odd" ("Parity"), "input"=w1197) -> ("output"=w1196:i32)
                            n476 = call-poly "ModFractionPoly.vi"("Modulo Fraction"=w1185, "Input"=w1186) -> ("Output"=w1189:dbl)  [unwired: 1 in]
                            n477 = call-poly "ModFractionPoly.vi"("Modulo Fraction"=w1185, "Input"=w1187) -> ("Output"=w1188:dbl)  [unwired: 1 in]
                            n478 = Bundle By Name(cluster=w1191, "number of scan planes"=w1196) -> (w1190:T26)
                            n479 = property on="Position (mm) (Pt1)" class="DigNum (strict)"("Value"=w1189) -> ()  [unwired: 2 in, 2 out]
                            n480 = property on="Position (mm) (Pt2)" class="DigNum (strict)"("Value"=w1188) -> ()  [unwired: 2 in, 2 out]
                          }
                          frame #2 {
                            n481 = property on="Real Time Image" class="IntGraph (strict)"("Active Cursor"=u32 3) -> ("Cursor.Cursor Y"=w1207:dbl)  [unwired: 2 in, 2 out]
                            n482 = Add(x=w1203, y=w1207) -> (x+y=w1206:dbl)
                            n483 = property on="Real Time Image" class="IntGraph (strict)"("Active Cursor"=u32 4, "Cursor.Cursor Y"=w1206) -> ()  [unwired: 2 in, 2 out]
                          }
                          frame #3 {
                            n484 = property on="Initilize" class="Bool (strict)"("Val(Sgnl)"=TRUE ("Value (Signaling)")) -> ()  [unwired: 2 in, 2 out]
                          }
                        }
                        n485 = property on="Acquisition Volume (mm)" class="Arr (strict)"("Value"=w1117) -> ()  [unwired: 2 in, 2 out]
                      }
                      event "view", "distance?": Value Change {
                        n486 = event-data() -> ()  [unwired: 1 in, 1 out]
                        n487 = stacked-sequence {
                          tunnel: w1210 -> [w1221 w1287]
                          tunnel: w1218 -> [w1243 w1285]
                          tunnel: w1217 -> [_ w1288]
                          tunnel: w1214 -> [_ w1286]
                          tunnel: w1215 -> [_ w1283]
                          tunnel: w1212 -> [w1227 _]
                          tunnel: w1209 -> [w1226 w1284]
                          frame #0 {
                            n488 = property on="FixedLinesPerPlane" class="DigNum (strict)"() -> ("Value"=w1219:i32)  [unwired: 2 in, 2 out]
                            n489 = local read "Display mode"() -> (w1236:u16)
                            n490 = Bundle By Name(cluster=w1221, "lines per plane"=w1219) -> (w1220:T30)
                            n491 = call "PlotScalingParams.vi"("Motion Settings In"=w1226, "c mm/mics"=w1243, "Digitizer Settings"=w1220, "Scan Axis"=w1227) -> ("lines per plane"=w1222:i32, "Total Scan Length (mm)"=w1224:sgl, "Cluster"=w1229:T66)  [unwired: 5 in]
                            n492 = Not(x="view") -> (.not. x?=w1239:bool)
                            n493 = case shown="True" "distance?" {
                              tunnel: [w1245 w1259] -> w1228
                              tunnel: [w1248 w1258] -> w1242
                              tunnel: [w1245 w1257] -> w1241
                              tunnel: [w1248 w1256] -> w1240
                              tunnel: "view" -> [_ w1255]
                              tunnel: w1236 -> [_ w1254]
                              tunnel: w1229 -> [_ w1253]
                              tunnel: ["(points)" w1252] -> w1233
                              tunnel: ["(lines)" w1252] -> w1232
                              tunnel: [w1244 w1249] -> w1225
                              tunnel: w1224 -> [_ w1251]
                              tunnel: [w1245 w1250] -> w1223
                              tunnel: w1222 -> [w1244 _]
                              frame False {
                                w1248 = 1
                                w1245 = 0
                              }
                              frame True {
                                w1252 = "(mm)"
                                n494 = Unbundle By Name(w1253) -> ("Y Scale Offset"=w1264:dbl, "Y Scale Multi"=w1263:dbl, "X Scale Offset"=w1262:dbl, "X Scale Multi"=w1261:dbl, "Gate Distance"=w1260:dbl)
                                n495 = case shown="0, Default" w1254 {
                                tunnel: w1264 -> [w1274]
                                tunnel: w1263 -> [w1273]
                                tunnel: w1262 -> [w1272]
                                tunnel: w1255 -> [w1271]
                                tunnel: w1261 -> [w1270]
                                tunnel: [w1269] -> w1259
                                tunnel: [w1268] -> w1258
                                tunnel: [w1267] -> w1257
                                tunnel: [w1266] -> w1256
                                tunnel: w1260 -> [w1265]
                                frame 0, Default {
                                n496 = case shown="True" w1271 {
                                tunnel: [w1278 w1282] -> w1269
                                tunnel: w1274 -> [w1278 w1279]
                                tunnel: [w1277 w1281] -> w1268
                                tunnel: w1273 -> [w1277 w1280]
                                tunnel: [w1276 w1279] -> w1267
                                tunnel: w1272 -> [w1276 w1282]
                                tunnel: [w1275 w1280] -> w1266
                                tunnel: w1270 -> [w1275 w1281]
                                tunnel: w1265 -> [_ _]
                                frame False {
                                }
                                frame True {
                                }
                                }
                                }
                                }
                                n497 = expression code="x/2"(w1251) -> (w1249:sgl)
                                n498 = Negate(x=w1249) -> (-x=w1250:sgl)
                              }
                            }
                            n499 = Concatenate Strings("axial depth " ("string"), w1233) -> (w1231:string)
                            n500 = Concatenate Strings("lateral width " ("string"), w1232) -> (w1230:string)
                            n501 = property on="Real Time Image" class="IntGraph (strict)"("YScale.NameLbl.Text"=w1231, "XScale.NameLbl.Text"=w1230, "X Scale.Offset and Multiplier:Offset"=w1228, "XScale.Minimum"=w1223, "XScale.Maximum"=w1225, "X Scale.Offset and Multiplier:Multiplier"=w1242, "Y Scale.Offset and Multiplier:Offset"=w1241, "Y Scale.Offset and Multiplier:Multiplier"=w1240, "Transpose Array"=w1239) -> ()  [unwired: 2 in, 2 out]
                          }
                          frame #1 {
                            n502 = case shown="\"Hawaii\", \"Stony Brook\"" w1283 {
                              tunnel: w1288 -> [_ w1313]
                              tunnel: w1287 -> [_ w1312]
                              tunnel: w1286 -> [_ w1311]
                              tunnel: w1285 -> [_ w1302]
                              tunnel: w1284 -> [_ w1310]
                              frame "WCM Main", Default {
                              }
                              frame "Hawaii", "Stony Brook" {
                                n503 = Unbundle By Name(w1312) -> ("lines per plane"=w1308:i32, "Digitizer delay (us)"=w1321:dbl, "Samp Rate (Hz)"=w1317:dbl, "rf points per line"=w1319:i32)
                                n504 = Unbundle By Name(w1310) -> ("Distance between\nscan lines (um)"=w1309:sgl)
                                n505 = Unbundle By Name(w1313) -> ("Scan Size"=w1328:dbl[], "XDCR Settings"=w1314:T2[])
                                n506 = Index Array(array=w1314, index=w1311) -> (element=w1322:T2)
                                n507 = expression code="x*1e-6"(w1317) -> (w1318:dbl)
                                n508 = expression code="x/2"(w1302) -> (w1305:sgl)
                                n509 = Unbundle By Name(w1322) -> ("XDCR Focal Length"=w1303:dbl, "Data Vertical Center"=w1296:dbl)
                                n510 = expression code="x*1e-3"(w1309) -> (w1307:sgl)
                                n511 = Divide(x=w1305, y=w1318) -> (x/y=w1320:dbl)
                                n512 = Multiply(x=w1305, y=w1321) -> (x*y=w1294:dbl)
                                n513 = Multiply(x=w1320, y=w1319) -> (x*y=w1304:dbl)
                                n514 = Multiply(x=w1307, y=w1308) -> (x*y=w1306:sgl)
                                n515 = Add(x=w1294, y=w1304) -> (x+y=w1289:dbl)
                                n516 = Index Array(array=w1328, index #1=0 ("index")) -> (element #1=w1324:dbl, element #3=w1295:dbl)  [unwired: 2 in, 1 out]
                                n517 = expression code="x/2"(w1324) -> (w1315:dbl)
                                n518 = Divide(x=w1306, y=2) -> (x/y=w1330:sgl)
                                n519 = call "Decimal Rounding.vi"("Round Method (Nearest)"=T47."Round to -INF", "Input"=w1294) -> ("Output"=w1293:dbl)  [unwired: 9 in]
                                n520 = expression code="x/2"(w1295) -> (w1297:dbl)
                                n521 = call "Decimal Rounding.vi"("Round Method (Nearest)"=T47."Round to +INF", "Input"=w1289) -> ("Output"=w1290:dbl)  [unwired: 9 in]
                                n522 = Negate(x=w1315) -> (-x=w1316:dbl)
                                n523 = Negate(x=w1330) -> (-x=w1329:sgl)
                                n524 = Subtract(x=w1296, y=w1297) -> (x-y=w1299:dbl)
                                n525 = Add(x=w1297, y=w1296) -> (x+y=w1298:dbl)
                                n526 = property on="Real Time Image" class="IntGraph (strict)"("XScale.Minimum"=w1329, "XScale.Maximum"=w1330, "Active Cursor"=u32 0, "Cursor.Cursor X"=w1316, "Active Cursor"=u32 1, "Cursor.Cursor X"=w1315, "Active Cursor"=u32 2, "Cursor.Cursor Y"=w1303, "YScale.Minimum"=w1293, "YScale.Maximum"=w1290, "Active Cursor"=u32 3, "Cursor.Cursor Y"=w1299, "Active Cursor"=u32 4, "Cursor.Cursor Y"=w1298) -> ()  [unwired: 2 in, 2 out]
                              }
                            }
                          }
                        }
                      }
                      event "1-to-1": Value Change {
                        n527 = event-data() -> ()  [unwired: 1 in, 6 out]
                        n528 = property on="Real Time Image" class="IntGraph (strict)"() -> ("X Scale.Offset and Multiplier:Multiplier"=w1352:dbl, "Y Scale.Offset and Multiplier:Multiplier"=w1351:dbl, "Plot Bounds"=w1337:T41, "Plot Area Size"=w1336:T67)  [unwired: 2 in, 2 out]
                        n529 = Unbundle By Name(w1338) -> ("lines per plane"=w1340:i32, "rf points per line"=w1339:i32)
                        n530 = Multiply(x=w1340, y=w1352) -> (x*y=w1350:dbl)
                        n531 = Multiply(x=w1351, y=w1339) -> (x*y=w1349:dbl)
                        n532 = Unbundle(w1336) -> ("Width"=w1344:u32, "Height"=w1342:u32)
                        n533 = Divide(x=w1344, y=w1350) -> (x/y=w1348:dbl)
                        n534 = Divide(x=w1342, y=w1349) -> (x/y=w1347:dbl)
                        n535 = Divide(x=w1348, y=w1347) -> (x/y=w1343:dbl)
                        n536 = Greater?(x=w1343, y=1.0) -> (0:w1346:bool)
                        n537 = case shown="True" w1346 {
                          tunnel: w1344 -> [_ w1368]
                          tunnel: w1343 -> [w1361 w1367]
                          tunnel: w1342 -> [w1360 _]
                          tunnel: w1337 -> [w1355 w1366]
                          tunnel: [w1356 w1362] -> w1341
                          frame False {
                            n538 = Unbundle By Name(w1355) -> ("Top"=w1359:i16)
                            n539 = Multiply(x=w1360, y=w1361) -> (x*y=w1357:dbl)
                            n540 = Add(x=w1359, y=w1357) -> (x+y=w1358:dbl)
                            n541 = Bundle By Name(cluster=w1355, "Bottom"=w1358) -> (w1356:T41)
                          }
                          frame True {
                            n542 = Unbundle By Name(w1366) -> ("Left"=w1364:i16)
                            n543 = Divide(x=w1368, y=w1367) -> (x/y=w1365:dbl)
                            n544 = Add(x=w1364, y=w1365) -> (x+y=w1363:dbl)
                            n545 = Bundle By Name(cluster=w1366, "Right"=w1363) -> (w1362:T41)
                          }
                        }
                        n546 = property on="Real Time Image" class="IntGraph (strict)"("Plot Bounds"=w1341) -> ()  [unwired: 2 in, 2 out]
                      }
                      event "Fill": Value Change {
                        n547 = event-data() -> ()  [unwired: 1 in, 6 out]
                        n548 = property on="Real Time Image" class="IntGraph (strict)"("Plot Bounds"=w1373) -> ()  [unwired: 2 in, 2 out]
                      }
                      event "Position (mm)": Value Change {
                        n549 = event-data() -> ("NewVal"=w1387:dbl)  [unwired: 1 in]
                        n550 = Unbundle By Name(w1382) -> ("Motion System"=w1386:T27)
                        n551 = case shown="\"NI 735x\", Default" w1386 {
                          tunnel: w1387 -> [_ w1392]
                          tunnel: w1382 -> [w1388 w1390]
                          tunnel: [w1388 w1391] -> w1385
                          tunnel: w1378 -> [_ w1389]
                          frame "MM3000", "Newport ESP", "No Motion Card" {
                          }
                          frame "NI 735x", Default {
                            n552 = disable-structure shown="Disabled" {
                              disable-tunnel: w1392 -> [w1401 _]
                              disable-tunnel: [w1396 _] -> w1391
                              disable-tunnel: w1390 -> [w1395 _]
                              disable-tunnel: w1389 -> [w1393 _]
                              frame Disabled {
                                n553 = Unbundle By Name(w1395) -> ("Steps per mm"=w1398:i32[], "Motion Bd ID"=w1397:u8)
                                n554 = local read "Axis Tune"() -> (w1399:enum32{"Axis 1", "Axis 2", "Axis 3", "Axis 4"})
                                n555 = Decrement(x=w1393) -> (x-1=w1394:i32)
                                n556 = Index Array(array=w1398, index=w1399) -> (element=w1406:i32)
                                n557 = Equal?(x=w1399, y=w1394) -> (x = y?=w1402:bool)
                                n558 = To Byte Integer(number=w1399) -> (8bit integer=w1403:i8)
                                n559 = Multiply(x=w1401, y=w1406) -> (x*y=w1405:dbl)
                                n560 = Increment(x=w1403) -> (x+1=w1400:i8)
                                n561 = case shown="\"Axis 3\"" w1399 {
                                tunnel: w1405 -> [w1422 w1426]
                                tunnel: [w1422 w1425] -> w1404
                                tunnel: w1395 -> [_ w1424]
                                frame "Axis 1", Default {
                                }
                                frame "Axis 3" {
                                n562 = Unbundle By Name(w1424) -> ("Reverse Z axis?"=w1423:bool)
                                n563 = Negate(x=w1426) -> (-x=w1427:dbl)
                                n564 = Select(t=w1427, s=w1423, f=w1426) -> (s? t:f=w1425:dbl)
                                }
                                }
                                n565 = case shown="False" w1402 {
                                tunnel: w1400 -> [w1416 _]
                                tunnel: w1404 -> [w1409 _]
                                tunnel: w1397 -> [w1408 _]
                                tunnel: w1399 -> [_ w1421]
                                tunnel: w1395 -> [w1407 w1419]
                                tunnel: [w1407 w1417] -> w1396
                                frame False {
                                n566 = call <vilib>:"Set Operation Mode.flx"("Axis or Vector Space"=w1416, "Board ID"=w1408) -> ("error out"=w1415:errorcluster, "Resource Output"=w1413:T56, "Bd ID Out"=w1414:T54)  [unwired: 4 in]
                                n567 = call <vilib>:"Load Target Position.flx"("Target Position (0)"=w1409, "error in (no error)"=w1415, "Axis"=w1413, "Board ID"=w1414) -> ("error out"=w1411:errorcluster, "Resource Output"=w1410:T56, "Bd ID Out"=w1412:T54)  [unwired: 3 in]
                                n568 = call-poly <vilib>:"Start Motion.flx"("error in (no error)"=w1411, "Axis or Vector Space"=w1410, "Board ID"=w1412) -> ()  [unwired: 3 in, 3 out]
                                }
                                frame True {
                                n569 = call "FindLocation_SingleAxis.vi"("Axis (0 is X)"=w1421, "Motion Settings"=w1419) -> ("Global Position"=w1418:dbl[], "Position (mm) (Abs)"=w1420:dbl)  [unwired: 2 in, 2 out]
                                n570 = Bundle By Name(cluster=w1419, "Global Position (mm)"=w1418) -> (w1417:T26)
                                n571 = local write "Position (mm)"(w1420) -> ()
                                }
                                }
                              }
                              frame Enabled {
                              }
                            }
                          }
                        }
                      }
                      event Key Down {
                        n572 = event-data() -> ("VKey"=w1440:T68, "PlatMods"=w1458:T69, "Char"=w1437:i16)  [unwired: 1 in]
                        n573 = property on="Dig Scale" class="Ring (strict)"() -> ("Key Focus"=w1455:bool)  [unwired: 2 in, 2 out]
                        n574 = property on="lines per plane" class="DigNum (strict)"() -> ("Key Focus"=w1454:bool)  [unwired: 2 in, 2 out]
                        n575 = property on="Sampling Rate" class="Ring (strict)"() -> ("Key Focus"=w1453:bool)  [unwired: 2 in, 2 out]
                        n576 = property on="Distance between\nscan lines (um)" class="DigNum (strict)"() -> ("Key Focus"=w1452:bool)  [unwired: 2 in, 2 out]
                        n577 = property on="Ref Delay (ms)" class="DigNum (strict)"() -> ("Key Focus"=w1451:bool)  [unwired: 2 in, 2 out]
                        n578 = property on="Frames/s" class="DigNum (strict)"() -> ("Key Focus"=w1450:bool)  [unwired: 2 in, 2 out]
                        n579 = property on="rf points per line" class="DigNum (strict)"() -> ("Key Focus"=w1449:bool)  [unwired: 2 in, 2 out]
                        n580 = property on="BKPT Shift" class="DigNum (strict)"() -> ("Key Focus"=w1448:bool)  [unwired: 2 in, 2 out]
                        n581 = case shown="2" w1439 {
                          tunnel: w1440 -> [_ w1469 w1472 w1475 _]
                          tunnel: [_ w1468 w1471 w1474 w1478] -> w1438
                          tunnel: w1437 -> [_ _ _ _ w1477]
                          frame 0, Default {
                          }
                          frame 1 {
                            n582 = case shown="\"Left\", \"Right\"" w1469 {
                              tunnel: [_ TRUE ("No data")] -> w1468
                              frame "ASCII", Default {
                              }
                              frame "Left", "Right" {
                              }
                            }
                          }
                          frame 2 {
                            n583 = case shown="\"Up\", \"Down\"" w1472 {
                              tunnel: [_ TRUE ("No data")] -> w1471
                              frame "ASCII", Default {
                              }
                              frame "Up", "Down" {
                              }
                            }
                          }
                          frame 3 {
                            n584 = case shown="\"PageUp\", \"PageDown\"" w1475 {
                              tunnel: [_ TRUE ("No data")] -> w1474
                              frame "ASCII", Default {
                              }
                              frame "PageUp", "PageDown" {
                              }
                            }
                          }
                          frame 4 {
                            n585 = case shown="0, Default" w1477 {
                              tunnel: [_ TRUE ("No data")] -> w1478
                              frame 0, Default {
                              }
                              frame 67, 90, 99, 122 {
                              }
                            }
                          }
                        }
                        n586 = Compound Arithmetic op=OR(w1455, w1454, w1453, w1452, w1451, w1450, w1449, w1448) -> (w1443:bool)
                        n587 = property on="UT340 Controls" class="Clust (strict)"() -> ("Key Focus"=w1429:bool)  [unwired: 2 in, 2 out]
                        n588 = property on="Inc Step Size\n(mm)" class="DigNum (strict)"() -> ("Key Focus"=w1433:bool)  [unwired: 2 in, 2 out]
                        n589 = property on="Position (mm)" class="DigNum (strict)"() -> ("Key Focus"=w1447:bool)  [unwired: 2 in, 2 out]
                        n590 = property on="File Name" class="Str"() -> ("Key Focus"=w1446:bool)  [unwired: 2 in, 2 out]
                        n591 = property on="Overshoot" class="DigNum (strict)"() -> ("Key Focus"=w1445:bool)  [unwired: 2 in, 2 out]
                        n592 = property on="Filter Prams" class="Clust (strict)"() -> ("Key Focus"=w1444:bool)  [unwired: 2 in, 2 out]
                        n593 = property on="Transducer" class="Ring (strict)"() -> ("Key Focus"=w1434:bool)  [unwired: 2 in, 2 out]
                        n594 = property on="Acquisition Volume (mm)" class="Arr (strict)"() -> ("Key Focus"=w1435:bool)  [unwired: 2 in, 2 out]
                        n595 = Compound Arithmetic op=OR(w1438, w1443, w1447, w1446, w1445, w1444, w1435, w1434, w1433, w1429) -> (w1442:bool)
                        n596 = control-ref of="Position (mm)"() -> (w1459:refnum<vi>)
                        n597 = control-ref of="Axis Tune"() -> (w1460:refnum<vi>)
                        n598 = control-ref of="UT340 Controls"() -> (w1428:refnum<vi>)
                        n599 = control-ref of="JSR Simple"() -> (w1431:refnum<vi>)
                        n600 = control-ref of="Daxsonics Settings"() -> (w1432:refnum<vi>)
                        n601 = call "KeyboardNudge.vi"("Axis Tune Refnum"=w1460, "Char"=w1437, "Position (mm) Refnum"=w1459, "Ignore Key Down"=w1442, "VKey"=w1440, "PlatMods"=w1458, "Daxsonics Settings"=w1432, "Pulser"=w1430, "Inc. Step Size (mm)"="Inc Step Size\n(mm)", "Motion Settings"=w1457, "UT340 Controls"=w1428, "JSR Simple"=w1431) -> ("Z Move?"=w1436:bool, "Quit"=w1441:bool)  [unwired: 6 in]
                        n602 = case shown="False" w1442 {
                          tunnel: w1461 -> [w1483 _]
                          tunnel: w1437 -> [w1482 _]
                          tunnel: w1440 -> [w1481 _]
                          tunnel: w1441 -> [_ _]
                          tunnel: w1436 -> [w1480 _]
                          frame False {
                            n603 = case shown="\"M scan\", Default" w1483 {
                              tunnel: w1481 -> [w1486 _]
                              tunnel: w1482 -> [w1485 _]
                              tunnel: w1480 -> [w1484 _]
                              frame "Dual Transducer" {
                                n604 = case shown="\"Up\", \"Down\"" w1486 {
                                tunnel: w1485 -> [w1491 _ _]
                                frame "ASCII", Default {
                                n605 = case shown="32" w1491 {
                                frame 0, Default {
                                }
                                frame 32 {
                                n606 = property on="Center" class="Bool (strict)"("Val(Sgnl)"=TRUE ("Value (Signaling)")) -> ()  [unwired: 2 in, 2 out]
                                }
                                }
                                }
                                frame "Return" {
                                n607 = property on="End Point\nMarker" class="Bool (strict)"("Val(Sgnl)"=TRUE ("Value (Signaling)")) -> ()  [unwired: 2 in, 2 out]
                                }
                                frame "Up", "Down" {
                                }
                                }
                                n608 = case shown="True" w1484 {
                                frame False {
                                }
                                frame True {
                                w1488 = 2 ("index")
                                n609 = property on="Scan Start Pos (mm)" class="Arr (strict)"() -> ("Value"=w1490:dbl[])  [unwired: 2 in, 2 out]
                                n610 = call "FindLocation_SingleAxis.vi"("Axis (0 is X)"=w1488) -> ()  [unwired: 3 in, 4 out]
                                n611 = property on="Position (mm)" class="DigNum (strict)"() -> ("Value"=w1487:dbl)  [unwired: 2 in, 2 out]
                                n612 = Replace Array Subset(array=w1490, new element=w1487, index=w1488) -> (w1489:dbl[])
                                n613 = property on="Scan Start Pos (mm)" class="Arr (strict)"("Value"=w1489) -> ()  [unwired: 2 in, 2 out]
                                }
                                }
                              }
                              frame "M scan", Default {
                              }
                            }
                          }
                          frame True {
                          }
                        }
                      }
                      event "Real Time Image": Cursor Release; "Initilize": Value Change {
                        n614 = event-data() -> ()  [unwired: 1 in, 1 out]
                        n615 = control-ref of="Real Time Image"() -> (w1494:refnum<vi>)
                        n616 = case shown="\"Hawaii\"" w1501 {
                          tunnel: [FALSE TRUE] -> w1500
                          frame "Hawaii" {
                          }
                          frame "Stony Brook", Default {
                          }
                        }
                        n617 = property on="Force Symmetric?" class="Bool (strict)"() -> ("Value"=w1499:bool)  [unwired: 2 in, 2 out]
                        n618 = call "DualTransCursorFix.vi"("IntensityGraph in"=w1494, "Digitizer Settings in"=w1512, "Force Include Focus?"=w1500, "Force Symmetric?"=w1499, "Motion Settings"=w1511, "Cursor\nHold-off"=w1502, "Current Trans"=w1508, "Scan Size in"=w1510, "Dual XDCR Settings"=w1509) -> ("Digitizer Settings out"=w1495:T30, "Scan Center (mm)"=w1498:dbl, "lines per plane"=w1504:i32, "rf points per line"=w1503:i32, "Dual XDCR Settings out"=w1505:T1, "Scan Size out"=w1496:dbl[], "Ref Delay (ms)"=w1506:dbl)
                        n619 = property on="lines per plane" class="DigNum (strict)"("Value"=w1504) -> ()  [unwired: 2 in, 2 out]
                        n620 = property on="rf points per line" class="DigNum (strict)"("Value"=w1503) -> ()  [unwired: 2 in, 2 out]
                        n621 = property on="Ref Delay (ms)" class="DigNum (strict)"("Value"=w1506) -> ()  [unwired: 2 in, 2 out]
                        n622 = case shown="False" w1499 {
                          tunnel: w1498 -> [w1517 _]
                          tunnel: w1497 -> [w1516 _]
                          frame False {
                            n623 = Negate(x=w1517) -> (-x=w1514:dbl)
                            n624 = property on="Scan Start Pos (mm)" class="Arr (strict)"() -> ("Value"=w1519:dbl[])  [unwired: 2 in, 2 out]
                            n625 = Decrement(x=w1516) -> (x-1=w1515:i32)
                            n626 = in-place {
                              in-place-border: w1514 -> [w1520]
                              n627 = in-place-array #2(w1519, w1515) -> (w1522:dbl)
                              n628 = Subtract(x=w1522, y=w1520) -> (x-y=w1521:dbl)
                              n629 = in-place-array #2(w1521) -> (w1518:dbl[])  [unwired: 1 out]
                            }
                            n630 = property on="Scan Start Pos (mm)" class="Arr (strict)"("Value"=w1518) -> ()  [unwired: 2 in, 2 out]
                          }
                          frame True {
                          }
                        }
                        n631 = property on="Acquisition Volume (mm)" class="Arr (strict)"("Value"=w1496) -> ()  [unwired: 2 in, 2 out]
                      }
                      event "Axis Tune": Value Change {
                        n632 = event-data() -> ("NewVal"=w1534:enum32{"Axis 1", "Axis 2", "Axis 3", "Axis 4"})  [unwired: 1 in]
                        n633 = Unbundle By Name(w1532) -> ("Motion System"=w1531:T27)
                        n634 = case shown="\"MM3000\", \"Newport ESP\", \"No Motion Card\"" w1531 {
                          tunnel: w1534 -> [w1539 _]
                          tunnel: w1532 -> [w1537 w1540]
                          tunnel: [w1535 w1540] -> w1530
                          frame "NI 735x", Default {
                            n635 = call "FindLocation_SingleAxis.vi"("Axis (0 is X)"=w1539, "Motion Settings"=w1537) -> ("Global Position"=w1536:dbl[], "Position (mm) (Abs)"=w1538:dbl)  [unwired: 2 in, 2 out]
                            n636 = local write "Position (mm)"(w1538) -> ()
                            n637 = Bundle By Name(cluster=w1537, "Global Position (mm)"=w1536) -> (w1535:T26)
                          }
                          frame "MM3000", "Newport ESP", "No Motion Card" {
                          }
                        }
                      }
                      event "Stop Motor": Value Change {
                        n638 = event-data() -> ()  [unwired: 1 in, 1 out]
                        n639 = local read "Axis Tune"() -> (w1554:enum32{"Axis 1", "Axis 2", "Axis 3", "Axis 4"})
                        n640 = Unbundle By Name(w1542) -> ("Motion System"=w1541:T27)
                        n641 = case shown="\"NI 735x\"" w1541 {
                          tunnel: w1554 -> [_ w1557 _]
                          tunnel: [_ w1556 w1564] -> w1552
                          tunnel: w1542 -> [_ w1555 w1567]
                          frame "MM3000", Default {
                          }
                          frame "NI 735x" {
                            n642 = disable-structure shown="Disabled" {
                              disable-tunnel: w1557 -> [w1561 _]
                              disable-tunnel: [w1560 _] -> w1556
                              disable-tunnel: w1555 -> [w1558 _]
                              frame Disabled {
                                n643 = Unbundle By Name(w1558) -> ("Motion Bd ID"=w1559:u8)
                                n644 = Increment(x=w1561) -> (x+1=w1563:enum32{"Axis 1", "Axis 2", "Axis 3", "Axis 4"})
                                n645 = call-poly <vilib>:"Stop Motion.flx"("Stop Type (Decel)"=enum16{"Decelerate", "Halt", "Kill"}."Halt", "Axis or Vector Space"=w1563, "Board ID"=w1559) -> ("error out"=w1560:errorcluster)  [unwired: 4 in, 2 out]
                              }
                              frame Enabled {
                              }
                            }
                          }
                          frame "Galil" {
                            n646 = Unbundle By Name(w1567) -> ("GL Ref Out"=w1565:refnum<k7>)
                            n647 = call "GL Command Set.vi"("Command"=Command_Menu."Abort Motion", "Galil.IGalil"=w1565) -> ("error out"=w1564:errorcluster)  [unwired: 5 in, 4 out]
                          }
                        }
                        n648 = call "FindLocation_SingleAxis.vi"("error in (no error)"=w1552, "Axis (0 is X)"=w1554, "Motion Settings"=w1542) -> ("error out"=w1543:errorcluster, "Global Position"=w1550:dbl[], "Position (mm) (Abs)"=w1553:dbl)  [unwired: 1 in, 1 out]
                        n649 = Bundle By Name(cluster=w1542, "Global Position (mm)"=w1550) -> (w1549:T26)
                        n650 = local write "Position (mm)"(w1553) -> ()
                        n651 = property on="error out" class="Clust (strict)"("Value"=w1543) -> ()  [unwired: 2 in, 2 out]
                      }
                      event "Acquistion Parameters": Value Change {
                        # "Restart loops with new digitizer settings"
                        n652 = event-data() -> ("NewVal"=w1593:T36, "OldVal"=w1583:T36)  [unwired: 1 in]
                        n653 = Unbundle By Name(w1593) -> ("Sampling Rate"=w1584:dbl, "Ref Delay (ms)"=w1581:dbl, "rf points per line"=w1578:i32, "Dig Scale"=w1585:dbl)
                        n654 = Unbundle By Name(w1583) -> ("Ref Delay (ms)"=w1580:dbl, "rf points per line"=w1579:i32)
                        n655 = expression code="x*1E6"(w1584) -> (w1582:dbl)
                        n656 = Subtract(x=w1581, y=w1580) -> (x-y=w1576:dbl)
                        n657 = Subtract(x=w1578, y=w1579) -> (x-y=w1577:i32)
                        n658 = case shown="\"Dual Transducer\"" w1573 {
                          tunnel: w1589 -> [w1598 w1603]
                          tunnel: [w1597 w1612] -> w1569
                          tunnel: w1588 -> [w1594 w1605]
                          tunnel: w1587 -> [_ w1608]
                          tunnel: w1586 -> [_ w1619]
                          tunnel: [w1595 w1618] -> w1572
                          tunnel: w1582 -> [w1602 w1604]
                          tunnel: w1581 -> [w1601 _]
                          tunnel: w1578 -> [w1600 _]
                          tunnel: w1585 -> [w1599 w1617]
                          tunnel: w1577 -> [_ _]
                          tunnel: w1576 -> [_ _]
                          tunnel: w1575 -> [w1595 w1606]
                          tunnel: [TRUE TRUE] -> w1568
                          tunnel: [w1594 w1605] -> w1571
                          tunnel: w1570 -> [_ _]
                          frame "M scan", Default {
                            n659 = Bundle By Name(cluster=w1598, "Samp Rate (Hz)"=w1602, "Digitizer delay (us)"=w1601, "rf points per line"=w1600, "Voltage Scale"=w1599) -> (w1597:T30)
                          }
                          frame "Dual Transducer" {
                            n660 = Unbundle By Name(w1606) -> ("XDCR Settings"=w1610:T2[])
                            n661 = property on="Dual XDCR\nDigi Time Settings" class="Arr (strict)"() -> ("Value"=w1611:cluster{"RF PPL":i32, "Ref Delay (us)":dbl}[])  [unwired: 2 in, 2 out]
                            n662 = To Long Integer(number=w1608) -> (32bit integer=w1607:i32)
                            n663 = in-place {
                              in-place-border: w1604 -> [w1628]
                              n664 = in-place-array #3(w1610, w1607) -> (w1627:T2)
                              n665 = in-place-array #4(w1611, w1607) -> (w1629:cluster{"RF PPL":i32, "Ref Delay (us)":dbl})
                              n666 = Unbundle By Name(w1627) -> ("Digitizer Settings.RF data Sampling.Sampling Rate"=w1626:dbl)
                              n667 = expression code="x*1e-6"(w1628) -> (w1625:dbl)
                              n668 = Unbundle By Name(w1629) -> ("RF PPL"=w1624:i32)
                              n669 = Divide(x=w1626, y=w1625) -> (x/y=w1623:dbl)
                              n670 = Divide(x=w1624, y=w1623) -> (x/y=w1622:dbl)
                              n671 = To Long Integer(number=w1622) -> (32bit integer=w1621:i32)
                              n672 = Bundle By Name(cluster=w1629, "RF PPL"=w1621) -> (w1630:cluster{"RF PPL":i32, "Ref Delay (us)":dbl})
                              n673 = property on="rf points per line" class="DigNum (strict)"("Value"=w1621) -> ()  [unwired: 2 in, 2 out]
                              n674 = in-place-array #3(w1627) -> ()  [unwired: 2 out]
                              n675 = in-place-array #4(w1630) -> (w1609:cluster{"RF PPL":i32, "Ref Delay (us)":dbl}[])  [unwired: 1 out]
                            }
                            n676 = Index Array(array=w1609, index=w1607) -> (element=w1616:cluster{"RF PPL":i32, "Ref Delay (us)":dbl})
                            n677 = Unbundle By Name(w1616) -> ("Ref Delay (us)"=w1615:dbl, "RF PPL"=w1614:i32)
                            n678 = property on="Dual XDCR\nDigi Time Settings" class="Arr (strict)"("Value"=w1609) -> ()  [unwired: 2 in, 2 out]
                            n679 = Bundle By Name(cluster=w1603, "Samp Rate (Hz)"=w1604, "Voltage Scale"=w1617, "Digitizer delay (us)"=w1615, "rf points per line"=w1614) -> (w1612:T30)
                            n680 = Increment(x=w1607) -> (x+1=w1620:i32)
                            n681 = call "UpdateDualXDCRSettings.vi"("Digitizer Settings in"=w1612, "Motion Settings in"=w1605, "Switch T/R"=w1620, "Dual XDCR Settings In"=w1606, "Switch Unit"=w1619) -> ("Dual XDCR Settings"=w1618:T1)  [unwired: 3 in]
                          }
                        }
                        n682 = Send Notification(notification=w1568, notifier=w1592) -> ()  [unwired: 1 in, 2 out]
                      }
                      event "Motion Parameters": Value Change {
                        w1655 = TRUE
                        # "Update parameters related to motion"
                        n683 = event-data() -> ("NewVal"=w1653:T37)  [unwired: 1 in]
                        n684 = Unbundle By Name(w1653) -> ("lines per plane"=w1634:u16, "Overshoot"=w1635:i32, "BKPT Shift"=w1652:i32, "Frames/s"=w1651:sgl, "Distance between\nscan lines (um)"=w1646:sgl)
                        n685 = Unbundle By Name(w1649) -> ("Steps per mm"=w1648:i32[])
                        n686 = Decrement(x=w1636) -> (x-1=w1650:i32)
                        n687 = Index Array(array=w1648, index=w1650) -> (element=w1645:i32)
                        n688 = Decrement(x=w1634) -> (x-1=w1647:u16)
                        n689 = Compound Arithmetic op=MULTIPLY(w1647, w1646, w1645, 0.001) -> (w1643:dbl)
                        n690 = Bundle By Name(cluster=w1649, "overshoot cts"=w1635, "BKPT Shift"=w1652, "RT fps"=w1651, "Distance between\nscan lines (um)"=w1646, "Total steps in line"=w1643) -> (w1640:T26)
                        n691 = Bundle By Name(cluster=w1654, "lines per plane"=w1634) -> (w1631:T30)
                        n692 = Send Notification(notification=w1655, notifier=w1656) -> ()  [unwired: 1 in, 2 out]
                        n693 = case shown="\"Dual Transducer\"" w1632 {
                          tunnel: w1631 -> [_ w1666]
                          tunnel: w1641 -> [_ w1660]
                          tunnel: w1640 -> [_ w1665]
                          tunnel: w1639 -> [w1658 w1664]
                          tunnel: [w1658 w1663] -> w1638
                          tunnel: w1637 -> [_ w1662]
                          frame "M scan", Default {
                          }
                          frame "Dual Transducer" {
                            n694 = To Long Integer(number=w1660) -> (32bit integer=w1659:i32)
                            n695 = Increment(x=w1659) -> (x+1=w1661:i32)
                            n696 = call "UpdateDualXDCRSettings.vi"("Digitizer Settings in"=w1666, "Motion Settings in"=w1665, "Switch T/R"=w1661, "Dual XDCR Settings In"=w1664, "Switch Unit"=w1662) -> ("Dual XDCR Settings"=w1663:T1)  [unwired: 3 in]
                          }
                        }
                      }
                      event "Full Scan Size (mm)", "Reset Scan": Value Change {
                        w1670 = TRUE
                        n697 = event-data() -> ()  [unwired: 1 in, 6 out]
                        n698 = property on="Reset Scan" class="Bool (strict)"("Value"=FALSE ("Reset Scan")) -> ()  [unwired: 2 in, 2 out]
                        n699 = Send Notification(notification=w1670, notifier=w1669) -> ()  [unwired: 1 in, 2 out]
                        "Z Change" <- TRUE ("Z Change")
                      }
                      event "Distance Between Planes (um)": Value Change {
                        n700 = event-data() -> ()  [unwired: 1 in, 1 out]
                        n701 = Unbundle By Name(w1684) -> ("Distance between\nscan planes (um)"=w1683:sgl, "number of scan planes"=w1680:i32)
                        n702 = Unbundle By Name(w1692) -> ("XDCR Settings"=w1691:T2[])
                        n703 = for {
                          tunnel: w1691 -> [w1698] mode=indexing
                          tunnel: [w1697] -> w1690 mode=indexing
                          tunnel: "Distance Between Planes (um)" -> [w1696] mode=indexing
                          n704 = Bundle By Name(cluster=w1698, "Motion Settings.Distance between\nscan planes (um)"=w1696) -> (w1697:T2)
                        }
                        n705 = Index Array(array="Distance Between Planes (um)", index=w1685) -> (element=w1682:sgl)
                        n706 = Divide(x=w1683, y=w1682) -> (x/y=w1681:sgl)
                        n707 = Multiply(x=w1681, y=w1680) -> (x*y=w1679:sgl)
                        n708 = call "Force Odd or Even.vi"("input"=w1679) -> ("output"=w1678:i32)  [unwired: 1 in]
                        n709 = Bundle By Name(cluster=w1684, "Distance between\nscan planes (um)"=w1682, "number of scan planes"=w1678) -> (w1687:T26)
                        n710 = Bundle By Name(cluster=w1692, "XDCR Settings"=w1690) -> (w1688:T1)
                      }
                      event "SetDig": Value Change {
                        w1699 = TRUE
                        # "Update digitizer settings"
                        n711 = event-data() -> ()  [unwired: 1 in, 1 out]
                        n712 = case shown="\"Dual Transducer\"" w1700 {
                          tunnel: w1714 -> [w1724 w1729]
                          tunnel: [w1722 w1732] -> w1713
                          tunnel: w1712 -> [w1721 w1755]
                          tunnel: [w1723 w1754] -> w1711
                          tunnel: w1709 -> [w1717 w1750]
                          tunnel: [w1717 w1749] -> w1708
                          tunnel: w1706 -> [w1720 w1747]
                          tunnel: w1705 -> [_ w1745]
                          tunnel: w1703 -> [_ w1744]
                          tunnel: w1702 -> [w1719 w1743]
                          tunnel: [w1718 w1742] -> w1701
                          frame "Therapy With Scan", Default {
                            n713 = call "SetUpDigi.vi"("Digitizer Settings"=w1724, "Motion Settings In"=w1721, "Ann Array Params"=w1720, "Dual XDCR Settings"=w1719) -> ("Dual XDCR Settings Out"=w1718:T1, "Digitizer Settings Out"=w1722:T30, "Motion Settings Out"=w1723:T26)  [unwired: 9 in, 4 out]
                          }
                          frame "Dual Transducer" {
                            n714 = property on="Dual XDCR\nDigi Time Settings" class="Arr (strict)"() -> ("Value"=w1736:cluster{"RF PPL":i32, "Ref Delay (us)":dbl}[])  [unwired: 2 in, 2 out]
                            n715 = case shown="False" w1744 {
                              tunnel: w1755 -> [w1767 w1768]
                              tunnel: [w1766 w1768] -> w1753
                              frame False {
                                n716 = property on="Scan Start Pos (mm)" class="Arr (strict)"() -> ("Value"=w1763:dbl[])  [unwired: 2 in, 2 out]
                                n717 = call "MultiAxisMove.vi"("Find Location"=TRUE, "Wait For Move Complete"=TRUE, "Position Mode (Rel)"=T48."Absolute Position", "Distance to move (mm)"=w1763, "Motion Settings"=w1767) -> ("Motion Settings Out"=w1766:T26)  [unwired: 4 in, 2 out]
                              }
                              frame True {
                              }
                            }
                            n718 = To Unsigned Long Integer(number=w1750) -> (unsigned 32bit integer=w1735:u32)
                            n719 = Increment(x=w1735) -> (x+1=w1741:u32)
                            n720 = Index Array(array=w1736, index=w1735) -> (element=w1734:cluster{"RF PPL":i32, "Ref Delay (us)":dbl})
                            n721 = Bundle By Name(cluster=w1747, "Switch T/R"=w1741) -> (w1746:T22)
                            n722 = property on="Ref Delay (ms)" class="DigNum (strict)"() -> ("Value"=w1726:dbl)  [unwired: 2 in, 2 out]
                            n723 = Unbundle By Name(w1734) -> ("Ref Delay (us)"=w1728:dbl, "RF PPL"=w1730:i32)
                            n724 = Subtract(x=w1726, y=w1728) -> (x-y=w1727:dbl)
                            n725 = Bundle By Name(cluster=w1729, "Additional dig delay (us)"=w1727, "Digitizer delay (us)"=w1728, "rf points per line"=w1730) -> (w1733:T30)
                            n726 = call "SetUpDigi.vi"("Digitizer Settings"=w1733, "Motion Settings In"=w1753, "Ann Array Params"=w1746, "Dual XDCR Settings"=w1743) -> ("Dual XDCR Settings Out"=w1742:T1, "Digitizer Settings Out"=w1752:T30, "Motion Settings Out"=w1740:T26, "Ann Array Params out"=w1739:T22)  [unwired: 9 in, 3 out]
                            n727 = case shown="True" w1744 {
                              tunnel: w1740 -> [w1756 w1761]
                              tunnel: [w1756 w1760] -> w1751
                              frame False {
                              }
                              frame True {
                                w1757 = 0.0 ("new element/subarray")
                                n728 = Unbundle By Name(w1761) -> ("Global Position (mm)"=w1759:dbl[])
                                n729 = Replace Array Subset(array=w1759, new element=w1757, index=w1757) -> (w1758:dbl[])
                                n730 = Bundle By Name(cluster=w1761, "Global Position (mm)"=w1758) -> (w1760:T26)
                              }
                            }
                            n731 = Unbundle By Name(w1739) -> ("Switch T/R"=w1748:i16)
                            n732 = Decrement(x=w1748) -> (x-1=w1749:i16)
                            n733 = call "ChooseDualXDCRSettings.vi"("Digitizer Settings in"=w1752, "Switch T/R"=w1748, "Pulser"=w1745, "Motion Settings in"=w1751, "Dual XDCR Settings"=w1742, "Setup Time\nParameters (F)"=FALSE ("Setup Time\nParameters (F)"), "Allow USB R/Ws?"=FALSE) -> ("Digitizer Settings"=w1731:T30, "Motion Settings"=w1754:T26)  [unwired: 18 in, 1 out]
                            n734 = Bundle By Name(cluster=w1731, "Digitizer delay (us)"=w1728, "rf points per line"=w1730, "Additional dig delay (us)"=0.0) -> (w1732:T30)
                          }
                        }
                        n735 = property on="SetDig" class="Bool (strict)"("Value"=FALSE ("SetDig")) -> ()  [unwired: 2 in, 2 out]
                        n736 = Send Notification(notification=w1699, notifier=w1715) -> ()  [unwired: 1 in, 2 out]
                      }
                      event "Set Pulser": Value Change {
                        n737 = event-data() -> ()  [unwired: 1 in, 2 out]
                        n738 = call "SetAllPulsersGUI.vi"("Init Tabor?"=FALSE ("Init?"), "Pulser"=w1770) -> ()  [unwired: 10 in]
                      }
                      event Value Change {
                        n739 = event-data() -> ()  [unwired: 1 in, 1 out]
                        n740 = Unbundle By Name(w1783) -> ("XDCR Settings"=w1782:T2[])
                        n741 = call "Set_Daxsonics_3Pulsers.vi"("Daxsonics Settings"="Daxsonics Settings") -> ()  [unwired: 9 in]
                        n742 = in-place {
                          in-place-border: "Daxsonics Settings" -> [w1791]
                          n743 = in-place-array #5(w1782, w1781) -> (w1790:T2)
                          n744 = Bundle By Name(cluster=w1790, "Daxsonics Settings"=w1791) -> (w1789:T2)
                          n745 = in-place-array #5(w1789) -> (w1780:T2[])  [unwired: 1 out]
                        }
                        n746 = Bundle By Name(cluster=w1783, "XDCR Settings"=w1780) -> (w1779:T1)
                        n747 = global write "SwitchGlobals.vi" "Dual XDCR Settings"(w1779) -> ()
                      }
                      event "Panametrics Settings": Value Change {
                        n748 = event-data() -> ("NewVal"=w1796:T39)  [unwired: 1 in]
                        n749 = case shown="\"Dual Transducer\"" w1794 {
                          tunnel: w1800 -> [w1811 w1816]
                          tunnel: [w1811 w1815] -> w1799
                          tunnel: w1798 -> [_ w1814]
                          tunnel: w1796 -> [w1807 w1813]
                          tunnel: [w1805 w1812] -> w1795
                          frame "Therapy With Scan", Default {
                            n750 = Unbundle By Name(w1807) -> ("ENERGY (uJ)"=w1808:u16, "COARSE ATTENUATION"=w1809:u16, "FINE ATTENUATION"=w1810:u16)
                            n751 = Bundle By Name(cluster=T4 {"ENERGY (uJ)"=0, "DAMPING (Ohm)"=0, "HP FILT (KHz) "=0, "LP FILT (MHz)"=0, "MODE"=0, "PRF (KHz)"=1, "GAIN (db)"=0, "COARSE ATTENUATION"=0, "FINE ATTENUATION"=0} ("Panametrics Settings"), "ENERGY (uJ)"=w1808, "COARSE ATTENUATION"=w1809, "FINE ATTENUATION"=w1810) -> (w1805:T4)
                          }
                          frame "Dual Transducer" {
                            n752 = Unbundle By Name(w1816) -> ("XDCR Settings"=w1818:T2[])
                            n753 = in-place {
                              in-place-border: w1813 -> [w1823]
                              in-place-border: [w1819] -> w1812
                              n754 = in-place-array #6(w1818, w1814) -> (w1821:T2)
                              n755 = Unbundle By Name(w1823) -> ("ENERGY (uJ)"=w1824:u16, "COARSE ATTENUATION"=w1825:u16, "FINE ATTENUATION"=w1826:u16)
                              n756 = Unbundle By Name(w1821) -> ("Panametrics Settings"=w1822:T4)
                              n757 = Bundle By Name(cluster=w1822, "ENERGY (uJ)"=w1824, "COARSE ATTENUATION"=w1825, "FINE ATTENUATION"=w1826) -> (w1819:T4)
                              n758 = Bundle By Name(cluster=w1821, "Panametrics Settings"=w1819) -> (w1820:T2)
                              n759 = in-place-array #6(w1820) -> (w1817:T2[])  [unwired: 1 out]
                            }
                            n760 = Bundle By Name(cluster=w1816, "XDCR Settings"=w1817) -> (w1815:T1)
                            n761 = global write "SwitchGlobals.vi" "Dual XDCR Settings"(w1815) -> ()
                          }
                        }
                        n762 = call "5900PRQuickSet.vi"("VISA resource name"=w1793, "Panametrics Settings"=w1795) -> ("error out"=w1792:errorcluster)  [unwired: 2 in]
                        n763 = property on="error out" class="Clust (strict)"("Value"=w1792) -> ()  [unwired: 2 in, 2 out]
                      }
                      event Value Change {
                        n764 = event-data() -> ()  [unwired: 1 in, 1 out]
                        n765 = Unbundle By Name("JSR Simple") -> ("Pulse Energy Level"=w1836:T8, "Gain (dB)"=w1834:T15, "Pulser Voltage (V)"=w1835:T10)
                        n766 = global read "PulserGlobals.vi" "JSR Settings"() -> (w1838:T5)
                        n767 = Bundle By Name(cluster=w1838, "JSR Pulse Settings.Pulse Energy Level"=w1836, "JSR Receive Settings.Gain (dB)"=w1834, "JSR Pulse Settings.Pulser Voltage (V)"=w1835) -> (w1830:T5)
                        n768 = case shown="\"Dual Transducer\"" w1829 {
                          tunnel: w1831 -> [w1843 w1847]
                          tunnel: [w1843 w1846] -> w1828
                          tunnel: w1832 -> [_ w1845]
                          tunnel: w1830 -> [_ w1844]
                          frame "Therapy With Scan", Default {
                          }
                          frame "Dual Transducer" {
                            n769 = Unbundle By Name(w1847) -> ("XDCR Settings"=w1849:T2[])
                            n770 = in-place {
                              in-place-border: w1844 -> [w1850]
                              n771 = in-place-array #7(w1849, w1845) -> (w1852:T2)
                              n772 = Bundle By Name(cluster=w1852, "JSR Complete"=w1850) -> (w1851:T2)
                              n773 = in-place-array #7(w1851) -> (w1848:T2[])  [unwired: 1 out]
                            }
                            n774 = Bundle By Name(cluster=w1847, "XDCR Settings"=w1848) -> (w1846:T1)
                            n775 = global write "SwitchGlobals.vi" "Dual XDCR Settings"(w1846) -> ()
                          }
                        }
                        n776 = call "JSR SetAll.vi"("JSR Complete"=w1830) -> ("error out"=w1827:errorcluster)  [unwired: 9 in, 1 out]
                        n777 = property on="error out" class="Clust (strict)"("Value"=w1827) -> ()  [unwired: 2 in, 2 out]
                      }
                      event Value Change {
                        n778 = event-data() -> ("OldVal"=w1859:T38)  [unwired: 1 in]
                        n779 = control-ref of="UT340 Controls"() -> (w1855:refnum<vi>)
                        n780 = Not Equal?(x="UT340 Controls", y=w1859) -> (x != y?=w1858:cluster{"PE Gain (dB)":bool, "Voltage":bool})
                        n781 = call "UTEX Simple Send.vi"("UT340 Simple Controls"=w1855, "Read Back Values?"=TRUE, "Changed Values?"=w1858, "UT340 Controls"="UT340 Controls") -> ("error out"=w1853:errorcluster)  [unwired: 7 in]
                        n782 = Unbundle By Name("UT340 Controls") -> ("PE Gain (dB)"=w1860:i16, "Voltage"=w1861:i16)
                        n783 = property on="error out" class="Clust (strict)"("Value"=w1853) -> ()  [unwired: 2 in, 2 out]
                        n784 = global read "PulserGlobals.vi" "UT340 Controls"() -> (w1867:T20)
                        n785 = Bundle By Name(cluster=w1867, "PE Gain (dB)"=w1860, "Voltage"=w1861) -> (w1856:T20)
                        n786 = case shown="\"Dual Transducer\"" w1863 {
                          tunnel: w1864 -> [w1872 w1876]
                          tunnel: [w1872 w1875] -> w1862
                          tunnel: w1865 -> [_ w1874]
                          tunnel: w1856 -> [_ w1873]
                          frame "Therapy With Scan", Default {
                          }
                          frame "Dual Transducer" {
                            n787 = Unbundle By Name(w1876) -> ("XDCR Settings"=w1878:T2[])
                            n788 = in-place {
                              in-place-border: w1873 -> [w1879]
                              n789 = in-place-array #8(w1878, w1874) -> (w1881:T2)
                              n790 = Bundle By Name(cluster=w1881, "UT340 Controls"=w1879) -> (w1880:T2)
                              n791 = in-place-array #8(w1880) -> (w1877:T2[])  [unwired: 1 out]
                            }
                            n792 = Bundle By Name(cluster=w1876, "XDCR Settings"=w1877) -> (w1875:T1)
                            n793 = global write "SwitchGlobals.vi" "Dual XDCR Settings"(w1875) -> ()
                          }
                        }
                      }
                      event "Filter Prams": Value Change {
                        n794 = event-data() -> ("NewVal"=w1884:T40)  [unwired: 1 in]
                        n795 = Unbundle By Name(w1883) -> ("Samp Rate (Hz)"=w1887:dbl)
                        n796 = expression code="x*1E-6"(w1887) -> (w1888:dbl)
                        n797 = case shown="\"Dual Transducer\"" w1882 {
                          tunnel: w1894 -> [_ w1906]
                          tunnel: w1893 -> [_ w1905]
                          tunnel: w1892 -> [_ w1902]
                          tunnel: w1891 -> [w1897 w1901]
                          tunnel: [w1897 w1900] -> w1890
                          tunnel: w1884 -> [_ w1899]
                          tunnel: w1883 -> [_ w1898]
                          frame "Therapy With Scan", Default {
                          }
                          frame "Dual Transducer" {
                            n798 = To Long Integer(number=w1905) -> (32bit integer=w1904:i32)
                            n799 = Increment(x=w1904) -> (x+1=w1903:i32)
                            n800 = call "UpdateDualXDCRSettings.vi"("Digitizer Settings in"=w1898, "Filter Prams"=w1899, "Motion Settings in"=w1906, "Switch T/R"=w1903, "Dual XDCR Settings In"=w1901, "Switch Unit"=w1902) -> ("Dual XDCR Settings"=w1900:T1)  [unwired: 2 in]
                          }
                        }
                        n801 = call "BP FilterCoeffs.vi"("sample rate MHz"=w1888, "Filter Prams"=w1884) -> ("FIR Windowed Coefficients"=w1889:dbl[])  [unwired: 4 in]
                        n802 = Bundle(cluster=w1885, "FIR Windowed Coefficients"=w1889, "Filter Prams"=w1884) -> (w1886:T62)
                      }
                      event "Pause Mode?": Value Change {
                        w1909 = TRUE
                        n803 = event-data() -> ()  [unwired: 1 in, 6 out]
                        n804 = Send Notification(notification=w1909, notifier=w1913) -> ()  [unwired: 1 in, 2 out]
                      }
                      event "Position (mm) (Pt1)": Value Change {
                        n805 = event-data() -> ("OldVal"=w1929:dbl, "NewVal"=w1920:dbl)  [unwired: 1 in]
                        n806 = property on="Position (mm) (Pt2)" class="DigNum (strict)"() -> ("Value"=w1926:dbl)  [unwired: 2 in, 2 out]
                        n807 = Greater?(x=w1920, y=w1926) -> (0:w1927:bool)
                        n808 = case shown="True" w1927 {
                          tunnel: w1926 -> [w1936 _]
                          tunnel: w1920 -> [w1935 w1938]
                          tunnel: [w1936 w1938] -> w1922
                          tunnel: [w1935 w1937] -> w1923
                          tunnel: w1929 -> [_ w1937]
                          frame False {
                          }
                          frame True {
                            n809 = property on="Position (mm) (Pt2)" class="DigNum (strict)"("Value"=w1938) -> ()  [unwired: 2 in, 2 out]
                            n810 = property on="Position (mm) (Pt1)" class="DigNum (strict)"("Value"=w1937) -> ()  [unwired: 2 in, 2 out]
                          }
                        }
                        n811 = Subtract(x=w1923, y=w1922) -> (x-y=w1925:dbl)
                        n812 = Absolute Value(x=w1925) -> (abs(x)=w1918:dbl)
                        n813 = call-poly "ModFractionPoly.vi"("Modulo Fraction"=w1916, "Input"=w1918) -> ("Output"=w1917:dbl)  [unwired: 1 in]
                        n814 = Replace Array Subset(array=w1924, new element=w1917, index=1) -> (w1921:dbl[])
                        n815 = property on="Acquisition Volume (mm)" class="Arr (strict)"("Val(Sgnl)"=w1921) -> ()  [unwired: 2 in, 2 out]
                      }
                      event "Position (mm) (Pt2)": Value Change {
                        n816 = event-data() -> ("NewVal"=w1952:dbl, "OldVal"=w1951:dbl)  [unwired: 1 in]
                        n817 = property on="Position (mm) (Pt1)" class="DigNum (strict)"() -> ("Value"=w1950:dbl)  [unwired: 2 in, 2 out]
                        n818 = Less?(x=w1952, y=w1950) -> (x < y?=w1948:bool)
                        n819 = case shown="True" w1948 {
                          tunnel: w1950 -> [w1958 _]
                          tunnel: w1952 -> [w1959 w1961]
                          tunnel: [w1959 w1961] -> w1946
                          tunnel: [w1958 w1960] -> w1945
                          tunnel: w1951 -> [_ w1960]
                          frame False {
                          }
                          frame True {
                            n820 = property on="Position (mm) (Pt2)" class="DigNum (strict)"("Value"=w1960) -> ()  [unwired: 2 in, 2 out]
                            n821 = property on="Position (mm) (Pt1)" class="DigNum (strict)"("Value"=w1961) -> ()  [unwired: 2 in, 2 out]
                          }
                        }
                        n822 = Subtract(x=w1946, y=w1945) -> (x-y=w1947:dbl)
                        n823 = Absolute Value(x=w1947) -> (abs(x)=w1941:dbl)
                        n824 = call-poly "ModFractionPoly.vi"("Modulo Fraction"=w1939, "Input"=w1941) -> ("Output"=w1940:dbl)  [unwired: 1 in]
                        n825 = Replace Array Subset(array=w1944, new element=w1940, index=1) -> (w1943:dbl[])
                        n826 = property on="Acquisition Volume (mm)" class="Arr (strict)"("Val(Sgnl)"=w1943) -> ()  [unwired: 2 in, 2 out]
                      }
                      event "End Point\nMarker": Value Change {
                        w1966 = T47."Round Nearest" ("Round Method")
                        w1967 = 2 ("Digits past \".\"")
                        n827 = event-data() -> ()  [unwired: 1 in, 1 out]
                        n828 = Decrement(x=w1962) -> (x-1=w1963:i32)
                        n829 = property on="Last End Point" class="DigNum (strict)"() -> ("Value"=w1969:dbl)  [unwired: 2 in, 2 out]
                        n830 = call "FindLocation_SingleAxis.vi"("Axis (0 is X)"=w1963, "Motion Settings"=w1964) -> ("Position (mm) (Abs)"=w1965:dbl)  [unwired: 2 in, 3 out]
                        n831 = call "Decimal Rounding.vi"("Round Method (Nearest)"=w1966, "Digits past \".\" (1)"=w1967, "Input"=w1969) -> ("Output"=w1968:dbl)  [unwired: 8 in]
                        n832 = call "Decimal Rounding.vi"("Round Method (Nearest)"=w1966, "Digits past \".\" (1)"=w1967, "Input"=w1965) -> ("Output"=w1970:dbl)  [unwired: 8 in]
                        n833 = Not Equal?(x=w1970, y=w1968) -> (x != y?=w1973:bool)
                        n834 = case shown="True" w1973 {
                          tunnel: w1965 -> [_ w1982]
                          frame False {
                            n835 = call <vilib>:"Beep.vi"("use system alert? (T)"=FALSE, "duration (msec)"=u32 250, "frequency (Hz)"=u32 1000) -> ()  [unwired: 9 in]
                          }
                          frame True {
                            n836 = flat-sequence {
                              tunnel: [w1987] -> w1984
                              tunnel: [w1986] -> w1983
                              tunnel: w1982 -> [w1985]
                              tunnel: w1984 -> [w2003]
                              tunnel: w1983 -> [w1998]
                              frame #0 {
                                n837 = property on="End Point Counter" class="DigNum (strict)"() -> ("Value"=w1987:u32)  [unwired: 2 in, 2 out]
                                n838 = case shown="0" w1987 {
                                tunnel: w1985 -> [w1988 w1989 w1990]
                                tunnel: [w1988 w1989 w1990] -> w1986
                                frame 0 {
                                n839 = property on="Position (mm) (Pt2)" class="DigNum (strict)"("Value"=w1988) -> ()  [unwired: 2 in, 2 out]
                                }
                                frame 1 {
                                n840 = property on="Position (mm) (Pt1)" class="DigNum (strict)"("Value"=w1989) -> ()  [unwired: 2 in, 2 out]
                                }
                                frame 2, Default {
                                n841 = property on="Position (mm) (Pt2)" class="DigNum (strict)"() -> ("Value"=w1993:dbl)  [unwired: 2 in, 2 out]
                                n842 = property on="Position (mm) (Pt1)" class="DigNum (strict)"() -> ("Value"=w1992:dbl)  [unwired: 2 in, 2 out]
                                n843 = Build Array(w1993, w1992) -> (w1995:dbl[])
                                n844 = call-poly <vilib>:"Mean.vi"("X"=w1995) -> ("mean"=w1994:dbl)  [unwired: 1 out]
                                n845 = Greater?(x=w1990, y=w1994) -> (0:w1991:bool)
                                n846 = case shown="True" w1991 {
                                tunnel: w1990 -> [w1996 w1997]
                                frame False {
                                n847 = property on="Position (mm) (Pt1)" class="DigNum (strict)"("Val(Sgnl)"=w1996) -> ()  [unwired: 2 in, 2 out]
                                }
                                frame True {
                                n848 = property on="Position (mm) (Pt2)" class="DigNum (strict)"("Val(Sgnl)"=w1997) -> ()  [unwired: 2 in, 2 out]
                                }
                                }
                                }
                                }
                              }
                              frame #1 {
                                n849 = Increment(x=w2003) -> (x+1=w2002:u32)
                                n850 = property on="End Point Counter" class="DigNum (strict)"("Value"=w2002) -> ()  [unwired: 2 in, 2 out]
                                n851 = call <vilib>:"Beep.vi"("use system alert? (T)"=FALSE, "duration (msec)"=u32 250, "frequency (Hz)"=u32 2000) -> ()  [unwired: 9 in]
                                "Last End Point" <- w1998
                              }
                            }
                          }
                        }
                        n852 = property on="End Point\nMarker" class="Bool (strict)"("Value"=FALSE ("End Point\nMarker")) -> ()  [unwired: 2 in, 2 out]
                      }
                      event "dB Range": Mouse Leave; "dB Range": Mouse Up {
                        w2013 = 1.0 ("Z Scale.Range:Minor Increment")
                        n853 = event-data() -> ()  [unwired: 1 in, 4 out]
                        n854 = Equal?(x=location."Hawaii", y=w2006) -> (x = y?=w2005:bool)
                        n855 = Select(t=0.0 ("upper limit"), s=w2005, f=-1.5) -> (s? t:f=w2008:dbl)
                        n856 = Unbundle("dB Range") -> (w2015:dbl, w2014:dbl)
                        n857 = In Range and Coerce(upper limit=w2008, x=w2015, lower limit=-80.0) -> (coerced(x)=w2012:dbl)  [unwired: 1 out]
                        n858 = property on="Real Time Image" class="IntGraph (strict)"("ZScale.Maximum"=w2012, "ZScale.Minimum"=w2014, "ZScale.MinorInc"=w2013, "ZScale.Increment"=w2013) -> ()  [unwired: 2 in, 2 out]
                      }
                      event "Center": Value Change {
                        n859 = event-data() -> ()  [unwired: 1 in, 1 out]
                        n860 = Unbundle By Name(w2023) -> ("Distance between\nscan planes (um)"=w2054:sgl, "Steps per mm"=w2039:i32[], "Motion System"=w2024:T27)  [unwired: 1 out]
                        n861 = local read "Position (mm) (Pt1)"() -> (w2062:dbl)
                        n862 = local read "Position (mm) (Pt2)"() -> (w2061:dbl)
                        n863 = To Long Integer(number=w2037) -> (32bit integer=w2033:i32)
                        n864 = Decrement(x=w2037) -> (x-1=w2036:i32)
                        n865 = property on="Axis Tune" class="RadioBtnsControl (strict)"("Val(Sgnl)"=w2036) -> ()  [unwired: 2 in, 2 out]
                        n866 = Max & Min(x=w2062, y=w2061) -> (max(x,y)=w2060:dbl, min(x,y)=w2058:dbl)
                        n867 = Subtract(x=w2060, y=w2058) -> (x-y=w2050:dbl)
                        n868 = expression code="x/1000"(w2054) -> (w2053:sgl)
                        n869 = Divide(x=w2050, y=2) -> (x/y=w2055:dbl)
                        n870 = Decrement(x=w2033) -> (x-1=w2027:i32)
                        n871 = Add(x=w2055, y=w2058) -> (x+y=w2034:dbl)
                        n872 = Divide(x=w2055, y=w2053) -> (x/y=w2044:dbl)
                        n873 = Index Array(array=w2039, index=w2027) -> (element=w2038:i32)
                        n874 = Replace Array Subset(array=w2045, new element=w2050, index=1) -> (w2041:dbl[])
                        n875 = Multiply(x=w2038, y=w2034) -> (x*y=w2057:dbl)
                        n876 = case shown="False" w2035 {
                          tunnel: w2034 -> [w2080 _]
                          tunnel: w2033 -> [w2079 _]
                          tunnel: [w2078 FALSE] -> w2032
                          tunnel: w2031 -> [w2077 _]
                          frame False {
                            w2078 = TRUE
                            n877 = Decrement(x=w2079) -> (x-1=w2076:i32)
                            n878 = property on="Scan Start Pos (mm)" class="Arr (strict)"() -> ("Value"=w2082:dbl[])  [unwired: 2 in, 2 out]
                            n879 = Replace Array Subset(array=w2082, new element=w2080, index=w2076) -> (w2081:dbl[])
                            n880 = property on="Scan Start Pos (mm)" class="Arr (strict)"("Value"=w2081) -> ()  [unwired: 2 in, 2 out]
                            n881 = Send Notification(notification=w2078, notifier=w2077) -> ()  [unwired: 1 in, 2 out]
                          }
                          frame True {
                          }
                        }
                        n882 = call "Force Odd or Even.vi"("Parity (odd)"=enum16{"Odd", "Even"}."Odd" ("Parity"), "input"=w2044) -> ("output"=w2048:i32)
                        n883 = case shown="\"NI 735x\"" w2024 {
                          tunnel: w2057 -> [_ w2069 w2072]
                          tunnel: w2033 -> [_ w2068 w2073]
                          tunnel: [_ w2067 w2075] -> w2030
                          tunnel: w2023 -> [_ w2066 w2071]
                          frame "MM3000", Default {
                          }
                          frame "NI 735x" {
                            n884 = Unbundle By Name(w2066) -> ("Motion Bd ID"=w2065:u8)
                            n885 = call "MoveMotor.vi"("Target Position (0)"=w2069, "Axis or Vector Space"=w2068, "Motion Bd ID"=w2065) -> ("error out"=w2067:errorcluster)  [unwired: 6 in, 2 out]
                          }
                          frame "Galil" {
                            n886 = Decrement(x=w2073) -> (x-1=w2074:i32)
                            n887 = Unbundle By Name(w2071) -> ("GL Ref Out"=w2070:refnum<k7>)
                            n888 = call "GL Set Operation Mode.vi"("position cts (abs/rel)"=w2072, "Axis"=w2074, "Galil.IGalil"=w2070) -> ("error out"=w2075:errorcluster)  [unwired: 6 in, 2 out]
                          }
                        }
                        n889 = property on="Acquisition Volume (mm)" class="Arr (strict)"("Val(Sgnl)"=w2041) -> ()  [unwired: 2 in, 2 out]
                        n890 = call "WaitForMoveComplete.vi"("Motion Settings"=w2023, "Axis to Ignore (x=1)"=w2025, "error in"=w2030, "Ignore Axis?"=TRUE) -> ("error out"=w2029:errorcluster)  [unwired: 2 in]
                        n891 = call "FindLocation_SingleAxis.vi"("error in (no error)"=w2029, "Axis (0 is X)"=w2033, "Motion Settings"=w2023) -> ("error out"=w2026:errorcluster, "Global Position"=w2052:dbl[])  [unwired: 1 in, 2 out]
                        n892 = Bundle By Name(cluster=w2023, "number of scan planes"=w2048, "Global Position (mm)"=w2052) -> (w2056:T26)
                        n893 = property on="Center" class="Bool (strict)"("Value"=TRUE ("Center")) -> ()  [unwired: 2 in, 2 out]
                        n894 = property on="error out" class="Clust (strict)"("Value"=w2026) -> ()  [unwired: 2 in, 2 out]
                        n895 = for {
                          N: 2 -> [_]
                          n896 = call <vilib>:"Beep.vi"("use system alert? (T)"=FALSE, "duration (msec)"=u32 250, "frequency (Hz)"=u32 2000) -> ()  [unwired: 9 in]
                        }
                      }
                      event "Pause Motion": Value Change {
                        n897 = event-data() -> ("NewVal"=w2087:bool)  [unwired: 1 in, 5 out]
                        n898 = case shown="False" w2090 {
                          tunnel: w2095 -> [w2100 _]
                          tunnel: w2089 -> [_ w2126]
                          tunnel: [FALSE w2125] -> w2088
                          tunnel: w2087 -> [w2098 _]
                          frame False {
                            n899 = Unbundle By Name(w2100) -> ("Motion System"=w2099:T27)
                            n900 = case shown="\"NI 735x\"" w2099 {
                              tunnel: w2100 -> [_ w2102 w2107]
                              tunnel: w2098 -> [_ _ w2106]
                              frame "MM3000", Default {
                              }
                              frame "NI 735x" {
                                n901 = disable-structure shown="Disabled" {
                                disable-tunnel: w2102 -> [w2103 _]
                                frame Disabled {
                                n902 = Unbundle By Name(w2103) -> ("Motion Bd ID"=w2105:u8)
                                n903 = call "Pause/Resume Program.flx"("Program (1)"=T52 8, "Board ID"=w2105) -> ()  [unwired: 4 in, 3 out]
                                }
                                frame Enabled {
                                }
                                }
                              }
                              frame "Galil" {
                                n904 = case shown="True" w2106 {
                                tunnel: w2107 -> [w2109 w2120]
                                frame False {
                                # "Resume after BK pause"
                                n905 = Unbundle By Name(w2109) -> ("GL Ref Out"=w2111:refnum<k7>)
                                n906 = call "GL Command Set.vi"("Command"=Command_Menu."BreakPoint", "Value"=-1, "Galil.IGalil"=w2111) -> ()  [unwired: 4 in, 5 out]
                                }
                                frame True {
                                # "Pause"
                                n907 = Unbundle By Name(w2120) -> ("GL Ref Out"=w2119:refnum<k7>)
                                n908 = call "GL Command Set.vi"("Command"=Command_Menu."Current Code Line", "Text Input"="#RAPID", "Galil.IGalil"=w2119) -> ("error out"=w2117:errorcluster, "Response#"=w2114:i32, "ref out"=w2116:refnum<k7>)  [unwired: 4 in, 2 out]
                                n909 = Add(x=w2114, y=5) -> (x+y=w2112:i32)
                                n910 = case shown="1, Default" w2112 {
                                selector: w2112 -> [_ w2121]
                                tunnel: w2117 -> [_ w2124]
                                tunnel: w2116 -> [_ w2123]
                                frame -1 {
                                }
                                frame 1, Default {
                                n911 = call "GL Command Set.vi"("Command"=Command_Menu."BreakPoint", "error in (no error)"=w2124, "Value"=w2121, "Galil.IGalil"=w2123) -> ()  [unwired: 3 in, 5 out]
                                }
                                }
                                }
                                }
                              }
                            }
                          }
                          frame True {
                            w2125 = TRUE
                            n912 = Send Notification(notification=w2125, notifier=w2126) -> ()  [unwired: 1 in, 2 out]
                          }
                        }
                      }
                      event Value Change {
                        w2127 = TRUE
                        n913 = event-data() -> ()  [unwired: 1 in, 6 out]
                        n914 = Bundle By Name(cluster=w2136, "scan pair"="scan pair") -> (w2130:T26)
                        n915 = Send Notification(notification=w2127, notifier=w2128) -> ()  [unwired: 1 in, 2 out]
                      }
                      event "Transducer": Value Change {
                        n916 = event-data() -> ("NewVal"=w2150:u16, "OldVal"=w2148:u16)  [unwired: 1 in]
                        n917 = Decrement(x=w2142) -> (x-1=w2141:i32)
                        n918 = Bundle By Name(cluster=w2149, "Scan Size"=w2146) -> (w2147:T1)
                        n919 = Decrement(x=w2140) -> (x-1=w2139:i32)
                        n920 = Not Equal?(x=w2150, y=w2148) -> (x != y?=w2161:bool)
                        n921 = Unbundle By Name(w2149) -> ("XDCR Offset"=w2154:dbl[])
                        n922 = case shown="True" w2161 {
                          selector: w2161 -> [_ w2278]
                          tunnel: w2158 -> [w2180 w2279]
                          tunnel: w2157 -> [w2177 w2280]
                          tunnel: [w2178 w2280] -> w2160
                          tunnel: w2150 -> [w2176 _]
                          tunnel: [w2179 w2279] -> w2159
                          tunnel: w2156 -> [w2175 _]
                          tunnel: [w2174 w2278] -> w2155
                          tunnel: w2154 -> [w2173 _]
                          tunnel: w2147 -> [w2172 w2277]
                          tunnel: w2148 -> [w2171 _]
                          tunnel: w2153 -> [w2170 _]
                          tunnel: [w2164 w2277] -> w2152
                          tunnel: w2151 -> [w2169 _]
                          tunnel: w2145 -> [w2168 _]
                          tunnel: w2143 -> [w2167 _]
                          tunnel: w2141 -> [w2166 _]
                          tunnel: w2139 -> [w2165 _]
                          tunnel: w2138 -> [w2163 _]
                          frame True {
                            n923 = stacked-sequence {
                              seq-local: [w2182 _ _ _ _ _] -> [_ _ w2203 _ w2246 _]
                              seq-local: [_ w2190 _ _ _ _] -> [_ _ w2200 _ _ _]
                              seq-local: [_ _ w2205 _ _ _] -> [_ _ _ _ w2251 _]
                              tunnel: w2180 -> [w2188 w2195 _ w2219 w2254 _]
                              tunnel: [_ _ _ _ w2255 _] -> w2179
                              tunnel: [_ _ _ _ w2259 _] -> w2178
                              tunnel: w2177 -> [w2189 _ _ _ w2260 _]
                              tunnel: w2176 -> [_ _ _ _ w2256 _]
                              tunnel: w2175 -> [_ _ _ _ _ w2276]
                              tunnel: [_ _ _ _ _ w2275] -> w2174
                              tunnel: w2173 -> [_ _ w2201 _ _ _]
                              tunnel: w2172 -> [w2185 _ _ _ _ _]
                              tunnel: w2171 -> [w2187 _ _ _ _ _]
                              tunnel: w2170 -> [w2186 _ _ _ _ _]
                              tunnel: w2169 -> [_ _ _ _ _ _]
                              tunnel: w2168 -> [_ _ _ _ w2249 _]
                              tunnel: w2167 -> [_ _ _ w2218 w2248 _]
                              tunnel: w2166 -> [_ w2191 _ _ _ _]
                              tunnel: w2165 -> [_ _ w2202 _ w2247 _]
                              tunnel: [w2182 _ _ _ _ _] -> w2164
                              tunnel: w2163 -> [_ _ _ _ _ _]
                              frame #0 {
                                n924 = To Long Integer(number=w2187) -> (32bit integer=w2181:i32)
                                n925 = Increment(x=w2181) -> (x+1=w2184:i32)
                                n926 = property on="Filter Prams" class="Clust (strict)"() -> ("Value"=w2183:T40)  [unwired: 2 in, 2 out]
                                n927 = call "UpdateDualXDCRSettings.vi"("Digitizer Settings in"=w2189, "Filter Prams"=w2183, "Motion Settings in"=w2188, "Switch T/R"=w2184, "Dual XDCR Settings In"=w2185, "Switch Unit"=w2186) -> ("Dual XDCR Settings"=w2182:T1)  [unwired: 2 in]
                              }
                              frame #1 {
                                n928 = property on="Position (mm) (Pt2)" class="DigNum (strict)"() -> ("Value"=w2196:dbl)  [unwired: 2 in, 2 out]
                                n929 = property on="Position (mm) (Pt1)" class="DigNum (strict)"() -> ("Value"=w2197:dbl)  [unwired: 2 in, 2 out]
                                n930 = call "FindLocation.vi"("Motion Settings"=w2195, "Wait for Motion Complete"=FALSE) -> ("location (mm)"=w2192:dbl[])  [unwired: 1 in, 3 out]
                                n931 = Build Array(w2197, w2196) -> (w2199:dbl[])
                                n932 = Index Array(array=w2192, index=w2191) -> (element=w2198:dbl)
                                n933 = call-poly <vilib>:"Mean.vi"("X"=w2199) -> ("mean"=w2193:dbl)  [unwired: 1 out]
                                n934 = Subtract(x=w2198, y=w2193) -> (x-y=w2190:dbl)
                              }
                              frame #2 {
                                n935 = in-place {
                                in-place-border: w2203 -> [w2208]
                                in-place-border: w2200 -> [w2206]
                                n936 = in-place-array #9(w2201, w2202, 2) -> (w2217:dbl, w2209:dbl)
                                n937 = Unbundle By Name(w2208) -> ("XDCR Settings"=w2213:T2[])
                                n938 = Index Array(array=w2213) -> (element #1=w2211:T2, element #2=w2215:T2)  [unwired: 2 in]
                                n939 = Unbundle By Name(w2215) -> ("Image Vertical Offset"=w2216:dbl)
                                n940 = Unbundle By Name(w2211) -> ("Image Vertical Offset"=w2212:dbl)
                                n941 = Add(x=w2206, y=w2217) -> (x+y=w2207:dbl)
                                n942 = Subtract(x=w2209, y=w2212) -> (x-y=w2214:dbl)
                                n943 = Subtract(x=w2214, y=w2216) -> (x-y=w2210:dbl)
                                n944 = in-place-array #9(w2207, w2210) -> (w2205:dbl[])  [unwired: 2 out]
                                }
                              }
                              frame #3 {
                                n945 = case shown="False" w2218 {
                                tunnel: w2219 -> [w2221 _]
                                frame False {
                                n946 = Unbundle By Name(w2221) -> ("Motion System"=w2220:T27)
                                n947 = case shown="\"NI 735x\"" w2220 {
                                tunnel: w2221 -> [_ w2222 w2227]
                                frame "MM3000", Default {
                                }
                                frame "NI 735x" {
                                n948 = disable-structure shown="Disabled" {
                                disable-tunnel: w2222 -> [w2223 _]
                                frame Disabled {
                                n949 = Unbundle By Name(w2223) -> ("Motion Bd ID"=w2225:u8)
                                n950 = call "Pause/Resume Program.flx"("Program (1)"=T52 8, "Board ID"=w2225) -> ()  [unwired: 4 in, 3 out]
                                }
                                frame Enabled {
                                }
                                }
                                }
                                frame "Galil" {
                                n951 = case shown="True" TRUE {
                                tunnel: w2227 -> [w2229 w2240]
                                frame False {
                                # "Resume after BK pause"
                                n952 = Unbundle By Name(w2229) -> ("GL Ref Out"=w2231:refnum<k7>)
                                n953 = call "GL Command Set.vi"("Command"=Command_Menu."BreakPoint", "Value"=-1, "Galil.IGalil"=w2231) -> ()  [unwired: 4 in, 5 out]
                                }
                                frame True {
                                # "Pause"
                                n954 = Unbundle By Name(w2240) -> ("GL Ref Out"=w2239:refnum<k7>)
                                n955 = call "GL Command Set.vi"("Command"=Command_Menu."Current Code Line", "Text Input"="#RAPID", "Galil.IGalil"=w2239) -> ("error out"=w2237:errorcluster, "Response#"=w2234:i32, "ref out"=w2236:refnum<k7>)  [unwired: 4 in, 2 out]
                                n956 = Add(x=w2234, y=5) -> (x+y=w2232:i32)
                                n957 = case shown="1, Default" w2232 {
                                selector: w2232 -> [_ w2241]
                                tunnel: w2237 -> [_ w2244]
                                tunnel: w2236 -> [_ w2243]
                                frame -1 {
                                }
                                frame 1, Default {
                                n958 = call "GL Command Set.vi"("Command"=Command_Menu."BreakPoint", "error in (no error)"=w2244, "Value"=w2241, "Galil.IGalil"=w2243) -> ()  [unwired: 3 in, 5 out]
                                }
                                }
                                }
                                }
                                }
                                }
                                }
                                frame True {
                                }
                                }
                              }
                              frame #4 {
                                n959 = To Long Integer(number=w2256) -> (32bit integer=w2258:i32)
                                n960 = control-ref of="Filter Prams"() -> (w2250:refnum<vi>)
                                n961 = Increment(x=w2258) -> (x+1=w2257:i32)
                                n962 = call "ChooseDualXDCRSettings.vi"("Digitizer Settings in"=w2260, "Switch T/R"=w2257, "Pulser"=w2249, "Motion Settings in"=w2254, "Dual XDCR Settings"=w2246, "Allow USB R/Ws?"=TRUE, "Filter Parameters Ref"=w2250) -> ("Digitizer Settings"=w2259:T30, "Change Polarity"=w2252:i32, "Motion Settings"=w2253:T26)  [unwired: 18 in]
                                n963 = case shown="False" w2248 {
                                tunnel: [w2267 w2274] -> w2255
                                tunnel: w2253 -> [w2266 w2274]
                                tunnel: w2252 -> [w2265 w2272]
                                tunnel: w2251 -> [w2263 w2273]
                                tunnel: w2247 -> [_ w2268]
                                frame False {
                                n964 = call "MultiAxisMove.vi"("Wait For Move Complete"=TRUE, "Position Mode (Rel)"=T48."Relative Position" ("Position Mode (Absolute)"), "Distance to move (mm)"=w2263, "Move Polarity"=w2265, "Motion Settings"=w2266) -> ("error out"=w2261:errorcluster, "Motion Settings Out"=w2267:T26)  [unwired: 4 in, 1 out]
                                n965 = property on="error out" class="Clust (strict)"("Value"=w2261) -> ()  [unwired: 2 in, 2 out]
                                }
                                frame True {
                                n966 = property on="Scan Start Pos (mm)" class="Arr (strict)"() -> ("Value"=w2269:dbl[])  [unwired: 2 in, 2 out]
                                n967 = Multiply(x=w2273, y=w2272) -> (x*y=w2271:dbl[])
                                n968 = Add(x=w2271, y=w2269) -> (x+y=w2270:dbl[])
                                n969 = Index Array(array=w2269, index=w2268) -> ()  [unwired: 1 out]
                                n970 = property on="Scan Start Pos (mm)" class="Arr (strict)"("Value"=w2270) -> ()  [unwired: 2 in, 2 out]
                                }
                                }
                              }
                              frame #5 {
                                w2275 = TRUE
                                n971 = Send Notification(notification=w2275, notifier=w2276) -> ()  [unwired: 1 in, 2 out]
                              }
                            }
                          }
                          frame False {
                          }
                        }
                      }
                      event "FileName Gen": Value Change {
                        n972 = event-data() -> ()  [unwired: 1 in, 1 out]
                        n973 = property on="FileName Gen" class="Bool (strict)"("Value"=FALSE ("FileName Gen")) -> ()  [unwired: 2 in, 2 out]
                        n974 = case shown="\"Hawaii\", \"Stony Brook\"" w2282 {
                          selector: w2282 -> [_ w2290]
                          frame "WCM Main", Default {
                          }
                          frame "Hawaii", "Stony Brook" {
                            n975 = call "PatientSpecificFileNameGen2.vi"("Location"=w2290, "Add to Database"=FALSE ("Auto Increment"), "Auto Increment"=TRUE) -> ("PatientFileName"=w2292:string)  [unwired: 1 in, 1 out]
                            n976 = property on="File Name" class="Str"("Value"=w2292) -> ()  [unwired: 2 in, 2 out]
                          }
                        }
                      }
                      event "File Name": Mouse Down {
                        n977 = event-data() -> ()  [unwired: 1 in, 1 out]
                        n978 = case shown="\"Stony Brook\"" w2295 {
                          selector: w2295 -> [_ w2302]
                          frame "WCM Main", Default {
                          }
                          frame "Stony Brook" {
                            n979 = call "PatientSpecificFileNameGen2.vi"("Location"=w2302, "Add to Database"=FALSE ("Auto Increment"), "Auto Increment"=TRUE) -> ("PatientFileName"=w2304:string)  [unwired: 1 in, 1 out]
                            n980 = property on="File Name" class="Str"("Value"=w2304) -> ()  [unwired: 2 in, 2 out]
                          }
                        }
                      }
                      event "Real Time Image": Scale Range Change {
                        n981 = event-data() -> ("NewRange"=w2310:T70)  [unwired: 1 in]
                        n982 = Unbundle By Name(w2310) -> ("Maximum"=w2308:dbl, "Minimum"=w2307:dbl)
                        n983 = Bundle("Maximum"=w2308, "Minimum"=w2307) -> (w2309:cluster{"Maximum":dbl, "Minimum":dbl})  [unwired: 1 in]
                        n984 = property on="dB Range" class="Slide (strict)"("Value"=w2309) -> ()  [unwired: 2 in, 2 out]
                      }
                      event "Save\nDual Transducer\nSettings": Value Change {
                        n985 = event-data() -> ()  [unwired: 1 in, 6 out]
                        n986 = Default Directory() -> (w2326:path)
                        n987 = Build Path(base path=w2326, name or relative path=path "ScanningControl/Location Specific" ("path to XML document")) -> (appended path=w2323:path)
                        n988 = case shown="\"Stony Brook\"" w2324 {
                          tunnel: [w2339 w2341 w2344] -> w2322
                          tunnel: w2323 -> [w2339 w2342 w2345]
                          frame "WCM Main", Default {
                          }
                          frame "Stony Brook" {
                            n989 = Build Path(base path=w2342, name or relative path=path "StonyBrook" ("path to XML document")) -> (appended path=w2341:path)
                          }
                          frame "Hawaii" {
                            n990 = Build Path(base path=w2345, name or relative path=path "Hawaii" ("path to XML document")) -> (appended path=w2344:path)
                          }
                        }
                        n991 = call "File Dialog"("start path"=w2322, "prompt"="Please choose a file to write the new defaults to", "default name"="DualXDCRSettings.xml", "pattern (all files)"="*.xml") -> ("selected path"=w2329:path, "cancelled"=w2319:bool, "error out"=w2318:errorcluster)  [unwired: 8 in, 1 out]
                        n992 = case shown="False" w2319 {
                          tunnel: w2329 -> [w2338 _]
                          tunnel: w2320 -> [w2337 _]
                          frame False {
                            n993 = global read "SwitchGlobals.vi" "Full Scan Size"() -> (w2335:dbl[])
                            n994 = Bundle By Name(cluster=w2337, "Scan Size"=w2335) -> (w2336:T1)
                            n995 = call "XDCRDefaultWriter.vi"("Dual XDCR Settings"=w2336, "path to XML document"=w2338) -> ()  [unwired: 10 in]
                          }
                          frame True {
                          }
                        }
                        n996 = property on="error out" class="Clust (strict)"("Value"=w2318) -> ()  [unwired: 2 in, 2 out]
                      }
                      event "Re-Load\nDual Transducer\nSettings": Value Change {
                        w2362 = TRUE
                        n997 = event-data() -> ()  [unwired: 1 in, 1 out]
                        n998 = Default Directory() -> (w2358:path)
                        n999 = Build Path(base path=w2358, name or relative path=path "ScanningControl/Location Specific" ("path to XML document")) -> (appended path=w2356:path)
                        n1000 = case shown="\"Hawaii\"" w2354 {
                          tunnel: [w2373 w2375 w2378] -> w2355
                          tunnel: w2356 -> [w2373 w2376 w2379]
                          frame "WCM Main", Default {
                          }
                          frame "Stony Brook" {
                            n1001 = Build Path(base path=w2376, name or relative path=path "StonyBrook" ("path to XML document")) -> (appended path=w2375:path)
                          }
                          frame "Hawaii" {
                            n1002 = Build Path(base path=w2379, name or relative path=path "Hawaii" ("path to XML document")) -> (appended path=w2378:path)
                          }
                        }
                        n1003 = call "File Dialog2"("start path"=w2355, "prompt"="Please choose a file to load the defaults from", "default name"="DualXDCRSettings.xml", "pattern (all files)"="*.xml") -> ("selected path"=w2361:path, "cancelled"=w2350:bool, "error out"=w2347:errorcluster)  [unwired: 8 in, 1 out]
                        n1004 = case shown="True" w2350 {
                          tunnel: w2361 -> [w2370 _]
                          tunnel: [w2369 w2372] -> w2352
                          tunnel: [w2368 w2371] -> w2351
                          tunnel: w2349 -> [_ w2372]
                          tunnel: w2348 -> [_ w2371]
                          frame False {
                            n1005 = call "XDCRDefaultReader.vi"("path to XML document"=w2370) -> ("Dual XDCR Settings"=w2368:T1)  [unwired: 10 in]
                            n1006 = Unbundle By Name(w2368) -> ("Scan Size"=w2369:dbl[])
                            n1007 = global write "SwitchGlobals.vi" "Full Scan Size"(w2369) -> ()
                          }
                          frame True {
                          }
                        }
                        n1008 = Send Notification(notification=w2362, notifier=w2363) -> ()  [unwired: 1 in, 2 out]
                        n1009 = property on="error out" class="Clust (strict)"("Value"=w2347) -> ()  [unwired: 2 in, 2 out]
                      }
                      event "Scan": Value Change {
                        n1010 = event-data() -> ()  [unwired: 1 in, 1 out]
                        n1011 = case shown="\"Dual Transducer\"" w2382 {
                          selector: w2382 -> [_ w2412]
                          tunnel: w2400 -> [_ w2428]
                          tunnel: w2399 -> [w2407 w2427]
                          tunnel: [w2407 w2426] -> w2398
                          tunnel: w2397 -> [w2406 w2425]
                          tunnel: w2396 -> [w2408 w2424]
                          tunnel: [w2406 w2423] -> w2395
                          tunnel: w2394 -> [w2409 w2422]
                          tunnel: [w2409 w2421] -> w2393
                          tunnel: [w2408 w2420] -> w2392
                          tunnel: [T53."Left Button" ("Which Button?") w2419] -> w2390
                          tunnel: [T25."Transducer 1" ("Dual XDCR Mode") w2418] -> w2389
                          tunnel: w2388 -> [_ w2417]
                          tunnel: w2386 -> [_ w2416]
                          tunnel: w2385 -> [_ w2415]
                          tunnel: w2384 -> [_ w2414]
                          tunnel: w2383 -> [_ w2413]
                          tunnel: w2381 -> [_ w2411]
                          tunnel: w2380 -> [_ w2410]
                          frame "M scan", Default {
                          }
                          frame "Dual Transducer" {
                            n1012 = stacked-sequence {
                              tunnel: w2428 -> [_ w2469 w2481]
                              tunnel: w2427 -> [_ _ w2473]
                              tunnel: [_ _ w2472] -> w2426
                              tunnel: w2425 -> [_ w2463 w2480]
                              tunnel: w2424 -> [w2430 _ w2470]
                              tunnel: w2422 -> [_ _ w2482]
                              tunnel: [_ _ w2479] -> w2423
                              tunnel: [_ _ w2478] -> w2421
                              tunnel: [_ _ w2477] -> w2420
                              tunnel: [_ w2468 _] -> w2419
                              tunnel: [_ w2467 _] -> w2418
                              tunnel: w2417 -> [_ _ w2476]
                              tunnel: w2412 -> [_ _ w2475]
                              tunnel: w2416 -> [_ _ _]
                              tunnel: w2415 -> [w2435 _ _]
                              tunnel: w2414 -> [_ _ _]
                              tunnel: w2413 -> [_ _ _]
                              tunnel: w2411 -> [_ w2466 _]
                              tunnel: w2410 -> [_ _ _]
                              frame #0 {
                                n1013 = Unbundle By Name(w2430) -> ("Steps per mm"=w2438:i32[], "Motion System"=w2429:T27)
                                n1014 = property on="Position (mm) (Pt1)" class="DigNum (strict)"() -> ("Value"=w2441:dbl)  [unwired: 2 in, 2 out]
                                n1015 = property on="Position (mm) (Pt2)" class="DigNum (strict)"() -> ("Value"=w2440:dbl)  [unwired: 2 in, 2 out]
                                n1016 = Decrement(x=w2435) -> (x-1=w2432:i32)
                                n1017 = Index Array(array=w2438, index=w2432) -> (element=w2437:i32)
                                n1018 = Build Array(w2441, w2440) -> (w2439:dbl[])
                                n1019 = call-poly <vilib>:"Mean.vi"("X"=w2439) -> ("mean"=w2431:dbl)  [unwired: 1 out]
                                n1020 = property on="Scan Start Pos (mm)" class="Arr (strict)"() -> ("Value"=w2434:dbl[])  [unwired: 2 in, 2 out]
                                n1021 = Multiply(x=w2431, y=w2437) -> (x*y=w2436:dbl)
                                n1022 = case shown="\"NI 735x\"" w2429 {
                                tunnel: w2436 -> [_ w2444 w2456]
                                tunnel: w2435 -> [_ w2443 w2459]
                                tunnel: w2430 -> [_ w2442 w2462]
                                frame "MM3000", Default {
                                }
                                frame "NI 735x" {
                                n1023 = disable-structure shown="Disabled" {
                                disable-tunnel: w2444 -> [w2449 _]
                                disable-tunnel: w2443 -> [w2447 _]
                                disable-tunnel: w2442 -> [w2446 _]
                                frame Disabled {
                                n1024 = Unbundle By Name(w2446) -> ("Motion Bd ID"=w2445:u8)
                                n1025 = call <vilib>:"Set Operation Mode.flx"("Position Mode (Absolute)"=T48."Absolute Position", "Axis or Vector Space"=w2447, "Board ID"=w2445) -> ("error out"=w2450:errorcluster, "Resource Output"=w2452:T56, "Bd ID Out"=w2451:T54)  [unwired: 3 in]
                                n1026 = call <vilib>:"Load Target Position.flx"("Target Position (0)"=w2449, "error in (no error)"=w2450, "Axis"=w2452, "Board ID"=w2451) -> ("error out"=w2454:errorcluster, "Resource Output"=w2455:T56, "Bd ID Out"=w2453:T54)  [unwired: 3 in]
                                n1027 = call-poly <vilib>:"Start Motion.flx"("error in (no error)"=w2454, "Axis or Vector Space"=w2455, "Board ID"=w2453) -> ()  [unwired: 3 in, 3 out]
                                }
                                frame Enabled {
                                }
                                }
                                }
                                frame "Galil" {
                                n1028 = Unbundle By Name(w2462) -> ("GL Ref Out"=w2460:refnum<k7>)
                                n1029 = Decrement(x=w2459) -> (x-1=w2458:i32)
                                n1030 = call "GL Set Operation Mode.vi"("position cts (abs/rel)"=w2456, "Position Mode (Absolute)"=T48."Absolute Position", "Start Now?"=TRUE, "Axis"=w2458, "Galil.IGalil"=w2460) -> ()  [unwired: 4 in, 3 out]
                                }
                                }
                                n1031 = Replace Array Subset(array=w2434, new element=w2431, index=w2432) -> (w2433:dbl[])
                                n1032 = property on="Scan Start Pos (mm)" class="Arr (strict)"("Value"=w2433) -> ()  [unwired: 2 in, 2 out]
                              }
                              frame #1 {
                                n1033 = Equal?(x=location."Stony Brook", y=w2466) -> (x = y?=w2465:bool)
                                n1034 = call "DualXDCRUserPrompt.vi"("Dual XDCR Settings"=w2463, "Current XDCR"=w2469, "Auto Dual?"=w2465) -> ("Which Button?"=w2468:T53, "Dual XDCR Mode"=w2467:T25)  [unwired: 7 in]
                              }
                              frame #2 {
                                n1035 = call-poly "ModFractionPoly.vi"("Round Method (Nearest)"=T47."Round to +INF", "Modulo Fraction"=0.5, "Input"=w2473) -> ("Output"=w2472:dbl[])
                                n1036 = Bundle By Name(cluster=w2480, "Scan Size"=w2472) -> (w2479:T1)
                                n1037 = case shown="\"Dual Transducer\"" w2475 {
                                tunnel: w2470 -> [w2483 w2495]
                                tunnel: w2482 -> [w2484 w2494]
                                tunnel: w2481 -> [_ w2493]
                                tunnel: w2479 -> [_ w2492]
                                tunnel: [w2484 w2491] -> w2478
                                tunnel: [w2483 w2490] -> w2477
                                tunnel: w2476 -> [_ w2485]
                                frame "Therapy With Scan", Default {
                                }
                                frame "Dual Transducer" {
                                n1038 = To Unsigned Long Integer(number=w2493) -> (unsigned 32bit integer=w2488:u32)
                                n1039 = Increment(x=w2488) -> (x+1=w2487:u32)
                                n1040 = call "ChooseDualXDCRSettings.vi"("Digitizer Settings in"=w2494, "Switch T/R"=w2487, "Pulser"=w2485, "Motion Settings in"=w2495, "Dual XDCR Settings"=w2492, "Setup Time\nParameters (F)"=FALSE ("Setup Time\nParameters (F)"), "Allow USB R/Ws?"=FALSE) -> ("Digitizer Settings"=w2491:T30, "Motion Settings"=w2490:T26)  [unwired: 18 in, 1 out]
                                }
                                }
                              }
                            }
                          }
                        }
                        "Dual XDCR Mode" <- w2389
                        n1041 = property on="Scan" class="Bool (strict)"("Value"=FALSE ("Run Dual Scan")) -> ()  [unwired: 2 in, 2 out]
                        n1042 = case shown="\"Left Button\", Default" w2390 {
                          tunnel: w2402 -> [_ w2498]
                          tunnel: [FALSE w2497] -> w2391
                          frame "Window Close" {
                          }
                          frame "Left Button", Default {
                            w2497 = TRUE
                            n1043 = Send Notification(notification=w2497, notifier=w2498) -> ()  [unwired: 1 in, 2 out]
                          }
                        }
                      }
                      event "Exit": Value Change {
                        w2508 = TRUE
                        n1044 = event-data() -> ()  [unwired: 1 in, 1 out]
                        n1045 = case shown="\"WCM Main\", Default" w2501 {
                          tunnel: w2503 -> [w2512 w2516]
                          tunnel: [w2512 w2514] -> w2502
                          frame "WCM Main", Default {
                          }
                          frame "Hawaii", "Stony Brook" {
                            n1046 = call-poly "ModFractionPoly.vi"("Round Method (Nearest)"=T47."Round to +INF", "Modulo Fraction"=0.5, "Input"=w2516) -> ("Output"=w2514:dbl[])
                          }
                        }
                        n1047 = Send Notification(notification=w2508, notifier=w2510) -> ()  [unwired: 1 in, 2 out]
                        n1048 = property on="Exit" class="Bool (strict)"("Value"=FALSE ("stop")) -> ()  [unwired: 2 in, 2 out]
                        n1049 = property on="Dual XDCR Mode" class="Enum (strict)"("Value"=T25."Exit" ("Dual XDCR Mode")) -> ()  [unwired: 2 in, 2 out]
                      }
                    }
                  }
                  n1050 = while {
                    tunnel: w954 -> [w2541]
                    tunnel: w961 -> [w2529]
                    tunnel: w943 -> [w2528]
                    tunnel: w956 -> [w2534]
                    tunnel: [w2531] -> w955
                    tunnel: w942 -> [w2530]
                    tunnel: w937 -> [w2523]
                    tunnel: w928 -> [w2521]
                    tunnel: w933 -> [w2519]
                    shift-right: [w2517] -> w929
                    shift-left: w930 -> [w2518]
                    stop <- w2533 continue-if-true
                    # "Slightly faster version to read data"
                    # "Get and display data"
                    n1051 = Select(t=sgl 0.6, s=w2521, f=sgl 10.0 ("DigTimeOut")) -> (s? t:f=w2522:sgl)
                    n1052 = call "Rapid Read.vi"("AlazarCluster"=w2529, "Forward?"=w2518, "Motion Settings"=w2530, "Digitizer Settings"=w2528, "Location"=w2523, "Pause?"=w2519, "DigTimeOut"=w2522) -> ("gain"=w2539:dbl, "Array"=w2526:i16[][], "Reverse?"=w2524:bool, "dig error"=w2536:bool, "gain 2 Ch"=w2538:dbl, "error out"=w2525:errorcluster)  [unwired: 3 in]
                    n1053 = local write "error out"(w2525) -> ()
                    n1054 = Not(x=w2524) -> (.not. x?=w2537:bool)
                    n1055 = case shown="True" w2524 {
                      tunnel: w2526 -> [w2542 w2544]
                      tunnel: [w2542 w2543] -> w2527
                      frame False {
                      }
                      frame True {
                        n1056 = call "ReverseData.vi"("Array in"=w2544) -> ("Array out"=w2543:i16[][])
                      }
                    }
                    n1057 = Wait on Notification(notifier=w2534, timeout in ms (-1)=10) -> (notifier out=w2531:refnum<notifier>, timed out?=w2533:bool)  [unwired: 2 in, 2 out]
                    n1058 = Bundle("gain"=w2539, w2537, "Array out"=w2527, "gain 2 Ch"=w2538, "dig error"=w2536) -> (w2540:T71)  [unwired: 1 out]
                    n1059 = Lossy Enqueue Element(queue=w2541, element=w2540) -> ()  [unwired: 1 in, 4 out]
                    n1060 = Not(x=w2518) -> (.not. x?=w2517:bool)
                  }
                  n1061 = Release Notifier(notifier=w955) -> ()  [unwired: 2 in, 3 out]
                }
                frame #2 {
                  # "Hack to step through tabor settings."
                  n1062 = Unbundle By Name(w2545) -> ("Main Digitizer"=w2546:T31)
                  n1063 = case shown="\"AlazarTech\"" w2546 {
                    tunnel: w2547 -> [_ w2548]
                    frame "Acqiris Digitizer", Default {
                    }
                    frame "AlazarTech" {
                      # "Stop Alazar"
                      n1064 = Unbundle By Name(w2548) -> ("data value reference"=w2549:refnum<data-value>)
                      n1065 = Delete Data Value Reference(data value reference=w2549) -> ()  [unwired: 1 in, 2 out]
                    }
                  }
                }
              }
            }
          }
          frame #7 {
            n1066 = Release Queue(queue=w2552) -> ()  [unwired: 2 in, 3 out]
            n1067 = local write "BMP?"(FALSE) -> ()
            n1068 = local write "Exit"(FALSE ("stop out")) -> ()
            n1069 = Unbundle By Name(w2551) -> ("Main Digitizer"=w2553:T31)
            n1070 = case shown="\"AlazarTech\"" w2553 {
              tunnel: w2551 -> [w2558 _ w2565]
              frame "NI Digitizer" {
                n1071 = Unbundle By Name(w2558) -> ("Digitizer ID Cluster.NI Instr Handles"=w2557:refnum<k15>[])
                n1072 = for {
                  tunnel: w2557 -> [w2559] mode=indexing
                  n1073 = call <instrlib>:"niScope Abort.vi"("instrument handle"=w2559) -> ()  [unwired: 13 in, 2 out]
                }
              }
              frame "Acqiris Digitizer", Default {
              }
              frame "AlazarTech" {
                n1074 = Unbundle By Name(w2565) -> ("Digitizer ID Cluster.Acqiris/Alazar/SP ID"=w2564:u32[])
                n1075 = Index Array(array=w2564) -> (element=w2563:u32)  [unwired: 1 in]
                n1076 = call "AlazarAbortAsyncRead.vi"("Handle"=w2563) -> ("Handle"=w2562:u64, "error out"=w2561:errorcluster)  [unwired: 1 in, 1 out]
                n1077 = call "AlazarConfigureAuxIO.vi"("error in (no error)"=w2561, "Mode"=u32 13, "Handle"=w2562) -> ()  [unwired: 1 in, 3 out]
              }
            }
            n1078 = case shown="\"Hawaii\", Default" w2556 {
              tunnel: w2550 -> [w2567 _]
              frame "Hawaii", Default {
                w2568 = u16 1 items=["Function Gen Input", "Motion Trig", "Internal RT Motion Trig", "Internal CTR 1 Output"] ("Trig Source")
                # "turn off real time trig"
                n1079 = Unbundle By Name(w2567) -> ("GL Ref Out"=w2566:refnum<k7>)
                n1080 = call "RouteTrigSource.vi"("Galil.IGalil"=w2566, "Trig Source"=w2568) -> ()  [unwired: 9 in, 1 out]
              }
              frame "UHI Allen", "CUMC RT" {
              }
            }
          }
          frame #8 {
            n1081 = Unbundle By Name(w2571) -> ("Motion System"=w2578:T27)
            n1082 = Unbundle By Name(w2577) -> ("Dig Config"=w2581:T32)
            n1083 = case shown="\"NI 735x\", Default" w2578 {
              selector: w2578 -> [_ w2583]
              tunnel: w2575 -> [_ w2589]
              tunnel: w2574 -> [_ w2588]
              tunnel: w2571 -> [w2582 w2587]
              tunnel: w2573 -> [_ w2586]
              tunnel: w2572 -> [_ w2585]
              tunnel: [w2582 w2584] -> w2570
              frame "No Motion Card" {
              }
              frame "NI 735x", Default {
                n1084 = case shown="False" w2589 {
                  tunnel: w2588 -> [_ w2604]
                  tunnel: w2587 -> [w2591 w2603]
                  tunnel: w2586 -> [_ w2602]
                  tunnel: w2585 -> [_ w2601]
                  tunnel: [w2591 w2600] -> w2584
                  tunnel: w2583 -> [w2590 _]
                  frame False {
                    n1085 = case shown="\"NI 735x\"" w2590 {
                      tunnel: w2591 -> [_ w2592 w2599]
                      frame "MM3000", Default {
                      }
                      frame "NI 735x" {
                        n1086 = disable-structure shown="Disabled" {
                          disable-tunnel: w2592 -> [w2594 _]
                          frame Disabled {
                            n1087 = Unbundle By Name(w2594) -> ("Motion Bd ID"=w2593:u8)
                            n1088 = call <vilib>:"Stop Program.flx"("Program (1)"=T52 8, "Board ID"=w2593) -> ()  [unwired: 1 in, 6 out]
                          }
                          frame Enabled {
                          }
                        }
                      }
                      frame "Galil" {
                        n1089 = Unbundle By Name(w2599) -> ("GL Ref Out"=w2598:refnum<k7>)
                        n1090 = call "GL Command Set.vi"("Command"=Command_Menu."Halt Execute", "Value"=-1, "Galil.IGalil"=w2598) -> ()  [unwired: 4 in, 5 out]
                      }
                    }
                  }
                  frame True {
                    n1091 = case shown="False" w2604 {
                      tunnel: w2603 -> [w2610 w2626]
                      tunnel: w2601 -> [w2612 _]
                      tunnel: w2602 -> [w2608 _]
                      tunnel: [w2605 w2625] -> w2600
                      frame False {
                        n1092 = property on="Dual XDCR \nHome (mm)" class="Arr (strict)"() -> ("Value"=w2611:dbl[])  [unwired: 2 in, 2 out]
                        n1093 = case shown="\"Real-Time Scan\", Default" w2612 {
                          tunnel: [w2619 w2624] -> w2607
                          tunnel: w2611 -> [w2620 w2624]
                          tunnel: w2608 -> [w2622 _]
                          tunnel: w2610 -> [w2618 w2623]
                          tunnel: [w2621 w2623] -> w2609
                          frame "Real-Time Scan", Default {
                            n1094 = call "FindLocation.vi"("Motion Settings"=w2618) -> ("Motion Settings Out"=w2621:T26, "location (mm)"=w2617:dbl[])  [unwired: 2 in, 2 out]
                            n1095 = Decrement(x=w2622) -> (x-1=w2615:i32)
                            n1096 = Index Array(array=w2620, index=w2615) -> (element=w2616:dbl)
                            n1097 = Replace Array Subset(array=w2617, new element=w2616, index=w2615) -> (w2619:dbl[])
                          }
                          frame "Dual Transducer" {
                          }
                        }
                        n1098 = call "MultiAxisMove.vi"("Find Location"=TRUE, "Wait For Move Complete"=TRUE, "Position Mode (Rel)"=T48."Absolute Position" ("Position Mode (Absolute)"), "Distance to move (mm)"=w2607, "Motion Settings"=w2609) -> ("Motion Settings Out"=w2605:T26)  [unwired: 4 in, 2 out]
                      }
                      frame True {
                        n1099 = call "FindLocation.vi"("Motion Settings"=w2626) -> ("Motion Settings Out"=w2625:T26)  [unwired: 2 in, 3 out]
                      }
                    }
                  }
                }
              }
            }
            n1100 = case shown="\"5-CH pulser w/ ann array\", \"5-pass style ann array\"" w2581 {
              tunnel: w2580 -> [_ w2627]
              frame "Single channel", Default {
              }
              frame "5-CH pulser w/ ann array", "5-pass style ann array" {
                n1101 = for {
                  tunnel: w2627 -> [w2628] mode=indexing
                  n1102 = call <vilib>:"DAQmx Stop Task.vi"("task/channels in"=w2628) -> ("task out"=w2630:refnum<k21>, "error out"=w2629:errorcluster)  [unwired: 13 in]
                  n1103 = call <vilib>:"DAQmx Clear Task.vi"("task in"=w2630, "error in"=w2629) -> ()  [unwired: 13 in, 1 out]
                }
              }
            }
            n1104 = call "NIClearErrors.vi"("Motion Settings"=w2570) -> ("Motion Settings Out"=w2569:T26)  [unwired: 8 in, 2 out]
            "File Name Out" <- "File Name"
          }
        }
      }
    }
  }
  "Digitizer Settings Out" <- w34
  "error out" <- w33
  "Dual XDCR Settings Out" <- w11
  n1105 = To Word Integer(number=w8) -> (16bit integer=w7:i16)
  n1106 = case shown="True" w17 {
    tunnel: w29 -> [w2631 w2633]
    tunnel: [w2631 w2632] -> w28
    frame False {
    }
    frame True {
      n1107 = call "NI_Stop Program and Reset Pos.vi"("return to start"="return to start", "Program ID"=u8 8, "Motion Settings In"=w2633) -> ("Motion Settings"=w2632:T26)  [unwired: 8 in]
    }
  }
  n1108 = Increment(x=w7) -> (x+1=w19:i16)
  n1109 = Bundle By Name(cluster=w20, "Switch T/R"=w19) -> (→"Ann Array Params Out":T22)
  n1110 = call "FindLocation.vi"("Motion Settings"=w28) -> ("Motion Settings Out"=w3:T26)  [unwired: 2 in, 3 out]
  n1111 = call "NIClearErrors.vi"("Motion Settings"=w3) -> ("Motion Settings Out"=→"Motion Settings Out":T26)  [unwired: 8 in, 2 out]
